vi "Maintenance4Ch.vi"() -> ()   [LabVIEW 2020]
doc: "Maintanence VI for FLS imaging system.\n[Covers: REQ9]\n[Covers: REQ10]"
uses:
  SubVI/DigitizerConfiguration/FLImDAQ.ctl
  <instrlib>/niScope/Controls/niScope trigger source.ctl
  SubVI/LabJack/LJ Pin Setting.ctl
  <vilib>/addons/control/pid/autopid.llb/PID autotuning parameters.ctl
  LaguerreDeconLib/DeconEngineClass/LaguerreDeconEngineClass.lvclass/LaguerreDeconEngineClass.ctl
  <vilib>/Utility/error.llb/DialogType.ctl
  <vilib>/event_ctls.llb/usereventprio.ctl
  <vilib>/Utility/miscctls.llb/LVRowAndColumnTypeDef.ctl
  <vilib>/Utility/miscctls.llb/LVMinMaxIncTypeDef.ctl
  SubVI/APD/APDClass.lvclass
  SubVI/APD/GainData.ctl
  SubVI/APD/iRFData.ctl
  <vilib>/Analysis/baseanly.llb/Mean (DBL).vi
  SubVI/GlobalVariables.vi
  <vilib>/addons/control/pid/autopid.llb/PID Online Autotuning (Step Closed Loop).vi
  <vilib>/addons/control/pid/pid.llb/PID Advanced (DBL).vi
  <instrlib>/niScope/Acquire/Fetch/niScope Multi Fetch Binary 16.vi
  <vilib>/Instr/_visa.llb/VISA Configure Serial Port (Instr).vi
  <userlib>/_OpenG.lib/file/file.llb/openg_file.lvlib
  <userlib>/_OpenG.lib/time/time.llb/openg_time.lvlib
  <vilib>/Analysis/NI_AALBase.lvlib
  LaguerreDeconLib/DeconEngineClass/LaguerreDeconEngineClass.lvclass
  <vilib>/Utility/miscctls.llb/LVPointTypeDef.ctl
  <vilib>/addons/control/pid/NI_PID_autopid.lvlib
  <vilib>/addons/control/pid/NI_PID_pid.lvlib
panel:
  in  "Duty Cycle (%)":u32=50
  in  "AB Rep Rate":u16 caption="Rep Rate" max=1000 step=1 format="%.0dHz"
  in  "Current":dbl=1.0 min=1.0 max=63.0 step=1.0 format="%#.1fA"
  out "GainIndicator":dbl caption="Gain"
  out "Noise\n(std of DC)":dbl format="%0.6f"
  in  "BG flag?":bool
  out "DC":dbl format="%0.2f"
  out "Amplitude":dbl
  in  "Gain High":dbl max=4.5
  in  "Gain low":dbl=3.0
  in  "Step":dbl=0.1
  in  "Num WF to acquire":u64=18446744073709551615
  in  "Channel":enum32{"Ch1", "Ch2", "Ch3", "Ch4"}(radio)
  in  "Task":enum32{"iRFAndGain", "Alignment"}(radio)
  in  "Aiming beam toggle":bool caption="445nm 15Hz"
  in  "Laser Rep Rate":u16=120 caption="Rep Rate" min=5 max=4000 step=1 format="%.0dHz"
  in  "355nm Laser toggle":bool caption="355nm 460Hz"
  out "appended path":path
  out "Current State":string
  out "WF max value":dbl
  out "Disclamer":picture
  out "Calibration #":i8
  out "BG #":i8
  in  "TCP Connect":bool
  out "Help":string
  in  "Auto gain":bool=TRUE
  out "Run #":i8
  in  "StopButton":bool caption="Stop"
  out "System Status:":bool
  in  "StartButton":bool caption="Start"
  in  "Ctrl V":dbl=0.05 min=0.0 max=5.5 step=0.1 format="%#.3f"
  out "System Hardware Connection Status":T1
  out "Waveform (no average)":dbl[](graph)
  in  "Tab Control":T2(tab)
  out "Ch1 Max CtrlV":dbl
  out "Ch1 iRF Graph":dbl[][](graph)
  out "Ch1 Gain":cluster{"CtrlV":dbl[], "Gain":dbl[]}(graph)
  out "Serial Number Ch1":string caption="Serial Number"
  out "DateTimeCh1":string caption="DateTime"
  out "Ch2 Gain":cluster{"CtrlV":dbl[], "Gain":dbl[]}(graph)
  out "Ch2 iRF Graph":dbl[][](graph)
  out "Ch2 Max CtrlV":dbl
  out "Serial Number Ch2":string caption="Serial Number"
  out "DateTimeCh2":string caption="DateTime"
  out "Ch3 iRF Graph":dbl[][](graph)
  out "Ch3 Gain":cluster{"CtrlV":dbl[], "Gain":dbl[]}(graph)
  out "Serial Number Ch3":string caption="Serial Number"
  out "Ch3 Max CtrlV":dbl
  out "DateTimeCh3":string caption="DateTime"
  out "Ch4 iRF Graph":dbl[][](graph)
  out "Ch4 Gain":cluster{"CtrlV":dbl[], "Gain":dbl[]}(graph)
  out "Serial Number Ch4":string caption="Serial Number"
  out "Ch4 Max CtrlV":dbl
  out "DateTimeCh4":string caption="DateTime"
  out "display loop timing(ms)":u32
  out "Aquisition loop timing(ms)":u32
  out "DisplayLoop":i32
  out "processing loop":i32
  out "processing loop timing(ms)":dbl
  out "laser EM lamp V":dbl format="%0.6f"
  out "aquisition loop Error Out":errorcluster
  out "Aq Loop?":bool
  out "processing Error Out":errorcluster
  out "Triggering:Trigger Delay":dbl
  out "Foot Pedal":bool
  out "LJ Pinout":T3={"Ch1 Bias"="DAC0", "Ch2 Bias"="DAC1", "Ch3 Bias"="DAC2", "Ch4 Bias"="DAC0", "355 PWM"="FIO0", "AimingBeam PWM"="FIO2", "Laser Ready"="FIO3", "Interlock"="FIO1", "Laser Start/Stop"="FIO1", "Red LED"="FIO1", "Green LED"="DIO3", "Foot Pedal"="DIO15"}
  out "FLImDAQ":T4={"Digitizer 1"="", "Digitizer 2"="", "Channel"=enum."Channel 0", "trigger source"="VAL_EXTERNAL", "trigger level"=0.5, "trigger delay"=1.35e-07, "min sample rate"=12500000000.0, "min record length"=2500, "vertical range"=1.0, "vertical offset"=-0.25, "Waveform to Avg"=2000} caption="FLIm DAQ Configuration" {"trigger delay" format="%^#.4e"; "trigger level" min=0.0 max=3.5 step=0.5 format="%.2f"; "vertical offset" format="%.4f"; "vertical range" format="%.2f"; "min sample rate" format="%#.2p"}
  out "Dig1 Temp":dbl
  out "Dig2 Temp":dbl
  in  "Sys Reconfig":bool
  out "Fetch Record #":i32
  out "Record Backlog":i32
  out "Fetch:Records Done":i32
  out "dt (s)":dbl format="%#_6p"
  out "Fetch:Records Done 2":i32
  in  "SaveData?":bool
  out "data Size":i32[](array[numeric])
  out "numWFInQ":i32
  in  "Clear WF Chart History":bool
  out "Waveform Chart":dbl(graph)
  in  "SaveiRFData":bool
  out "iRFDataTable":string[][](table)
  in  "SetIRFCtrlV":bool
  in  "ClearIRFData":bool
  in  "AcquireIRF":bool
  out "iRFInstSting":string="To aquire gain data, please start data aquisition! \nPlace blue (Ch1&2) or Green(Ch3) Chroma slide as close as possible to the fiber port! \nPlease remove channel 3 bandpass filter as well!"
  out "iRFSigInRange":bool caption="Signal  In Range?"
  out "Current iRF":dbl[](graph)
  out "iRFCtrlV":dbl[](array[numeric])
  in  "SaveGainData":bool
  out "GainInstSting":string="To aquire gain data, please start data aquisition! \nPlace blue (Ch1&2) or Green(Ch3) Chroma slide as close as possible to the fiber port! \nPlease remove channel 3 bandpass filter as well!"
  in  "ClearGainData":bool
  out "Gain":dbl[](array[numeric])
  in  "ComputeGain":bool
  out "Int Corr AUC":dbl[](array[numeric])
  out "AUC Std":dbl[](array[numeric])
  out "GainSigInRange":bool caption="Signal  In Range?"
  in  "AcquireGain":bool
  out "GainDataTable":string[][](table)
  out "Intensity Factor":dbl[](array[numeric])
  out "AUC":dbl[](array[numeric])
  out "Ctrl V":dbl[](array[numeric])
  out "XY Graph":cluster{"Ctrl V":dbl[], dbl[]}(graph)
  in  "Ch4 PID gains":T6={"proportional gain (Kc)"=0.5, "integral time (Ti, min)"=0.0003, "derivative time (Td, min)"=1e-05} {"derivative time (Td, min)" format="%.6f"; "integral time (Ti, min)" format="%.6f"; "proportional gain (Kc)" format="%.6f"}
  in  "Save PID":bool
  out "Targer and Max":cluster{"V target(1.0)":dbl, dbl}(graph)
  out "Completed?":bool
  out "Gain(Log10)":dbl(graph)
  in  "Gain(Log)":dbl=1.0
  in  "Ch1 PID gains":T6={"proportional gain (Kc)"=0.5, "integral time (Ti, min)"=0.0003, "derivative time (Td, min)"=1e-05} {"derivative time (Td, min)" format="%.6f"; "integral time (Ti, min)" format="%.6f"; "proportional gain (Kc)" format="%.6f"}
  in  "autotune? (F)":bool
  in  "PID dt (s)":dbl=-1.0
  out "dt out (s)":dbl format="%.3f"
  in  "V target(1.0)":dbl=1.0 format="%#_2f"
  in  "Accept?":bool
  out "tuned PID gains":T6={"proportional gain (Kc)"=1.0, "integral time (Ti, min)"=0.01, "derivative time (Td, min)"=0.0} {"derivative time (Td, min)" format="%_6f"; "integral time (Ti, min)" format="%.6f"; "proportional gain (Kc)" format="%.6f"}
  in  "autotuning parameters":T7={"type of controller"=2, "relay cycles"=100, "relay amplitude"=0.25, "control specifications"=1, "PV noise level"=0.01} {"PV noise level" format="%.5f"; "control specifications" items=["normal", "fast", "slow"]; "relay amplitude" format="%.2f"; "type of controller" items=["P", "PI", "PID"]}
  in  "Ch2 PID gains":T6={"proportional gain (Kc)"=0.5, "integral time (Ti, min)"=0.0003, "derivative time (Td, min)"=1e-05} {"derivative time (Td, min)" format="%.6f"; "integral time (Ti, min)" format="%.6f"; "proportional gain (Kc)" format="%.6f"}
  in  "Ch3 PID gains":T6={"proportional gain (Kc)"=0.5, "integral time (Ti, min)"=0.0003, "derivative time (Td, min)"=1e-05} {"derivative time (Td, min)" format="%.6f"; "integral time (Ti, min)" format="%.6f"; "proportional gain (Kc)" format="%.6f"}
  in  "gamma":dbl=1.0 format="%.2f"
  in  "alpha":dbl=nan format="%.2f"
  in  "Quit":bool
  # "440nm Laser Setting"
  # "355nm Laser Setting"
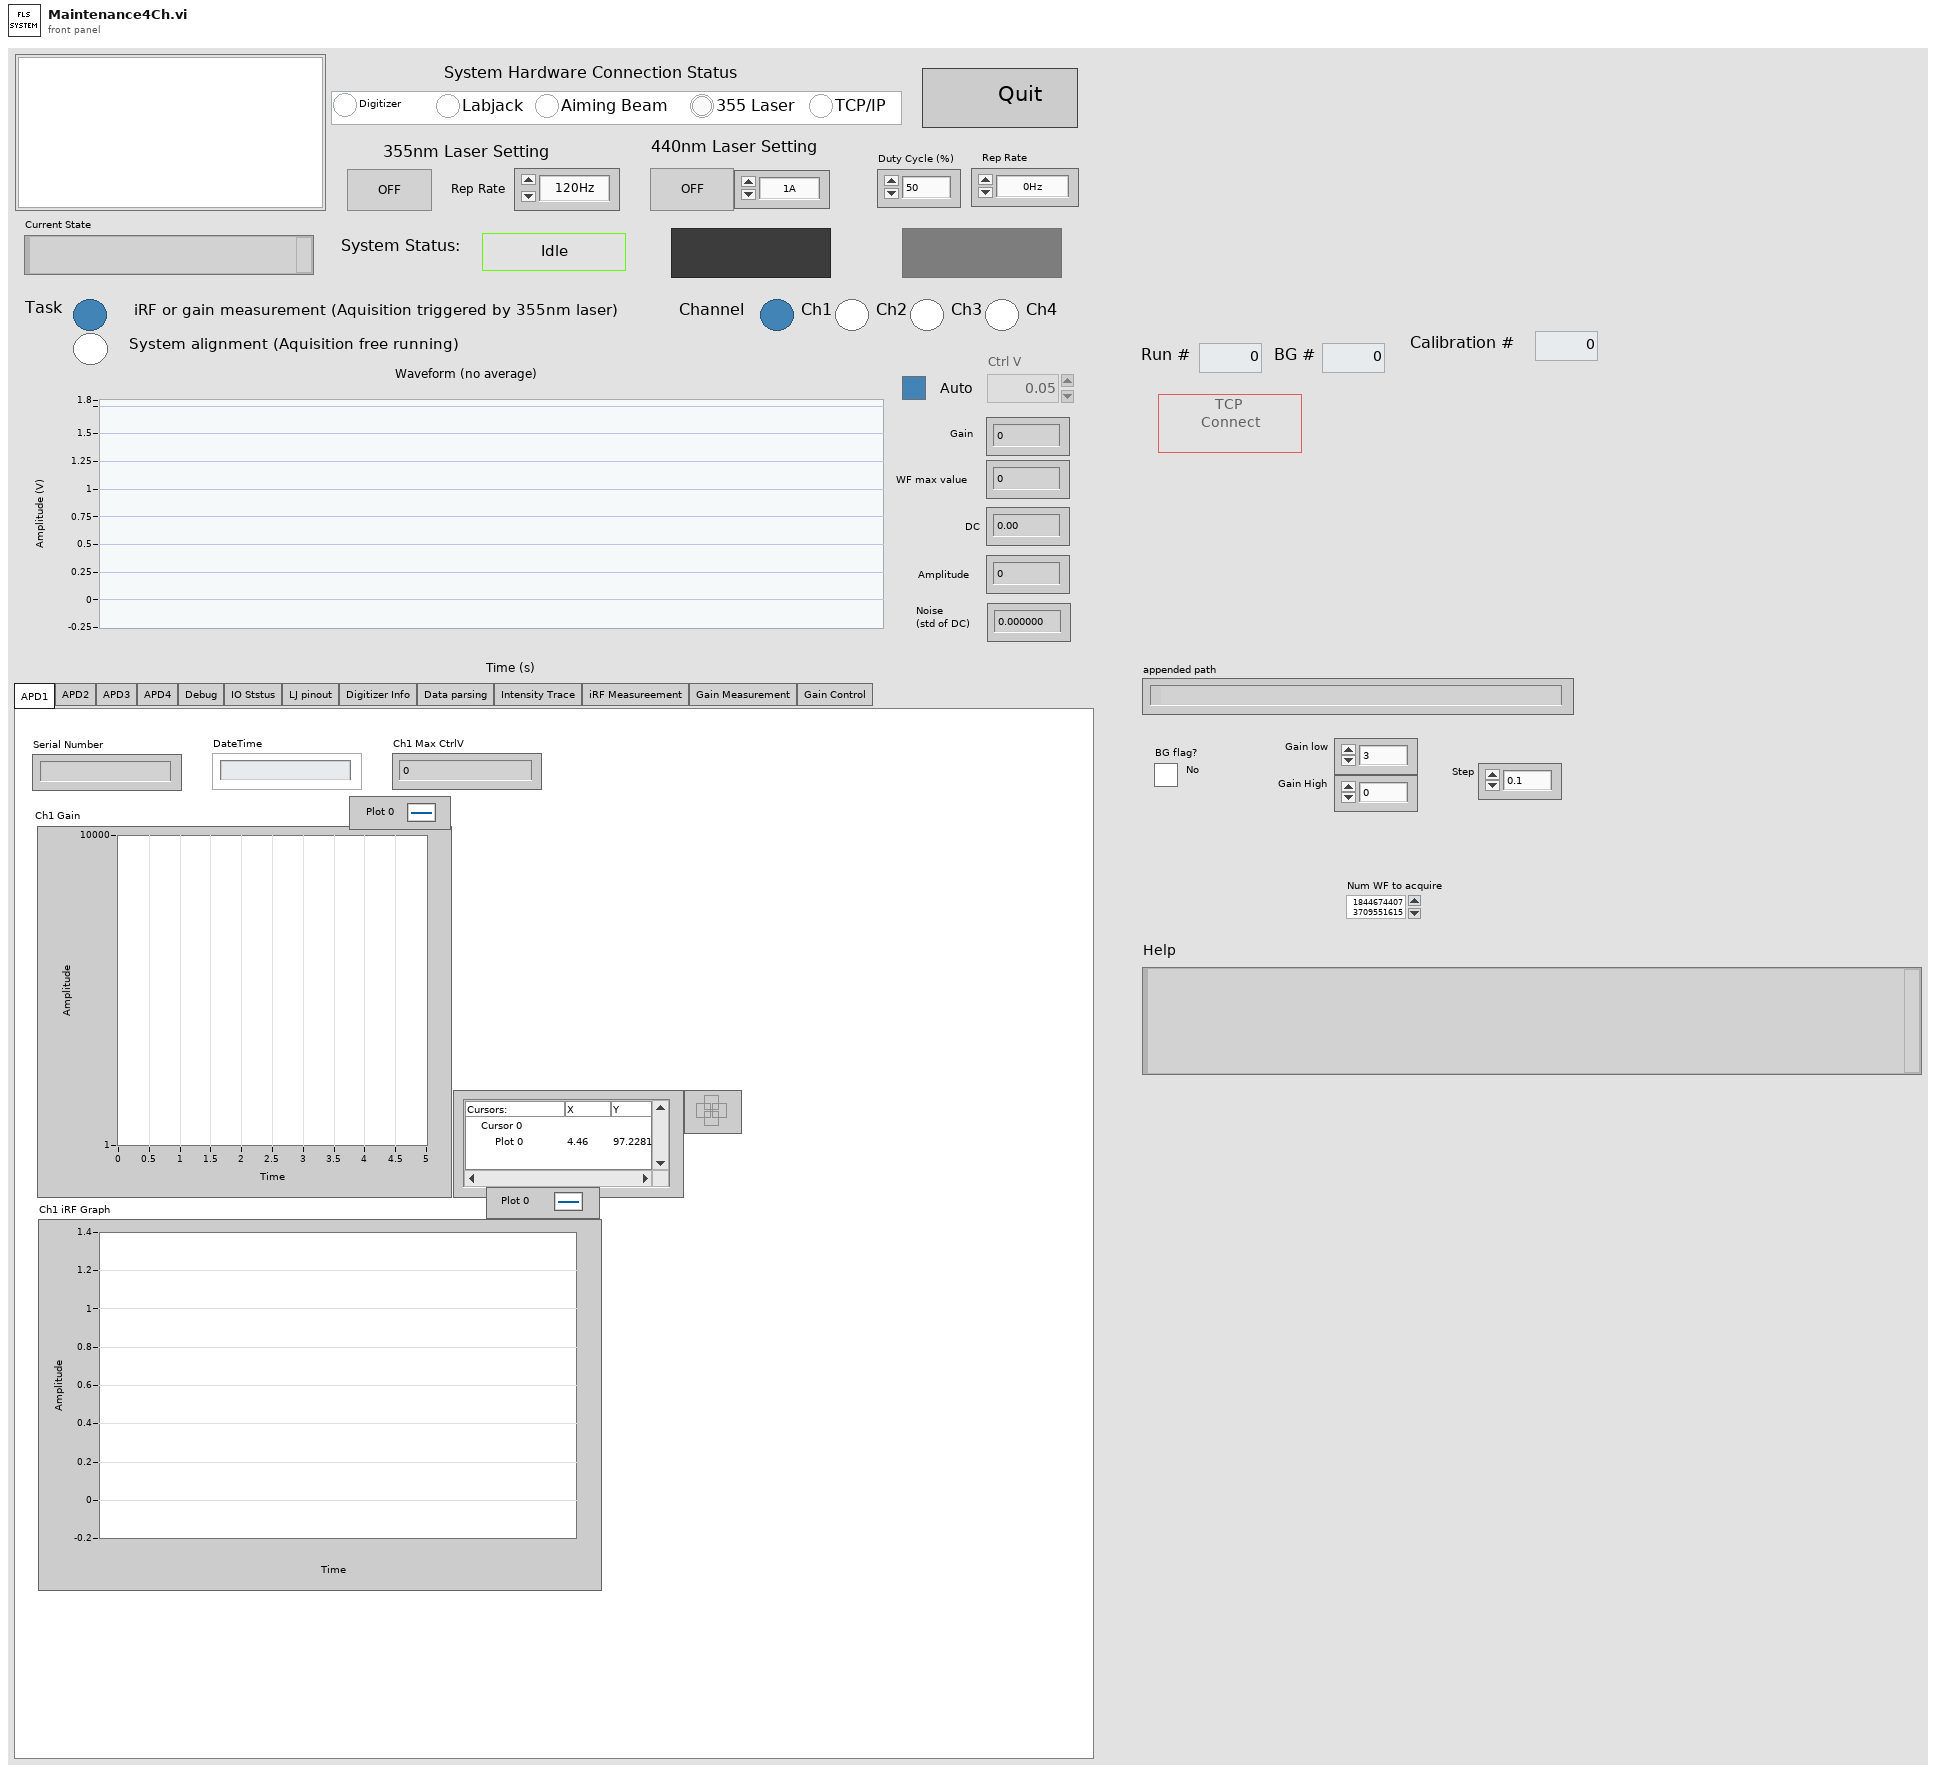
[diagram p1: front panel]
types:
  T1 = cluster{"Digitizer":bool, "Labjack":bool, "Aiming Beam":bool, "355 Laser":bool, "TCP/IP":bool}
  T2 = enum32{"APD1", "APD2", "APD3", "APD4", "Debug", "IO Ststus", "LJ pinout", "Digitizer Info", "Data parsing", "Intensity Trace", "iRF Measureement", "Gain Measurement", "Gain Control"}
  T3 = typedef "LJ Pin Setting.ctl" = cluster{"Ch1 Bias":string, "Ch2 Bias":string, "Ch3 Bias":string, "Ch4 Bias":string, "355 PWM":string, "AimingBeam PWM":string, "Laser Ready":string, "Interlock":string, "Laser Start/Stop":string, "Red LED":string, "Green LED":string, "Foot Pedal":string}
  T4 = typedef "FLImDAQ.ctl" = cluster{"Digitizer 1":refnum<k15>, "Digitizer 2":refnum<k15>, "Channel":enum16{"Channel 0", "Channel 1", "Channel 0&1"}, "trigger source":T5, "trigger level":dbl, "trigger delay":dbl, "min sample rate":dbl, "min record length":i32, "vertical range":dbl, "vertical offset":dbl, "Waveform to Avg":i16}
  T5 = typedef "niScope trigger source.ctl" = string
  T6 = cluster{"proportional gain (Kc)":dbl, "integral time (Ti, min)":dbl, "derivative time (Td, min)":dbl}
  T7 = typedef "PID autotuning parameters.ctl" = cluster{"type of controller":u16, "relay cycles":i32, "relay amplitude":dbl, "control specifications":u16, "PV noise level":dbl}
  T8 = cluster{"CtrlV":dbl, "WFs":dbl[][], "WFavg":dbl[]}
  T9 = enum16{"open", "replace", "create", "open or create", "replace or create", "replace or create with confirmation"}
  T10 = typedef "LVPointTypeDef.ctl" = cluster{"Horizontal":i16, "Vertical":i16}
  T11 = enum8{"Enabled", "Disabled", "Disabled and Grayed Out"}
  T12 = cluster{"CtrlV":dbl, "PeakV":dbl, "PeakV Std":dbl, "IntFactor":dbl, "IntCorrPeakV":dbl}
  T13 = enum16{"open", "open or create", "create or replace", "create", "open (read-only)"}
  T14 = enum32{"Invalid", "Standard", "Closed", "Hidden", "Minimized", "Maximized"}
  T15 = enum32{"invalid app kind", "Development System", "Run Time System", "Student Edition", "Embedded LabVIEW", "Evaluation", "Custom"}
  T16 = typedef "usereventprio.ctl" = enum32{"high priority", "normal priority"}
  T17 = enum32{"APD1", "APD2", "APD3", "Debug", "IO Ststus", "LJ pinout", "Digitizer Info", "Data parsing"}
  T18 = enum32{"Bad", "Idle", "Run top level", "Running"}
  T19 = typedef "LVRowAndColumnTypeDef.ctl" = cluster{"Row":i32, "Column":i32}
  T20 = typedef "LVMinMaxIncTypeDef.ctl" = cluster{"Minimum":dbl, "Maximum":dbl, "Increment":dbl}
  T21 = cluster{"Aiming Beam COM Port":refnum<visa-resource-name>, "Min Current":dbl, "Max Current":dbl, "Default Current":dbl, "Frequency(Hz)":i32}
  T22 = cluster{"Core":cluster{"Current VI Reference":refnum<vi>, "Close Panel on Exit?":bool}, "SysConfigCluster":cluster{"Ch1Enable?":bool, "Ch2Enable?":bool, "Ch3Enable?":bool, "Ch1AutoGain?":bool, "Ch2AutoGain?":bool, "Ch3AutoGain?":bool, "AimingBeamEnable?":bool}, "System Status":cluster{"Digitizer":bool, "Labjack":bool, "Aiming Beam":bool, "355 Laser":bool, "TCP/IP":bool}, "IDs":cluster{"RunID":i8, "BG ID":i8, "Cali ID":i8}, "DefaultPath":path, "Pathes":cluster{"DataPath":path, "BG Path":path, "iRFPath":path, "CaliPath":path}, "FLImDAQ":cluster{"resource name":refnum<k15>, "resource name 2":refnum<k15>, "Channel":enum16{"Channel 0", "Channel 1", "Channel 0&1"}, "trigger source":T5, "trigger level":dbl, "trigger delay":dbl, "min sample rate":dbl, "min record length":i32, "vertical range":dbl, "vertical offset":dbl, "Waveform to Avg":i32}, "SysRunning?":bool, "AB Cluster":cluster{"Aiming Beam COM Port":refnum<visa-resource-name>, "Min Current":dbl, "Max Current":dbl, "Default Current":dbl, "Frequency(Hz)":i32}, "LJ Pinout":T3, "355 PWM setting":cluster{"DIO_EF_CLOCK1_DIVISOR":i16, "DIO_EF_CLOCK1_ROLL_VALUE":i32, "DIO#_EF_INDEX":i16, "DIO#_EF_OPTIONS":i16, "DIO#_EF_CONFIG_A":i32}, "AB PWM setting":cluster{"DIO_EF_CLOCK1_DIVISOR":i16, "DIO_EF_CLOCK1_ROLL_VALUE":i32, "DIO#_EF_INDEX":i16, "DIO#_EF_OPTIONS":i16, "DIO#_EF_CONFIG_A":i32}, "Last Trigger":u32, "niTClk sessions":refnum<k20>[], "Laser start tic":u32, "TCP attempt count":i32, "iRFAllGain":dbl[][], "SlowTimer":u32, "FastTimer":u32, "TempPath":path, "LED vi reference":refnum<vi>, "APDSerials":cluster{"Ch1Serial":string, "Ch2Serial":string, "Ch3Serial":string, "Ch4Serial":string}, "LedViRefOpen":bool, "GainBGRaw":dbl[][], "GainDataTemp":cluster{"CtrlV":dbl, "AUC":dbl, "AUC Std":dbl, "IntFactor":dbl, "IntCorrAUC":dbl}, "iRFIdx":i32}
  T23 = cluster{"CtrlV":dbl, "AUC":dbl, "AUC Std":dbl, "IntFactor":dbl, "IntCorrAUC":dbl}
  T24 = cluster{"Ch1Serial":string, "Ch2Serial":string, "Ch3Serial":string, "Ch4Serial":string}
  T25 = cluster{"DataPath":path, "BG Path":path, "iRFPath":path, "CaliPath":path}
  T26 = cluster{"DIO_EF_CLOCK1_DIVISOR":i16, "DIO_EF_CLOCK1_ROLL_VALUE":i32, "DIO#_EF_INDEX":i16, "DIO#_EF_OPTIONS":i16, "DIO#_EF_CONFIG_A":i32}
  T27 = cluster{"resource name":refnum<k15>, "resource name 2":refnum<k15>, "Channel":enum16{"Channel 0", "Channel 1", "Channel 0&1"}, "trigger source":T5, "trigger level":dbl, "trigger delay":dbl, "min sample rate":dbl, "min record length":i32, "vertical range":dbl, "vertical offset":dbl, "Waveform to Avg":i32}
  T28 = cluster{"Ch1Enable?":bool, "Ch2Enable?":bool, "Ch3Enable?":bool, "Ch1AutoGain?":bool, "Ch2AutoGain?":bool, "Ch3AutoGain?":bool, "AimingBeamEnable?":bool}
  T29 = cluster{"Current VI Reference":refnum<vi>, "Close Panel on Exit?":bool}
  T30 = cluster{"iRF":dbl[], "iRF":dbl[], "iRF":dbl[], "iRF":dbl[]}
  T31 = typedef "DialogType.ctl" = u16
  T32 = typedef "LJ PWM Setting.ctl" = cluster{"DIO_EF_CLOCK1_DIVISOR":i16, "DIO_EF_CLOCK1_ROLL_VALUE":i32, "DIO#_EF_INDEX":i16, "DIO#_EF_OPTIONS":i16, "DIO#_EF_CONFIG_A":i32}
  T33 = typedef "AimingBeam.ctl" = cluster{"Aiming Beam COM Port":refnum<visa-resource-name>, "Min Current":dbl, "Max Current":dbl, "Default Current":dbl, "Frequency(Hz)":u32}
  T34 = typedef "LVBoundsTypeDef.ctl" = cluster{"Width":u32, "Height":u32}
  T35 = typedef "imagedata.ctl" = cluster{"image type":i32, "image depth":i32, "image":u8[], "mask":u8[], "colors":u32[], "Rectangle":cluster{"left":i16, "top":i16, "right":i16, "bottom":i16}}
  T36 = typedef "LVCursorListTypeDef.ctl" = cluster{"Name":string, "Color":u32, "Style":u8, "Point Style":u8, "Name Visible":bool, "Allow Drag":bool, "Cursor Mode":u32, "Plot":i32, "Index":i32, "Position":cluster{"X":dbl, "Y":dbl}, "X Scale":u32, "Y Scale":u32, "Watch Plots":i32[], "Watch All Plots":bool, "Plot Area":i32, "Label Offset":cluster{"X":dbl, "Y":dbl}}[]
  T37 = cluster{"Name":string, "Color":u32, "Style":u8, "Point Style":u8, "Name Visible":bool, "Allow Drag":bool, "Cursor Mode":u32, "Plot":i32, "Index":i32, "Position":cluster{"X":dbl, "Y":dbl}, "X Scale":u32, "Y Scale":u32, "Watch Plots":i32[], "Watch All Plots":bool, "Plot Area":i32, "Label Offset":cluster{"X":dbl, "Y":dbl}}
  T38 = cluster{"Name":string, "Color":u32, "Style":u8, "Point Style":u8, "Name Visible":bool, "Allow Drag":bool, "Cursor Mode":u32, "Plot":i32, "Index":i32, "Position":cluster{"X":dbl, "Y":dbl}, "X Scale":u32, "Y Scale":u32, "Watch Plots":i32[], "Watch All Plots":bool, "Plot Area":i32, "Label Offset":cluster{"X":dbl, "Y":dbl}}[]
  T39 = cluster{"Ch1APDSerial#":string, "Ch2APDSerial#":string, "Ch3APDSerial#":string, "Ch4APDSerial#":string}
  T40 = typedef "GainData.ctl" = cluster{"CtrlV":dbl[], "NumOfWFs":i32, "WF length":i32, "Gain":dbl[], "GainRaw":dbl[][], "GainBGRaw":dbl[][]}
  T41 = typedef "iRFData.ctl" = cluster{"dt":dbl, "NumOfWFs":i32, "WFLength":i32, "iRFCtrlV":dbl[], "iRFWFsAvg":dbl[][], "iRFRaw":dbl[][]}
  T42 = cluster{"CtrlV":dbl, "WFs":dbl[][], "WFavg":dbl[]}[]
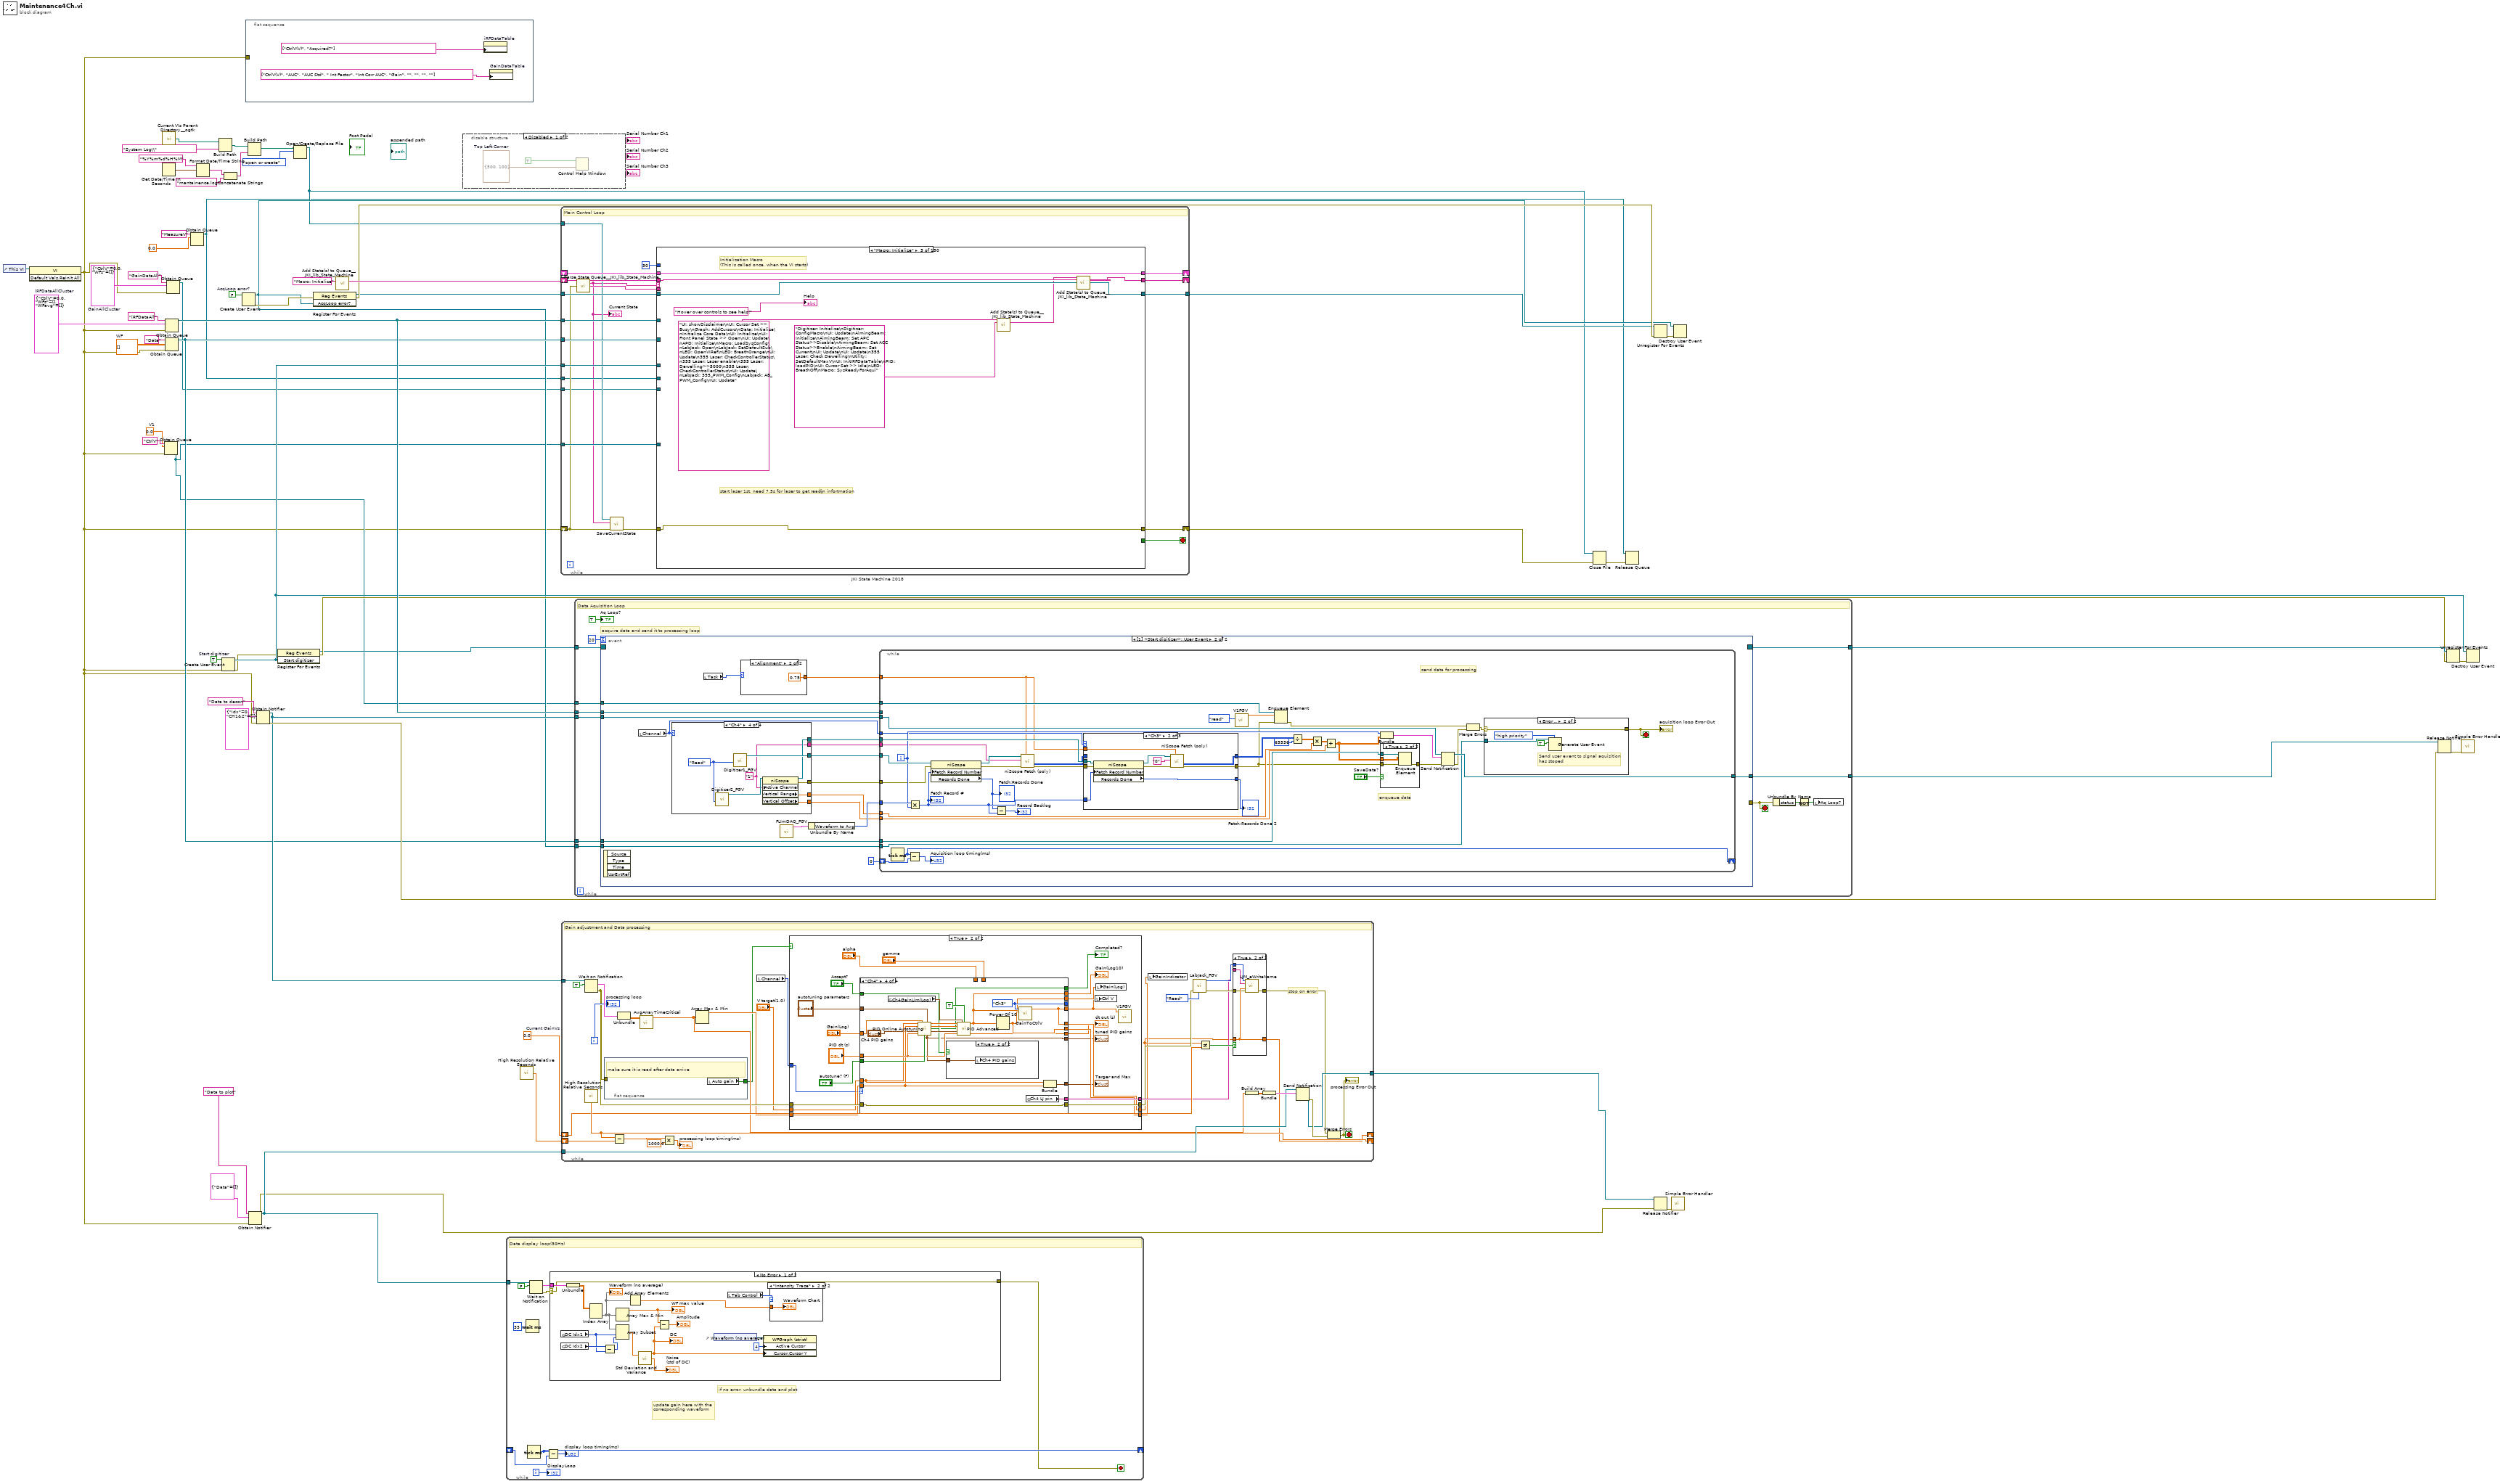
[diagram p0: block diagram]
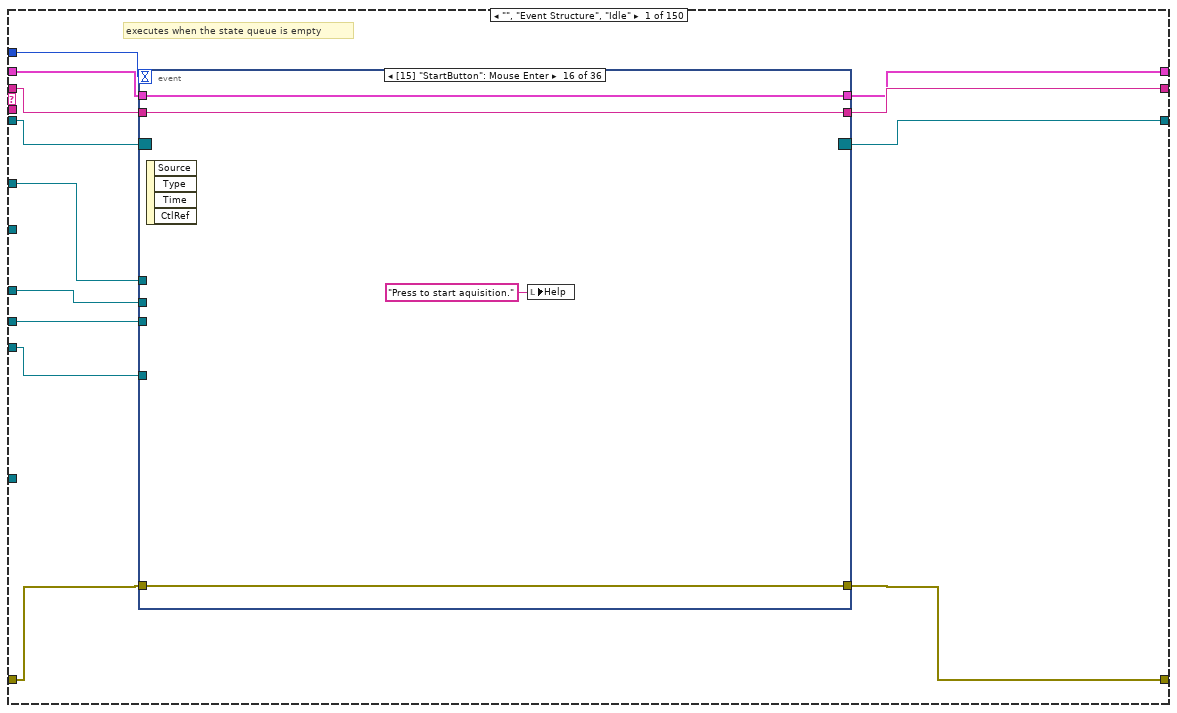
[diagram p3: hidden frame]
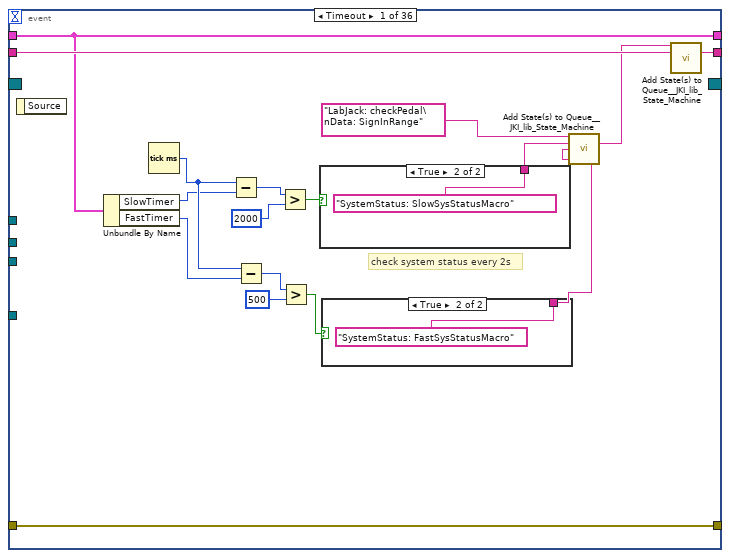
[diagram p4: hidden frame]
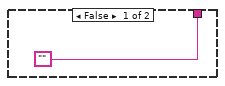
[diagram p5: hidden frame]
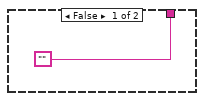
[diagram p6: hidden frame]
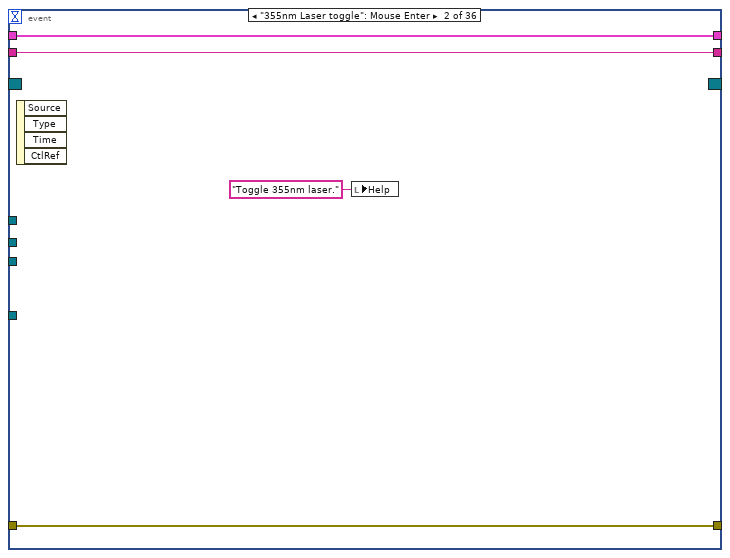
[diagram p7: hidden frame]
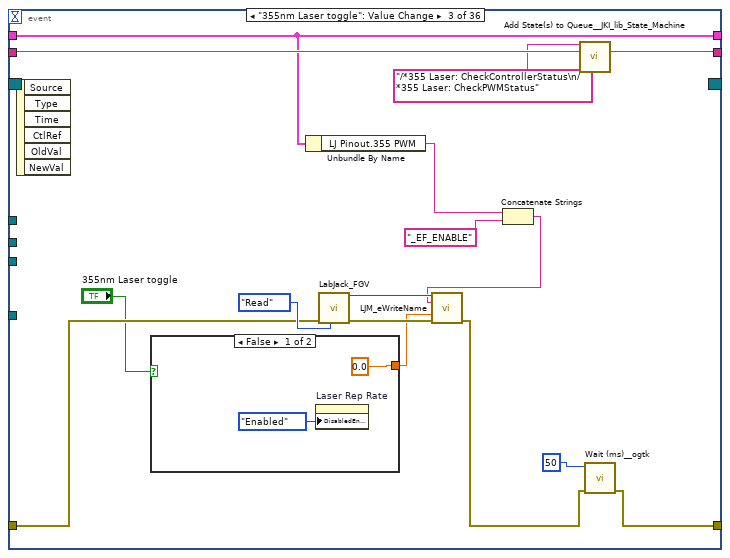
[diagram p8: hidden frame]
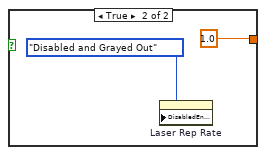
[diagram p9: hidden frame]
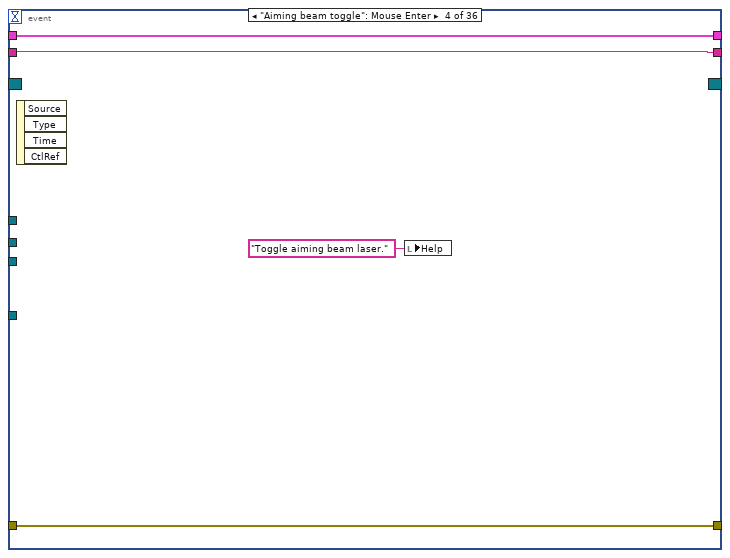
[diagram p10: hidden frame]
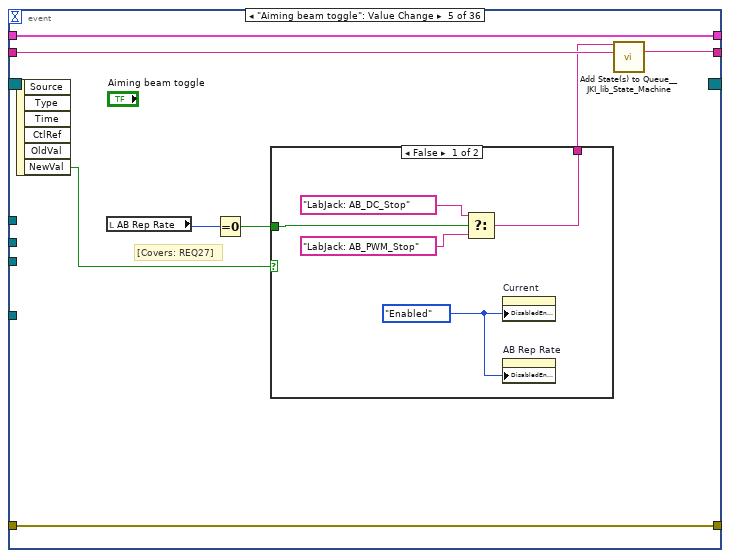
[diagram p11: hidden frame]
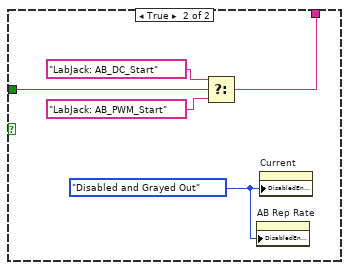
[diagram p12: hidden frame]
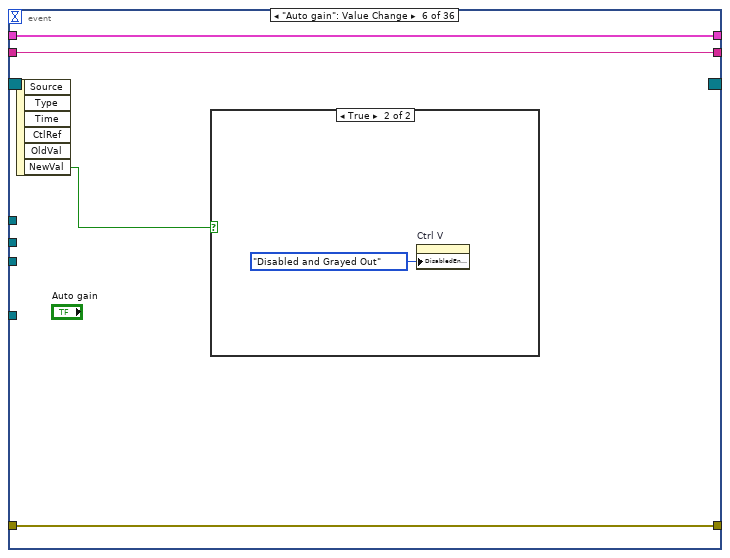
[diagram p13: hidden frame]
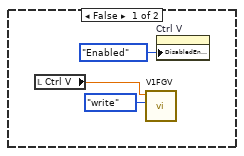
[diagram p14: hidden frame]
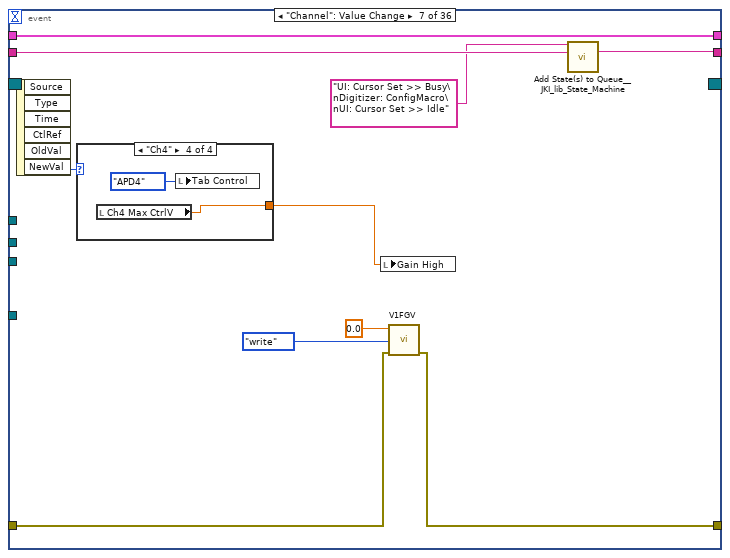
[diagram p15: hidden frame]
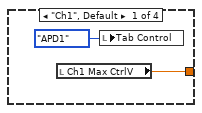
[diagram p16: hidden frame]
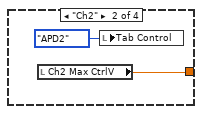
[diagram p17: hidden frame]
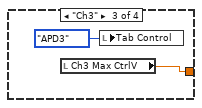
[diagram p18: hidden frame]
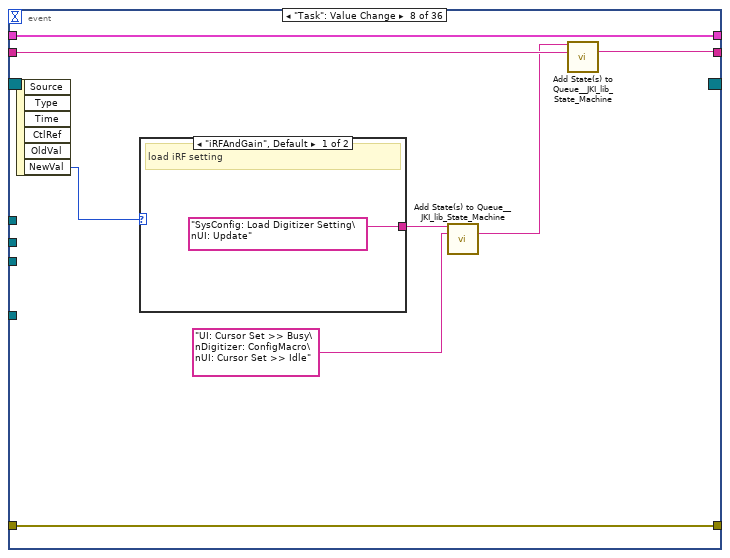
[diagram p19: hidden frame]
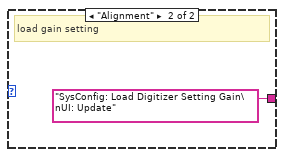
[diagram p20: hidden frame]
diagram:
  w3 = cluster{"CtrlV":dbl, "WFs":dbl[][]} {"CtrlV"=0.0, "WFs"=[]}  # GainAllCluster
  w5 = T8 {"CtrlV"=0.0, "WFs"=[], "WFavg"=[]}  # iRFDataAllCluster
  w22 = 0.0  # V1
  w26 = 0.0  # Current GainVs
  w43 = FALSE  # AcqLoop error?
  w53 = TRUE  # Start digitizer
  w56 = dbl[][] []  # WF
  n1 = control-ref of="This VI"() -> (w58:refnum<vi>)
  n2 = invoke on="Invoke Node" class="VI" method="Default Vals.Reinit All"(reference=w58) -> (error out=w1:errorcluster)  [unwired: 2 in, 2 out]
  n3 = call <userlib>:"Current VIs Parent Directory__ogtk.vi"() -> ("Parent Directory (+ Relative)"=w21:path)  [unwired: 5 in]
  n4 = Get Date/Time In Seconds() -> (seconds since 1Jan1904=w19:timestamp)
  n5 = Obtain Queue(name (unnamed)="CtrlV", element data type=w22, error in (no error)=w1) -> (queue out=w24:refnum<queue>)  [unwired: 2 in, 2 out]
  n6 = Obtain Queue(name (unnamed)="Data", element data type=w56, error in (no error)=w1) -> (queue out=w32:refnum<queue>)  [unwired: 2 in, 2 out]
  n7 = Obtain Queue(name (unnamed)="iRFDataAll", element data type=w5, error in (no error)=w1) -> (queue out=w54:refnum<queue>)  [unwired: 2 in, 2 out]
  n8 = Obtain Queue(name (unnamed)="GainDataAll", element data type=w3, error in (no error)=w1) -> (queue out=w2:refnum<queue>)  [unwired: 2 in, 2 out]
  n9 = Obtain Queue(name (unnamed)="MeasureV", element data type=0.0) -> (queue out=w6:refnum<queue>)  [unwired: 3 in, 2 out]
  n10 = Format Date/Time String(time format string (%c)="%Y%m%d%H%M", seconds (now)=w19) -> (date/time string=w16:string)  [unwired: 1 in]
  n11 = Build Path(base path=w21, name or relative path="System Log\\") -> (appended path=w12:path)
  n12 = Create User Event(user event datatype=w53, error in=w1) -> (user event=w42:refnum<user-event>, error out=w28:errorcluster)
  n13 = Concatenate Strings(w16, "mantainence.log" ("string")) -> (w14:string)
  n14 = Create User Event(user event datatype=w43) -> (user event=w27:refnum<user-event>, error out=w29:errorcluster)  [unwired: 1 in]
  n15 = flat-sequence {
    tunnel: w1 -> [_]
    frame #0 {
      n16 = property on="iRFDataTable" class="Tbl (strict)"("Column Headers[]"=string[] ["CtrlV(V)", "Acquired?"] ("Column Header Strings[]")) -> ()  [unwired: 2 in, 2 out]
      n17 = property on="GainDataTable" class="Tbl (strict)"("Column Headers[]"=string[] ["CtrlV(V)", "AUC", "AUC Std", " Int Factor", "Int Corr AUC", "Gain", "", "", "", ""] ("Column Header Strings[]")) -> ()  [unwired: 2 in, 2 out]
    }
  }
  n18 = Build Path(base path=w12, name or relative path=w14) -> (appended path=w17:path)
  n19 = Obtain Notifier(name (unnamed)="Data to plot", notification data type=cluster{"Data":dbl[][]} {"Data"=[]}, error in (no error)=w1) -> (notifier out=w36:refnum<notifier>, error out=w33:errorcluster)  [unwired: 1 in, 1 out]
  n20 = Obtain Notifier(name (unnamed)="Data to decon", notification data type=cluster{"idx":i32, "CH1&2":dbl[][]} {"idx"=0, "CH1&2"=[]}, error in (no error)=w1) -> (notifier out=w39:refnum<notifier>, error out=w47:errorcluster)  [unwired: 1 in, 1 out]
  n21 = register-events(error in=w28, w42) -> (reference out=w44:refnum<event-registration>, error out=w50:errorcluster)  [unwired: 1 in]
  n22 = Open/Create/Replace File(file path (use dialog)=w17, operation (0:open)=T9."open or create") -> (refnum out=w10:refnum<file>)  [unwired: 4 in, 2 out]
  n23 = register-events(error in=w29, w27) -> (reference out=w31:refnum<event-registration>, error out=w40:errorcluster)  [unwired: 1 in]
  n24 = call <vilib>:"Add State(s) to Queue__JKI_lib_State_Machine.vi"("State(s) in (\"\")"="Macro: Initialize") -> ("States Out"=w60:string)  [unwired: 14 in]
  n25 = disable-structure "Diagram Disable Structure" shown="Disabled" {
    frame Disabled {
      w63 = T10 {"Horizontal"=500, "Vertical"=100}  # Top Left Corner
      n26 = Control Help Window(0:w63, 1:TRUE ("Show")) -> ()
    }
    frame Enabled {
    }
  }
  n27 = while {
    tunnel: w36 -> [w74]
    shift-right: [w68] -> _
    shift-left: _ -> [w72]
    i -> [w66]
    stop <- w65 stop-if-true
    # "if no error, unbundle data and plot"
    # "update gain here with the corresponding waveform"
    # "Data display loop(30Hz)"
    n28 = Wait (ms)(milliseconds to wait=u32 33) -> ()  [unwired: 1 out]
    n29 = Tick Count (ms)() -> (millisecond timer value=w68:u32)
    n30 = Wait on Notification(notifier=w74, ignore previous (F)=FALSE) -> (notification=w69:cluster{"Data":dbl[][]}, error out=w67:errorcluster)  [unwired: 2 in, 2 out]
    n31 = Subtract(x=w68, y=w72) -> (x-y=→"display loop timing(ms)":u32)
    n32 = case shown="No Error" w67 {
      selector: w67 -> [w83 w92]
      tunnel: w69 -> [w90 _]
      tunnel: [w83 w92] -> w65
      frame No Error {
        n33 = global read "GlobalVariables.vi" "DC Idx1"() -> (w76:i32)
        n34 = global read "GlobalVariables.vi" "DC Idx2"() -> (w77:i32)
        n35 = Unbundle(w90) -> ("Data"=w87:dbl[][])
        n36 = Index Array(array=w87) -> (element=w86:dbl[])  [unwired: 2 in]
        "Waveform (no average)" <- w86
        n37 = Subtract(x=w77, y=w76) -> (x-y=w75:i32)
        n38 = Array Max & Min(array=w86) -> (max value=w89:dbl)  [unwired: 3 out]
        "WF max value" <- w89
        n39 = Array Subset(array=w86, index=w76, length=w75) -> (w82:dbl[])
        n40 = Add Array Elements(numeric array=w86) -> (sum=w85:dbl)
        n41 = call <vilib>:"Std Deviation and Variance.vi"("X"=w82) -> ("mean"=w78:dbl, "standard deviation"=→"Noise\n(std of DC)":dbl)  [unwired: 1 in, 1 out]
        "DC" <- w78
        n42 = Subtract(x=w89, y=w78) -> (x-y=→"Amplitude":dbl)
        n43 = control-ref of="Waveform (no average)"() -> (w80:refnum<vi>)
        n44 = local read "Tab Control"() -> (w84:T2)
        n45 = property class="WFGraph (strict)"(reference=w80, "Active Cursor"=u32 4, "Cursor.Cursor Y"=w78) -> ()  [unwired: 1 in, 2 out]
        n46 = case shown="\"Intensity Trace\"" w84 {
          tunnel: w85 -> [_ w91]
          frame "APD1", Default {
          }
          frame "Intensity Trace" {
            "Waveform Chart" <- w91
          }
        }
      }
      frame Error {
      }
    }
    "DisplayLoop" <- w66
  }
  n47 = call <vilib>:"High Resolution Relative Seconds.vi"() -> ("relative seconds"=w23:dbl)
  n48 = while "JKI State Machine 2018" {
    shift-right: [w109] -> _
    shift-left: _ -> [w108]
    shift-right: [w99] -> w11
    shift-left: w1 -> [w98]
    shift-right: [w110] -> _
    shift-left: w60 -> [w111]
    tunnel: w54 -> [w106]
    tunnel: w32 -> [w105]
    tunnel: w42 -> [w104]
    tunnel: w31 -> [w103]
    tunnel: [w102] -> w30
    tunnel: w24 -> [w100]
    tunnel: w10 -> [w96]
    tunnel: w6 -> [w95]
    tunnel: w2 -> [w94]
    stop <- w101 stop-if-true
    # "Main Control Loop"
    n49 = call <vilib>:"Parse State Queue__JKI_lib_State_Machine.vi"("State Queue"=w111, "Error In (no error)"=w98) -> ("Remaining States"=w113:string, "Current State"=w93:string, "Arguments"=w112:string)  [unwired: 11 in]
    "Current State" <- w93
    n50 = call "SaveCurrentState.vi"("error in (no error)"=w98, "Current State"=w93, "Byte Stream File in"=w96) -> ("error out"=w97:errorcluster)  [unwired: 8 in]
    n51 = case shown="\"Macro: Initialize\"" w93 {
      selector: w93 -> [_ _ _ _ _ _ _ _ _ _ _ _ _ _ _ _ _ _ _ _ _ _ w832 _ _ _ _ _ _ _ _ _ _ _ _ _ _ _ _ _ _ _ _ _ _ _ _ _ _ _ _ _ _ _ _ _ _ _ _ _ _ _ _ _ _ _ _ _ _ _ _ _ _ _ _ _ _ _ _ _ _ _ _ _ _ _ _ _ _ _ _ _ _ _ _ _ _ _ _ _ _ _ _ _ _ _ _ _ _ _ _ _ _ _ _ _ _ _ _ _ _ _ _ _ _ _ _ _ _ _ _ _ _ _ _ _ _ _ _ _ _ _ _ _ _ _ _ _ _ _]
      tunnel: w113 -> [w126 w461 w470 w476 w483 w492 w503 w512 w537 w552 w583 w589 w614 w635 w652 w664 w695 w728 w783 w818 w825 w830 w836 w861 w869 w893 w898 w910 w919 w936 w944 w960 w976 w1000 w1005 w1015 w1040 w1068 w1091 w1135 w1187 w1218 w1241 w1266 w1298 w1321 w1370 w1385 w1401 w1406 w1417 w1428 w1444 w1482 w1499 w1513 w1547 w1558 w1564 w1575 w1587 w1618 w1650 w1663 w1676 w1690 w1704 w1709 w1721 w1733 w1746 w1759 w1775 w1803 w1818 w1823 w1832 w1870 w1883 w1891 w1899 w1913 w1918 w1924 w1941 w1958 w1975 w1995 w2020 w2029 w2034 w2042 w2050 w2055 w2064 w2103 w2143 w2148 w2171 w2184 w2202 w2208 w2219 w2232 w2250 w2257 w2269 w2334 w2345 w2358 w2383 w2406 w2412 w2418 w2433 w2478 w2486 w2492 w2497 w2503 w2511 w2520 w2530 w2536 w2542 w2547 w2553 w2566 w2600 w2609 w2621 w2632 w2686 w2708 w2714 w2739 w2764 w2789 w2814 w2831 w2894 w2952 w2971 w2981 w3004 w3009 w3031 w3040 w3049 w3054]
      tunnel: w112 -> [_ _ _ _ _ _ _ _ _ _ _ _ _ _ _ _ _ _ _ _ _ _ _ _ _ _ _ _ _ _ w943 w959 _ _ _ _ _ _ _ _ _ _ _ _ _ _ _ _ _ _ _ _ _ _ _ _ _ _ _ _ w1585 _ _ _ _ _ _ _ _ _ _ _ _ _ _ _ _ _ _ _ _ _ _ _ _ _ _ _ _ _ _ _ _ _ _ _ _ _ w2162 _ _ _ _ _ _ w2252 w2264 _ _ _ _ w2402 _ _ _ _ _ _ _ w2498 _ w2512 w2525 _ _ _ _ _ _ _ _ _ _ _ _ _ _ _ _ _ _ _ _ _ w2995 _ _ _ _ _]
      tunnel: w108 -> [w124 w458 w466 w473 w479 w486 w500 w510 w521 w549 _ w586 w608 w626 w649 w655 w692 w722 w765 w792 w819 w827 w834 w844 w866 w891 w895 w900 w912 w921 w937 w953 w972 w992 w1002 w1012 w1037 w1052 w1075 w1100 w1152 w1203 w1225 w1248 w1280 w1318 w1358 w1383 w1387 w1403 w1410 w1421 w1433 w1470 w1486 w1503 w1523 w1556 w1561 w1565 w1577 w1595 w1628 w1652 w1665 w1679 w1692 w1706 w1718 w1730 w1741 w1753 w1770 w1791 w1806 w1820 w1828 w1868 w1880 w1888 w1897 w1911 w1915 w1922 w1925 w1942 w1960 w1976 w2001 w2025 w2031 w2035 w2043 w2052 w2061 w2098 w2124 w2155 w2168 w2182 w2199 w2205 w2212 w2224 w2246 w2255 w2262 w2331 w2336 w2350 w2375 w2403 w2409 w2415 w2419 w2465 w2483 w2489 w2494 w2500 w2508 w2517 w2527 w2533 w2539 w2544 w2550 w2564 w2598 w2606 w2619 w2628 w2672 w2706 w2711 w2736 w2762 w2787 w2812 w2825 w2888 w2950 w2968 w2979 w2996 w3006 w3010 w3037 w3047 w3051]
      tunnel: [w123 w459 w468 w474 w481 w490 w501 w504 w535 w550 w581 w587 w604 w620 w650 w659 w693 w703 w771 w798 w822 w828 w838 w859 errorcluster {"status"=FALSE, "code"=0, "source"=""} ("error out") w890 w896 w905 w917 w928 w941 w957 w971 w994 w1003 w1013 w1035 w1060 w1083 w1126 w1178 w1210 w1233 w1259 w1291 w1313 w1360 w1373 w1391 w1404 w1407 w1418 w1438 w1471 w1493 w1506 w1527 w1550 w1562 w1573 w1579 w1600 w1632 w1655 w1668 w1680 w1696 w1707 w1711 w1723 w1742 w1754 w1764 w1793 w1808 w1821 w1825 w1863 w1881 w1889 w1894 w1908 w1916 w1919 w1930 w1947 w1970 w1990 w2015 w2023 w2032 w2040 w2048 w2053 w2062 w2101 w2141 w2156 w2169 w2181 w2200 w2206 w2217 w2230 w2248 w2253 w2266 w2332 w2342 w2354 w2378 w2404 w2410 w2416 w2424 w2470 w2484 w2490 w2495 w2501 w2509 w2518 w2528 w2534 w2540 w2545 w2551 w2559 w2595 w2607 w2616 w2622 w2671 w2692 w2712 w2726 w2740 w2766 w2790 w2826 w2890 w2944 w2969 w2975 w2998 w3007 w3011 w3038 w3045 w3052] -> w99
      tunnel: w97 -> [w122 w459 w468 w474 w481 w490 w501 w504 w535 w550 w581 w587 w609 w630 w650 w661 w693 w702 w770 w807 w823 w828 w837 w859 w862 w890 w896 w906 w916 w927 w940 w956 w973 w993 w1003 w1013 w1034 w1062 w1085 w1129 w1181 w1212 w1235 w1260 w1292 w1312 w1359 w1374 w1393 w1404 w1413 w1424 w1437 w1472 w1494 w1511 w1531 w1549 w1562 w1571 w1582 w1599 w1620 w1654 w1667 w1684 w1695 w1707 w1710 w1722 w1743 w1756 w1771 w1792 w1809 w1821 w1824 w1861 w1881 w1889 w1892 w1902 w1916 w1919 w1936 w1953 w1969 w1989 w2014 w2024 w2032 w2040 w2048 w2053 w2062 w2101 w2141 w2156 w2169 w2181 w2200 w2206 w2217 w2230 w2248 w2254 w2267 w2332 w2342 w2352 w2381 w2404 w2410 w2416 w2428 w2469 w2484 w2490 w2495 w2501 w2509 w2518 w2528 w2534 w2540 w2545 w2551 w2557 w2594 w2607 w2612 w2627 w2668 w2690 w2712 w2715 w2741 w2765 w2806 w2828 w2889 w2946 w2969 w2974 w2999 w3007 w3012 w3038 w3044 w3052]
      tunnel: [w125 w460 w469 w475 w482 w491 w502 w511 w536 w551 w582 w588 w613 w634 w651 w663 w694 w727 w782 w817 w824 w829 w835 w860 w868 w892 w897 w909 w918 w935 w944 w960 w975 w999 w1004 w1014 w1039 w1067 w1090 w1134 w1186 w1217 w1240 w1265 w1297 w1320 w1369 w1384 w1400 w1405 w1416 w1427 w1443 w1481 w1498 w1512 w1546 w1557 w1563 w1574 w1586 w1617 w1649 w1662 w1675 w1689 w1703 w1708 w1720 w1732 w1745 w1758 w1774 w1802 w1817 w1822 w1831 w1869 w1882 w1890 w1898 w1912 w1917 w1923 w1940 w1957 w1974 w1994 w2019 w2028 w2033 w2041 w2049 w2054 w2063 w2102 w2142 w2157 w2170 w2183 w2201 w2207 w2218 w2231 w2249 w2256 w2268 w2333 w2344 w2357 w2382 w2405 w2411 w2417 w2432 w2477 w2485 w2491 w2496 w2502 w2510 w2519 w2529 w2535 w2541 w2546 w2552 w2565 w2599 w2608 w2620 w2631 w2685 w2707 w2713 w2738 w2763 w2788 w2813 w2830 w2893 w2951 w2970 w2980 w3003 w3008 w3030 w3039 w3048 w3053] -> w110
      tunnel: [_ _ _ _ _ _ _ _ _ _ _ _ _ _ _ _ _ _ _ _ _ _ _ _ _ TRUE _ _ _ _ _ _ _ _ _ _ _ _ _ _ _ _ _ _ _ _ _ _ _ _ _ _ _ _ _ _ _ _ _ _ _ _ _ _ _ _ _ _ _ _ _ _ _ _ _ _ _ _ _ _ _ _ _ _ _ _ _ _ _ _ _ _ _ _ _ _ _ _ _ _ _ _ _ _ _ _ _ _ _ _ _ _ _ _ _ _ _ _ _ _ _ _ _ _ _ _ _ _ _ _ _ _ _ _ _ _ _ _ _ _ _ _ _ _ _ _ _ _ _ _] -> w101
      tunnel: [w121 w458 w466 w473 w479 w486 w500 w510 w521 w549 w559 w586 w608 w626 w649 w656 w692 w721 w766 w792 w819 w827 w834 w843 w866 w891 w895 w901 w911 w921 w937 w953 w972 w992 w1002 w1012 w1037 w1051 w1074 w1099 w1151 w1202 w1224 w1253 w1285 w1318 w1358 w1383 w1386 w1403 w1410 w1421 w1434 w1470 w1486 w1504 w1523 w1556 w1561 w1566 w1577 w1595 w1628 w1652 w1665 w1679 w1692 w1706 w1718 w1730 w1739 w1753 w1770 w1791 w1806 w1820 w1828 w1868 w1880 w1888 w1897 w1911 w1915 w1922 w1926 w1943 w1961 w1977 w2002 w2026 w2031 w2036 w2044 w2052 w2061 w2098 w2124 w2155 w2168 w2182 w2199 w2205 w2213 w2225 w2246 w2255 w2262 w2331 w2336 w2351 w2376 w2403 w2409 w2415 w2420 w2465 w2483 w2489 w2494 w2500 w2508 w2517 w2527 w2533 w2539 w2544 w2550 w2564 w2598 w2606 w2619 w2629 w2673 w2706 w2711 w2736 w2762 w2787 w2812 w2825 w2888 w2950 w2968 w2979 w2996 w3006 w3010 w3037 w3047 w3051] -> w109
      tunnel: 30 ("Timeout") -> [w120 _ _ _ _ _ _ _ _ _ _ _ _ _ _ _ _ _ _ _ _ _ _ _ _ _ _ _ _ _ _ _ _ _ _ _ _ _ _ _ _ _ _ _ _ _ _ _ _ _ _ _ _ _ _ _ _ _ _ _ _ _ _ _ _ _ _ _ _ _ _ _ _ _ _ _ _ _ _ _ _ _ _ _ _ _ _ _ _ _ _ _ _ _ _ _ _ _ _ _ _ _ _ _ _ _ _ _ _ _ _ _ _ _ _ _ _ _ _ _ _ _ _ _ _ _ _ _ _ _ _ _ _ _ _ _ _ _ _ _ _ _ _ _ _ _ _ _ _ _]
      tunnel: w106 -> [w114 _ _ _ _ _ _ _ _ _ _ _ _ w623 _ _ _ _ w774 _ _ _ _ _ _ _ _ _ _ _ _ _ _ _ _ _ _ _ _ _ _ _ _ _ _ _ _ _ _ _ _ _ _ _ _ _ _ _ _ _ _ _ _ _ _ _ _ _ _ _ _ _ _ _ _ _ _ w1864 _ _ _ w1907 _ _ _ _ _ _ _ _ _ _ _ _ _ _ _ _ _ _ _ _ _ _ _ _ _ _ _ _ _ _ _ _ _ _ _ _ _ _ _ _ _ _ _ _ _ _ _ _ _ _ _ _ _ _ _ _ _ _ w2891 _ _ _ _ _ _ _ _ _]
      tunnel: w105 -> [_ _ _ _ _ _ _ _ _ _ _ _ w611 w632 _ _ _ w724 w780 _ _ _ _ _ _ _ _ _ _ _ _ _ _ _ _ _ _ _ _ _ _ _ _ _ _ _ _ _ _ _ _ _ _ _ _ _ _ _ _ _ _ _ _ _ _ _ _ _ _ _ _ _ _ _ _ _ _ _ w1875 _ w1895 w1906 _ _ _ _ _ _ _ _ _ _ _ _ _ _ _ _ _ _ _ _ _ _ _ _ _ _ _ _ _ _ _ _ _ _ _ _ _ _ _ _ _ _ _ _ _ _ _ _ _ _ _ _ _ _ _ _ _ _ _ _ _ _ _ _ _ _ _ _]
      tunnel: w104 -> [w119 _ _ _ _ _ _ _ _ _ _ _ _ _ _ _ _ _ _ _ _ _ _ _ _ _ _ _ _ _ _ _ _ _ _ _ _ _ _ _ _ _ _ _ _ w1315 _ _ _ _ _ _ _ _ _ _ _ _ _ _ _ _ _ _ _ _ _ _ _ _ _ _ _ _ _ _ _ _ _ _ _ _ _ _ _ _ _ _ _ _ _ _ _ _ _ _ _ _ _ _ _ _ _ _ _ _ _ _ _ _ _ _ _ _ _ _ _ _ _ _ _ _ _ _ _ _ _ _ _ _ _ _ _ _ _ _ _ _ _ _ _ _ _ _ _ _ _ _ _ _]
      tunnel: w103 -> [w118 w457 w467 w472 w480 w489 w499 w509 w530 w548 w569 w585 w612 w633 w648 w662 w691 w726 w781 w816 w821 w826 w831 w848 w865 w889 w894 w902 w914 w926 w939 w955 w974 w998 w1001 w1011 w1030 w1058 w1081 w1106 w1158 w1208 w1231 w1257 w1289 w1319 w1368 w1382 w1388 w1402 w1415 w1426 w1442 w1480 w1497 w1505 w1545 w1548 w1560 w1569 w1578 w1596 w1629 w1653 w1666 w1683 w1694 w1705 w1719 w1731 w1744 w1757 w1773 w1801 w1807 w1819 w1830 w1867 w1879 w1887 w1896 w1905 w1914 w1921 w1928 w1945 w1964 w1980 w2006 w2027 w2030 w2038 w2046 w2051 w2060 w2100 w2140 w2154 w2167 w2180 w2198 w2204 w2216 w2228 w2247 w2251 w2263 w2330 w2343 w2355 w2379 w2399 w2407 w2413 w2427 w2476 w2481 w2487 w2493 w2499 w2507 w2516 w2526 w2532 w2538 w2543 w2549 w2563 w2597 w2605 w2618 w2630 w2684 w2705 w2710 w2737 w2761 w2786 w2811 w2829 w2892 w2949 w2967 w2978 w3002 w3005 w3029 w3036 w3046 w3050]
      tunnel: [w116 w457 w467 w472 w480 w489 w499 w509 w530 w548 w569 w585 w612 w633 w648 w662 w691 w726 w781 w816 w821 w826 w831 w848 w865 w889 w894 w902 w914 w926 w939 w955 w974 w998 w1001 w1011 w1030 w1058 w1081 w1106 w1158 w1208 w1231 w1257 w1289 w1319 w1368 w1382 w1388 w1402 w1415 w1426 w1442 w1480 w1497 w1505 w1545 w1548 w1560 w1569 w1578 w1596 w1629 w1653 w1666 w1683 w1694 w1705 w1719 w1731 w1744 w1757 w1773 w1801 w1807 w1819 w1830 w1867 w1879 w1887 w1896 w1905 w1914 w1921 w1928 w1945 w1964 w1980 w2006 w2027 w2030 w2038 w2046 w2051 w2060 w2100 w2140 w2154 w2167 w2180 w2198 w2204 w2216 w2228 w2247 w2251 w2263 w2330 w2343 w2355 w2379 w2399 w2407 w2413 w2427 w2476 w2481 w2487 w2493 w2499 w2507 w2516 w2526 w2532 w2538 w2543 w2549 w2563 w2597 w2605 w2618 w2630 w2684 w2705 w2710 w2737 w2761 w2786 w2811 w2829 w2892 w2949 w2967 w2978 w3002 w3005 w3029 w3036 w3046 w3050] -> w102
      tunnel: w100 -> [_ _ _ _ _ _ _ _ _ _ _ _ _ _ _ _ _ _ _ _ _ _ _ _ _ _ _ _ _ _ _ _ _ _ _ _ _ _ _ _ _ _ _ _ _ _ _ _ _ _ _ _ _ _ _ _ _ _ _ _ _ _ _ _ _ _ _ _ _ _ _ _ _ _ _ _ _ _ _ _ _ w1904 _ _ _ _ _ _ _ _ _ _ _ _ _ _ _ _ _ _ _ _ _ _ _ _ _ _ _ _ _ _ _ _ _ _ _ _ _ _ _ _ _ _ _ _ _ _ _ _ _ _ _ _ _ _ _ _ _ _ _ _ _ _ _ _ _ _ _ _]
      tunnel: w95 -> [w117 _ _ _ _ _ _ _ _ _ _ _ _ _ _ _ _ _ _ _ _ _ _ _ _ _ _ _ _ _ _ _ _ _ _ _ _ _ _ _ _ _ _ _ _ _ _ _ _ _ _ _ _ _ _ _ _ _ _ _ _ _ _ _ _ _ _ _ _ _ _ _ _ _ _ _ w1829 w1866 _ _ _ _ _ _ _ _ _ _ _ _ _ _ _ _ _ _ _ _ _ _ _ _ _ _ _ _ _ _ _ _ _ _ _ _ _ _ _ _ _ _ _ _ _ _ _ _ _ _ _ _ _ _ _ _ _ _ _ _ _ _ _ _ _ w2976 _ _ _ _ _ _]
      tunnel: w94 -> [w115 _ _ _ _ _ _ _ _ _ _ _ w601 _ _ w660 _ w707 _ _ _ _ _ _ _ _ _ _ _ _ _ _ _ _ _ _ _ _ _ _ _ _ _ _ _ _ _ _ _ _ _ _ _ _ _ _ _ _ _ _ _ _ _ _ _ _ _ _ _ _ _ _ _ _ _ _ _ w1860 _ _ _ w1901 _ _ _ _ _ _ _ _ _ _ _ _ _ _ _ _ _ _ _ _ _ _ _ _ _ _ _ _ _ _ _ _ _ _ _ _ _ _ _ _ _ _ _ _ _ _ _ _ _ _ _ _ _ _ _ _ _ w2827 _ _ _ _ _ _ _ _ _ _]
      frame "", "Event Structure", "Idle" {
        # "executes when the state queue is empty"
        n52 = event shown="[15] \"StartButton\": Mouse Enter" {
          selector: w118 -> [_ _ _ _ _ _ _ _ _ _ _ _ _ _ _ _ _ _ _ _ _ _ _ _ _ _ _ _ _ _ _ _ _ _ _ _]
          dyn-events: [_ _ _ _ _ _ _ _ _ _ _ _ _ _ _ _ _ _ _ _ _ _ _ _ _ _ _ _ _ _ _ _ _ _ _ _] -> w116
          timeout: w120 -> [_ _ _ _ _ _ _ _ _ _ _ _ _ _ _ _ _ _ _ _ _ _ _ _ _ _ _ _ _ _ _ _ _ _ _ _]
          tunnel: w126 -> [w142 w151 w160 w172 w180 w197 w210 w227 w234 w241 w254 w265 w270 w276 w292 w296 w300 w305 w309 w314 w327 w333 w338 w342 w346 w357 w364 w382 w399 w404 w411 w416 w424 w433 w447 w456]
          tunnel: [w143 w151 w159 w172 w179 w197 w209 w226 w234 w240 w254 w265 w269 w277 w291 w296 w301 w305 w310 w314 w328 w332 w338 w342 w345 w358 w363 w381 w399 w405 w410 w415 w424 w433 w447 w455] -> w125
          tunnel: w124 -> [w129 w149 w153 w174 w182 w196 w211 w225 w233 w237 w253 w264 w266 w278 w290 w294 w298 w303 w307 w312 w316 w334 w336 w340 w347 w356 w366 w383 w397 w406 w412 w417 w419 w428 w445 w453]
          tunnel: [w131 w150 w156 w175 w183 w195 w202 w224 w230 w243 w250 w260 w268 w271 w286 w295 w299 w304 w308 w313 w324 w335 w337 w341 w348 w359 w367 w384 w398 w401 w413 w418 w423 w426 w446 w454] -> w123
          tunnel: w122 -> [w131 w150 w161 w175 w183 w195 w203 w224 w231 w242 w249 w259 w268 w272 w287 w295 w299 w304 w308 w313 w326 w335 w337 w341 w348 w359 w367 w384 w398 w400 w413 w418 w423 w425 w446 w454]
          tunnel: [w129 w149 w153 w174 w182 w196 w211 w225 w233 w236 w253 w264 w266 w278 w290 w294 w298 w303 w307 w312 w315 w334 w336 w340 w347 w356 w366 w383 w397 w407 w412 w417 w419 w429 w445 w453] -> w121
          tunnel: w119 -> [_ _ _ _ _ _ _ _ _ _ _ _ _ _ _ _ _ _ _ _ _ _ _ _ _ _ _ _ _ _ _ _ _ _ _ _]
          tunnel: w117 -> [_ _ _ _ _ _ _ _ _ _ _ _ _ _ _ _ _ _ _ _ _ _ _ _ _ _ _ _ _ _ _ _ _ _ _ _]
          tunnel: w115 -> [_ _ _ _ _ _ _ _ _ _ _ _ _ _ _ _ _ _ _ _ _ _ _ _ _ _ _ _ _ _ _ _ _ w427 _ _]
          tunnel: w114 -> [_ _ _ _ _ _ _ _ _ _ _ _ _ _ _ _ _ _ _ _ _ _ _ _ _ _ _ _ _ w402 _ _ _ _ _ _]
          event Timeout {
            # "check system status every 2s"
            n53 = event-data() -> ()  [unwired: 1 in, 1 out]
            n54 = Unbundle By Name(w129) -> ("SlowTimer"=w127:u32, "FastTimer"=w128:u32)
            n55 = Tick Count (ms)() -> (millisecond timer value=w132:u32)
            n56 = Subtract(x=w132, y=w127) -> (x-y=w137:u32)
            n57 = Subtract(x=w132, y=w128) -> (x-y=w133:u32)
            n58 = Greater?(x=w137, y=u32 2000) -> (0:w138:bool)
            n59 = Greater?(x=w133, y=u32 500) -> (0:w135:bool)
            n60 = case shown="True" w138 {
              tunnel: ["" ("Empty String Constant") "SystemStatus: SlowSysStatusMacro" ("State(s) in Front (\"\")")] -> w139
              frame False {
              }
              frame True {
              }
            }
            n61 = case shown="True" w135 {
              tunnel: ["" ("Empty String Constant") "SystemStatus: FastSysStatusMacro" ("State(s) in Front (\"\")")] -> w134
              frame False {
              }
              frame True {
              }
            }
            n62 = call <vilib>:"Add State(s) to Queue__JKI_lib_State_Machine.vi"("State(s) in Front (\"\")"="LabJack: checkPedal\nData: SignInRange" ("State(s) in Front (\"\")"), "State(s) in (\"\")"=w139, "State(s) at Back (\"\")"=w134) -> ("States Out"=w130:string)  [unwired: 12 in]
            n63 = call <vilib>:"Add State(s) to Queue__JKI_lib_State_Machine.vi"("State(s) in Front (\"\")"=w130, "State(s) in (\"\")"=w142) -> ("States Out"=w143:string)  [unwired: 13 in]
          }
          event "355nm Laser toggle": Mouse Enter {
            n64 = event-data() -> ()  [unwired: 1 in, 4 out]
            n65 = local write "Help"("Toggle 355nm laser." ("Help")) -> ()
          }
          event "355nm Laser toggle": Value Change {
            n66 = event-data() -> ()  [unwired: 1 in, 6 out]
            n67 = case shown="False" "355nm Laser toggle" {
              tunnel: [0.0 ("Value") 1.0 ("Value")] -> w163
              frame False {
                n68 = property on="Laser Rep Rate" class="DigNum (strict)"("DisabledEnum"=T11."Enabled" ("Disabled")) -> ()  [unwired: 2 in, 2 out]
              }
              frame True {
                n69 = property on="Laser Rep Rate" class="DigNum (strict)"("DisabledEnum"=T11."Disabled and Grayed Out" ("Disabled")) -> ()  [unwired: 2 in, 2 out]
              }
            }
            n70 = Unbundle By Name(w153) -> ("LJ Pinout.355 PWM"=w152:string)
            n71 = call "LabJack_FGV.vi"("Operation(Read)"=enum16{"Write", "Read"}."Read" ("Operation"), "error in (no error)"=w161) -> ("error out"=w165:errorcluster, "Read data"=w166:i32)  [unwired: 8 in]
            n72 = Concatenate Strings(w152, "_EF_ENABLE" ("string")) -> (w162:string)
            n73 = call "LJM_eWriteName.vi"("Handle In"=w166, "Name"=w162, "Value"=w163, "error in"=w165) -> ("error out"=w157:errorcluster)  [unwired: 10 in, 1 out]
            n74 = call <vilib>:"Add State(s) to Queue__JKI_lib_State_Machine.vi"("State(s) in Front (\"\")"="/*355 Laser: CheckControllerStatus\n/*355 Laser: CheckPWMStatus" ("State(s) in Front (\"\")"), "State(s) in (\"\")"=w160) -> ("States Out"=w159:string)  [unwired: 13 in]
            n75 = call <userlib>:"Wait (ms)__ogtk.vi"("error in (no error)"=w157, "milliseconds to wait"=u32 50) -> ("error out"=w156:errorcluster)  [unwired: 8 in, 1 out]
          }
          event "Aiming beam toggle": Mouse Enter {
            n76 = event-data() -> ()  [unwired: 1 in, 4 out]
            n77 = local write "Help"("Toggle aiming beam laser." ("Help")) -> ()
          }
          event "Aiming beam toggle": Value Change {
            # "[Covers: REQ27]"
            n78 = event-data() -> ("NewVal"=w181:bool)  [unwired: 1 in, 5 out]
            n79 = local read "AB Rep Rate"() -> (w177:u16)
            n80 = Equal To 0?(x=w177) -> (x = 0?=w176:bool)
            n81 = case shown="False" w181 {
              tunnel: [w184 w191] -> w178
              tunnel: w176 -> [w187 w189]
              frame False {
                w188 = T11."Enabled" ("Disabled")
                n82 = Select(t="LabJack: AB_DC_Stop" ("State(s) in Front (\"\")"), s=w187, f="LabJack: AB_PWM_Stop" ("State(s) in Front (\"\")")) -> (s? t:f=w184:string)
                n83 = property on="Current" class="DigNum (strict)"("DisabledEnum"=w188) -> ()  [unwired: 2 in, 2 out]
                n84 = property on="AB Rep Rate" class="DigNum (strict)"("DisabledEnum"=w188) -> ()  [unwired: 2 in, 2 out]
              }
              frame True {
                w193 = T11."Disabled and Grayed Out" ("Disabled")
                n85 = Select(t="LabJack: AB_DC_Start" ("State(s) in Front (\"\")"), s=w189, f="LabJack: AB_PWM_Start" ("State(s) in Front (\"\")")) -> (s? t:f=w191:string)
                n86 = property on="AB Rep Rate" class="DigNum (strict)"("DisabledEnum"=w193) -> ()  [unwired: 2 in, 2 out]
                n87 = property on="Current" class="DigNum (strict)"("DisabledEnum"=w193) -> ()  [unwired: 2 in, 2 out]
              }
            }
            n88 = call <vilib>:"Add State(s) to Queue__JKI_lib_State_Machine.vi"("State(s) in Front (\"\")"=w178, "State(s) in (\"\")"=w180) -> ("States Out"=w179:string)  [unwired: 13 in]
          }
          event "Auto gain": Value Change {
            n89 = event-data() -> ("NewVal"=w194:bool)  [unwired: 1 in, 5 out]
            n90 = case shown="True" w194 {
              frame False {
                n91 = local read "Ctrl V"() -> (w198:dbl)
                n92 = call "V1FGV.vi"("action (write)"=enum16{"write", "read"}."write" ("action"), "V1 in"=w198) -> ()  [unwired: 8 in, 2 out]
                n93 = property on="Ctrl V" class="DigNum (strict)"("DisabledEnum"=T11."Enabled" ("Disabled")) -> ()  [unwired: 2 in, 2 out]
              }
              frame True {
                n94 = property on="Ctrl V" class="DigNum (strict)"("DisabledEnum"=T11."Disabled and Grayed Out" ("Disabled")) -> ()  [unwired: 2 in, 2 out]
              }
            }
          }
          event "Channel": Value Change {
            n95 = event-data() -> ("NewVal"=w207:enum32{"Ch1", "Ch2", "Ch3", "Ch4"})  [unwired: 1 in, 5 out]
            n96 = case shown="\"Ch4\"" w207 {
              tunnel: [w213 w215 w217 w218] -> w206
              frame "Ch1", Default {
                n97 = local read "Ch1 Max CtrlV"() -> (w213:dbl)
                n98 = local write "Tab Control"(T2."APD1" ("Tab Control")) -> ()
              }
              frame "Ch2" {
                n99 = local read "Ch2 Max CtrlV"() -> (w215:dbl)
                n100 = local write "Tab Control"(T2."APD2" ("Tab Control")) -> ()
              }
              frame "Ch3" {
                n101 = local read "Ch3 Max CtrlV"() -> (w217:dbl)
                n102 = local write "Tab Control"(T2."APD3" ("Tab Control")) -> ()
              }
              frame "Ch4" {
                n103 = local read "Ch4 Max CtrlV"() -> (w218:dbl)
                n104 = local write "Tab Control"(T2."APD4" ("Tab Control")) -> ()
              }
            }
            n105 = local write "Gain High"(w206) -> ()
            n106 = call "V1FGV.vi"("Error In"=w203, "action (write)"=enum16{"write", "read"}."write" ("action"), "V1 in"=0.0) -> ("Error Out"=w202:errorcluster)  [unwired: 7 in, 1 out]
            n107 = call <vilib>:"Add State(s) to Queue__JKI_lib_State_Machine.vi"("State(s) in Front (\"\")"="UI: Cursor Set >> Busy\nDigitizer: ConfigMacro\nUI: Cursor Set >> Idle" ("State(s) in Front (\"\")"), "State(s) in (\"\")"=w210) -> ("States Out"=w209:string)  [unwired: 13 in]
          }
          event "Task": Value Change {
            n108 = event-data() -> ("NewVal"=w223:enum32{"iRFAndGain", "Alignment"})  [unwired: 1 in, 5 out]
            n109 = case shown="\"iRFAndGain\", Default" w223 {
              tunnel: ["SysConfig: Load Digitizer Setting\nUI: Update" ("State(s) in Front (\"\")") "SysConfig: Load Digitizer Setting Gain\nUI: Update" ("State(s) in Front (\"\")")] -> w222
              frame "iRFAndGain", Default {
                # "load iRF setting"
              }
              frame "Alignment" {
                # "load gain setting"
              }
            }
            n110 = call <vilib>:"Add State(s) to Queue__JKI_lib_State_Machine.vi"("State(s) in Front (\"\")"=w222, "State(s) in (\"\")"="UI: Cursor Set >> Busy\nDigitizer: ConfigMacro\nUI: Cursor Set >> Idle" ("State(s) in Front (\"\")")) -> ("States Out"=w220:string)  [unwired: 13 in]
            n111 = call <vilib>:"Add State(s) to Queue__JKI_lib_State_Machine.vi"("State(s) in Front (\"\")"=w220, "State(s) in (\"\")"=w227) -> ("States Out"=w226:string)  [unwired: 13 in]
          }
          event "Waveform (no average)": Cursor Move {
            n112 = event-data() -> ()  [unwired: 1 in, 9 out]
            n113 = control-ref of="Waveform (no average)"() -> (w232:refnum<vi>)
            n114 = call "UpdateCurserIdx(SubVI).vi"("error in (no error)"=w231, "WaveformGraph in"=w232) -> ("error out"=w230:errorcluster)  [unwired: 9 in]
          }
          event "Current": Value Change {
            n115 = event-data() -> ()  [unwired: 1 in, 6 out]
            n116 = Unbundle By Name(w237) -> ("AB Cluster"=w238:T21)
            n117 = Bundle By Name(cluster=w238, "Default Current"="Current") -> (w235:T21)
            n118 = Bundle By Name(cluster=w237, "AB Cluster"=w235) -> (w236:T22)
            n119 = call "writeAimingBeamSetting.vi"("error in"=w242, "Aiming Beam Cluster"=w235) -> ("error out"=w243:errorcluster)  [unwired: 9 in]
            n120 = call <vilib>:"Add State(s) to Queue__JKI_lib_State_Machine.vi"("State(s) in Front (\"\")"="SysConfig: Load AB setting\nAimingBeam: Set Current" ("State(s) in Front (\"\")"), "State(s) in (\"\")"=w241) -> ("States Out"=w240:string)  [unwired: 13 in]
          }
          event "Ctrl V": Value Change; "Ctrl V": Key Down {
            n121 = event-data() -> ()  [unwired: 1 in, 4 out]
            n122 = local read "Channel"() -> (w251:enum32{"Ch1", "Ch2", "Ch3", "Ch4"})
            n123 = case shown="\"Ch4\"" w251 {
              tunnel: [enum16{"Ch1", "Ch2", "Ch3", "Ch4"}."Ch1" ("Channel") enum16{"Ch1", "Ch2", "Ch3", "Ch4"}."Ch2" ("Channel") enum16{"Ch1", "Ch2", "Ch3", "Ch4"}."Ch3" ("Channel") enum16{"Ch1", "Ch2", "Ch3", "Ch4"}."Ch4" ("Channel")] -> w245
              frame "Ch1", Default {
              }
              frame "Ch2" {
              }
              frame "Ch3" {
              }
              frame "Ch4" {
              }
            }
            n124 = call "CtrlVtoGain.vi"("error in (no error)"=w249, "CtrlV(V)"="Ctrl V", "Channel"=w245) -> ("error out"=w250:errorcluster, "Gain"=→"GainIndicator":dbl)  [unwired: 7 in]
            n125 = formula code="float32 y=0.05;\nif (x>0&&x<3.8)\ny=0.1;\nif (x>=3.8&&x<4.4)\ny=0.02;\nif (x>=4.4)\ny=0.01;"("x"="Ctrl V") -> ("y"=w246:sgl)
            n126 = call "V1FGV.vi"("action (write)"=enum16{"write", "read"}."write" ("action"), "V1 in"="Ctrl V") -> ()  [unwired: 8 in, 2 out]
            n127 = property on="Ctrl V" class="DigNum (strict)"("Increment"=w246) -> ()  [unwired: 2 in, 2 out]
          }
          event "Save PID": Value Change {
            n128 = event-data() -> ()  [unwired: 1 in, 6 out]
            n129 = local read "Ch1 PID gains"() -> (w263:T6)
            n130 = local read "Ch2 PID gains"() -> (w262:T6)
            n131 = local read "Ch3 PID gains"() -> (w261:T6)
            n132 = call "writePIDSetting.vi"("Error In"=w259, "Ch3 PID gains"=w261, "Ch2 PID gains"=w262, "Ch1 PID gains"=w263) -> ("Error Out"=w260:errorcluster)  [unwired: 7 in]
          }
          event "Quit": Value Change {
            # "Exit Button Value Change (pressed) Event\n(when pressed.  quite)"
            n133 = event-data() -> ()  [unwired: 1 in, 1 out]
            n134 = call <vilib>:"Add State(s) to Queue__JKI_lib_State_Machine.vi"("State(s) in Front (\"\")"="LED: Off\nMacro: Exit", "State(s) in (\"\")"=w270) -> ("States Out"=w269:string)  [unwired: 13 in]
          }
          event "Laser Rep Rate": Value Change {
            n135 = event-data() -> ()  [unwired: 1 in, 6 out]
            n136 = call "LJ_calculate_PWM_parameters.vi"("Error In"=w272, "Laser Rep Rate (Hz)"="Laser Rep Rate", "Laser"=enum16{"355nm", "AimingBeam"}."355nm") -> ("Error Out"=w271:errorcluster)  [unwired: 7 in, 1 out]
            n137 = call <vilib>:"Add State(s) to Queue__JKI_lib_State_Machine.vi"("State(s) in Front (\"\")"="SysConfig: Load 355 PWM\nLabJack: 355_PWM_Config" ("State(s) in Front (\"\")"), "State(s) in (\"\")"=w276) -> ("States Out"=w277:string)  [unwired: 13 in]
          }
          event "AB Rep Rate", "Duty Cycle (%)": Value Change {
            n138 = event-data() -> ()  [unwired: 1 in, 6 out]
            n139 = Unbundle By Name(w290) -> ("AB Cluster"=w289:T21)
            n140 = Bundle By Name(cluster=w289, "Frequency(Hz)"="AB Rep Rate") -> (w288:T21)
            n141 = call "writeAimingBeamSetting.vi"("error in"=w287, "Aiming Beam Cluster"=w288) -> ("error out"=w286:errorcluster)  [unwired: 9 in]
            n142 = Equal To 0?(x="AB Rep Rate") -> (x = 0?=w284:bool)
            n143 = Select(t="", s=w284, f="AimingBeam: ComputePWM\nSysConfig: Load AB PWM\nLabJack: AB_PWM_Config" ("State(s) in Front (\"\")")) -> (s? t:f=w280:string)
            n144 = call <vilib>:"Add State(s) to Queue__JKI_lib_State_Machine.vi"("State(s) in Front (\"\")"="SysConfig: Load AB setting" ("State(s) in Front (\"\")"), "State(s) in (\"\")"=w280) -> ("States Out"=w279:string)  [unwired: 13 in]
            n145 = call <vilib>:"Add State(s) to Queue__JKI_lib_State_Machine.vi"("State(s) in Front (\"\")"=w279, "State(s) in (\"\")"=w292) -> ("States Out"=w291:string)  [unwired: 13 in]
          }
          event "StartButton": Mouse Enter {
            n146 = event-data() -> ()  [unwired: 1 in, 4 out]
            n147 = local write "Help"("Press to start aquisition." ("Help")) -> ()
          }
          event "StartButton": Value Change {
            # "Initialize both digitizer aquisition and\n send user event to trigger aquisition loop"
            n148 = event-data() -> ()  [unwired: 1 in, 6 out]
            n149 = call <vilib>:"Add State(s) to Queue__JKI_lib_State_Machine.vi"("State(s) in Front (\"\")"="Macro: StartRun" ("State(s) in Front (\"\")"), "State(s) in (\"\")"=w300) -> ("States Out"=w301:string)  [unwired: 13 in]
          }
          event "StopButton": Mouse Enter {
            n150 = event-data() -> ()  [unwired: 1 in, 4 out]
            n151 = local write "Help"("Press to stop data aquisition." ("Help")) -> ()
          }
          event "StopButton": Value Change {
            n152 = event-data() -> ()  [unwired: 1 in, 6 out]
            n153 = call <vilib>:"Add State(s) to Queue__JKI_lib_State_Machine.vi"("State(s) in Front (\"\")"="Macro: StopRun" ("State(s) in Front (\"\")"), "State(s) in (\"\")"=w309) -> ("States Out"=w310:string)  [unwired: 13 in]
          }
          event "Sys Reconfig": Mouse Enter {
            n154 = event-data() -> ()  [unwired: 1 in, 4 out]
            n155 = local write "Help"("Click to reconfig digitizer settings." ("Help")) -> ()
          }
          event "Sys Reconfig": Value Change {
            # "everytime the user change data aquisition setting, need to reinitilize decon engine and realign iRF.\ncheck whether data length has changed, if changed, reinitialize Decon engine\nreset BG ready, need a new BG"
            # "update DAQ FGV"
            n156 = event-data() -> ()  [unwired: 1 in, 6 out]
            n157 = call "SystemConfigEditorV6.vi"("error in"=w326) -> ("error out"=w325:errorcluster, "FLImDAQ out"=w322:T4)  [unwired: 1 in]
            n158 = Unbundle By Name(w316) -> ("FLImDAQ.min record length"=w317:i32)
            n159 = Unbundle By Name(w322) -> ("min record length"=w323:i32)
            n160 = call "FLImDAQ_FGV.vi"("error in (no error)"=w325, "Operation (Read)"=enum16{"Write", "Read"}."Write" ("Operation"), "Write data"=w322) -> ("error out"=w324:errorcluster, "Read data"=w321:T4)  [unwired: 7 in]
            n161 = Equal?(x=w317, y=w323) -> (x = y?=w320:bool)
            n162 = case shown="False" w320 {
              tunnel: ["UI: Cursor Set >> Busy\nDigitizer: ConfigMacro\n/*UI: CaliAndiRFNotReady\n/*UI iRF not ready\nUI: Update\nUI: Cursor Set >> Idle" "UI: Cursor Set >> Busy\nDigitizer: ConfigCh3iRF\nUI: Update\nUI: Cursor Set >> Idle"] -> w319
              frame False {
              }
              frame True {
              }
            }
            n163 = Bundle By Name(cluster=w316, "FLImDAQ"=w321) -> (w315:T22)
            n164 = call <vilib>:"Add State(s) to Queue__JKI_lib_State_Machine.vi"("State(s) in Front (\"\")"=w319, "State(s) in (\"\")"=w327) -> ("States Out"=w328:string)  [unwired: 13 in]
          }
          event "Clear WF Chart History": Value Change {
            n165 = event-data() -> ()  [unwired: 1 in, 6 out]
            n166 = call <vilib>:"Add State(s) to Queue__JKI_lib_State_Machine.vi"("State(s) in Front (\"\")"="Graph: ClearHistory" ("State(s) in Front (\"\")"), "State(s) in (\"\")"=w333) -> ("States Out"=w332:string)  [unwired: 13 in]
          }
          event "System Hardware Connection Status", "StartButton", "StopButton", "355nm Laser toggle", "Aiming beam toggle", "Sys Reconfig": Mouse Leave {
            n167 = event-data() -> ()  [unwired: 1 in, 4 out]
            n168 = invoke on="Help" class="Str" method="Reinit To Default"() -> ()  [unwired: 3 in, 3 out]
          }
          event "System Hardware Connection Status.Digitizer": Mouse Enter {
            n169 = event-data() -> ()  [unwired: 1 in, 4 out]
            n170 = local write "Help"("Status of hardware connections. TCP/IP is optional." ("Help")) -> ()
          }
          event "TCP Connect": Value Change {
            n171 = event-data() -> ("NewVal"=w343:bool)  [unwired: 1 in, 5 out]
            n172 = case shown="False" w343 {
              tunnel: ["UI: Update" ("State(s) in Front (\"\")") "UI: Update" ("State(s) in Front (\"\")")] -> w344
              frame False {
              }
              frame True {
              }
            }
            n173 = call <vilib>:"Add State(s) to Queue__JKI_lib_State_Machine.vi"("State(s) in Front (\"\")"=w344, "State(s) in (\"\")"=w346) -> ("States Out"=w345:string)  [unwired: 13 in]
          }
          event User Event {
            # "if aquisition loop is error out. Stop digitizer, flash queue, update front panel indicator, stop both laser and parse and save data"
            n174 = event-data() -> ()  [unwired: 1 in, 5 out]
            n175 = case shown="True" FALSE {
              tunnel: ["" ("Empty String Constant") "Data: parseRunDataMacro" ("State(s) in Front (\"\")")] -> w354
              frame False {
                # "if flag is 0, do not save data"
              }
              frame True {
                # "if save data flag is true enqueue data"
              }
            }
            n176 = call <vilib>:"Add State(s) to Queue__JKI_lib_State_Machine.vi"("State(s) in Front (\"\")"="Digitizer: Abort\nLabJack: ZeroV" ("State(s) in Front (\"\")"), "State(s) in (\"\")"=w354, "State(s) at Back (\"\")"="LED: BreathOff\nMacro: SysReadyForAqui\nUI: Update" ("State(s) in Front (\"\")")) -> ("States Out"=w355:string)  [unwired: 12 in]
            n177 = call <vilib>:"Add State(s) to Queue__JKI_lib_State_Machine.vi"("State(s) in Front (\"\")"=w355, "State(s) in (\"\")"=w357) -> ("States Out"=w358:string)  [unwired: 13 in]
          }
          event "AcquireGain": Value Change {
            n178 = event-data() -> ()  [unwired: 1 in, 6 out]
            n179 = local read "GainSigInRange"() -> (w365:bool)
            n180 = case shown="True" w365 {
              tunnel: ["" ("State(s) in Front (\"\")") w370] -> w362
              frame False {
                n181 = One Button Dialog(message="Please make sure peak voltage is with in 0.3V to 1.4V and try again!") -> ()  [unwired: 1 in, 1 out]
              }
              frame True {
                n182 = local read "Laser Rep Rate"() -> (w374:u16)
                n183 = In Range and Coerce(upper limit=u16 1500, x=w374, lower limit=u16 50) -> (In Range?=w371:bool)  [unwired: 1 out]
                n184 = case shown="False" w371 {
                  tunnel: ["" ("State(s) in Front (\"\")") "UI: Cursor Set >> Busy\nUtility: EnableGain? >> False\nUtility: setSaveFlag >> 0\nQueue: Flash\nUtility: setSaveFlag >> 1\nQueue: CheckNumOfWF\nData: parseSingleGainData\nUI: UpdateGainDataIndicators\nUtility: EnableGain? >> True\nUI: Cursor Set >> Idle\n" ("State(s) in Front (\"\")")] -> w370
                  frame False {
                    n185 = One Button Dialog(message="Please set 355nm laser rep rate between 20 and 1500Hz ") -> ()  [unwired: 1 in, 1 out]
                  }
                  frame True {
                    n186 = local write "Num WF to acquire"(500) -> ()
                  }
                }
              }
            }
            n187 = call <vilib>:"Add State(s) to Queue__JKI_lib_State_Machine.vi"("State(s) in Front (\"\")"=w362, "State(s) in (\"\")"=w364) -> ("States Out"=w363:string)  [unwired: 13 in]
          }
          event "AcquireIRF": Value Change {
            n188 = event-data() -> ()  [unwired: 1 in, 6 out]
            n189 = local read "iRFSigInRange"() -> (w379:bool)
            n190 = case shown="True" w379 {
              tunnel: ["" ("State(s) in Front (\"\")") w387] -> w380
              frame False {
                n191 = One Button Dialog(message="Please make sure peak voltage is with in 0.5V to 1.4V and try again!") -> ()  [unwired: 1 in, 1 out]
              }
              frame True {
                n192 = local read "Laser Rep Rate"() -> (w391:u16)
                n193 = In Range and Coerce(upper limit=u16 1500, x=w391, lower limit=u16 20) -> (In Range?=w388:bool)  [unwired: 1 out]
                n194 = case shown="False" w388 {
                  tunnel: ["" ("State(s) in Front (\"\")") "UI: Cursor Set >> Busy\nUtility: EnableGain? >> False\nUtility: setSaveFlag >> 0\nQueue: Flash\nUtility: setSaveFlag >> 1\nQueue: CheckNumOfWF\nData: parseIRFSingleIRFData\nUI: UpdateIRFDataTable\nUtility: EnableGain? >> True\nUI: Cursor Set >> Idle\n" ("State(s) in Front (\"\")")] -> w387
                  frame False {
                    n195 = One Button Dialog(message="Please set 355nm laser rep rate between 20 and 1500Hz ") -> ()  [unwired: 1 in, 1 out]
                  }
                  frame True {
                    n196 = local write "Num WF to acquire"(500) -> ()
                  }
                }
              }
            }
            n197 = call <vilib>:"Add State(s) to Queue__JKI_lib_State_Machine.vi"("State(s) in Front (\"\")"=w380, "State(s) in (\"\")"=w382) -> ("States Out"=w381:string)  [unwired: 13 in]
          }
          event "Tab Control": Value Change {
            n198 = event-data() -> ()  [unwired: 1 in, 6 out]
            n199 = case shown="\"Data parsing\"" "Tab Control" {
              frame "APD1", Default {
              }
              frame "APD2" {
              }
              frame "APD3" {
              }
              frame "Debug" {
              }
              frame "IO Ststus" {
              }
              frame "LJ pinout" {
              }
              frame "Digitizer Info" {
              }
              frame "Data parsing" {
              }
              frame "Intensity Trace" {
              }
              frame "iRF Measureement" {
              }
              frame "Gain Measurement" {
              }
            }
          }
          event "ClearIRFData": Value Change {
            n200 = event-data() -> ()  [unwired: 1 in, 6 out]
            n201 = Bundle By Name(cluster=w406, "iRFIdx"=0) -> (w407:T22)
            n202 = Flush Queue(queue=w402, error in (no error)=w400) -> (error out=w401:errorcluster)  [unwired: 2 out]
            n203 = call <vilib>:"Add State(s) to Queue__JKI_lib_State_Machine.vi"("State(s) in Front (\"\")"="UI: InitIRFDataTable" ("State(s) in Front (\"\")"), "State(s) in (\"\")"=w404) -> ("States Out"=w405:string)  [unwired: 13 in]
          }
          event "SaveGainData": Value Change {
            n204 = event-data() -> ()  [unwired: 1 in, 6 out]
            n205 = call <vilib>:"Add State(s) to Queue__JKI_lib_State_Machine.vi"("State(s) in Front (\"\")"="UI: Cursor Set >> Busy\nAPD: LoadFromSerial\nAPD: writeGain\nFile: BackupOld\nAPD: SaveNew\nAPD: LoadFromSerialNoRawData\nAPD: UpdateIndicatorCh1\nAPD: UpdateIndicatorCh2\nAPD: UpdateIndicatorCh3\nAPD: UpdateIndicatorCh4\nUI: Cursor Set >> Idle" ("State(s) in Front (\"\")"), "State(s) in (\"\")"=w411) -> ("States Out"=w410:string)  [unwired: 13 in]
          }
          event "SaveiRFData": Value Change {
            n206 = event-data() -> ()  [unwired: 1 in, 6 out]
            n207 = call <vilib>:"Add State(s) to Queue__JKI_lib_State_Machine.vi"("State(s) in Front (\"\")"="UI: Cursor Set >> Busy\nAPD: LoadFromSerial\nAPD: writeiRF\nFile: BackupOld\nAPD: SaveNew\nAPD: LoadFromSerialNoRawData\nAPD: UpdateIndicatorCh1\nAPD: UpdateIndicatorCh2\nAPD: UpdateIndicatorCh3\nAPD: UpdateIndicatorCh4\nUI: Cursor Set >> Idle" ("State(s) in Front (\"\")"), "State(s) in (\"\")"=w416) -> ("States Out"=w415:string)  [unwired: 13 in]
          }
          event "SetIRFCtrlV": Value Change {
            # "set iRF V"
            n208 = event-data() -> ()  [unwired: 1 in, 6 out]
            n209 = local read "iRFCtrlV"() -> (w422:dbl[])
            n210 = Unbundle By Name(w419) -> ("iRFIdx"=w420:i32)
            n211 = Index Array(array=w422, index=w420) -> (element=w421:dbl)
            n212 = property on="Ctrl V" class="DigNum (strict)"("Val(Sgnl)"=w421) -> ()  [unwired: 2 in, 2 out]
          }
          event "ClearGainData": Value Change {
            w432 = dbl[] [] ("Gain")
            n213 = event-data() -> ()  [unwired: 1 in, 6 out]
            n214 = Flush Queue(queue=w427, error in (no error)=w425) -> (error out=w426:errorcluster)  [unwired: 2 out]
            n215 = local write "GainDataTable"(string[][] [] ("Table Control")) -> ()
            n216 = Bundle By Name(cluster=w428, "GainDataTemp"=T12 {"CtrlV"=-1.0, "PeakV"=0.0, "PeakV Std"=0.0, "IntFactor"=1.0, "IntCorrPeakV"=0.0}) -> (w429:T22)
            n217 = local write "Gain"(w432) -> ()
            n218 = local write "Ctrl V"(w432) -> ()
            n219 = local write "Intensity Factor"(w432) -> ()
            n220 = local write "AUC Std"(w432) -> ()
            n221 = local write "AUC"(w432) -> ()
            n222 = local write "Int Corr AUC"(w432) -> ()
          }
          event "ComputeGain": Value Change {
            # "Devide Int corrected Peak V by the 1st element"
            n223 = event-data() -> ()  [unwired: 1 in, 6 out]
            n224 = local read "Int Corr AUC"() -> (w444:dbl[])
            n225 = local read "Ctrl V"() -> (w436:dbl[])
            n226 = Reverse 1D Array(array=w444) -> (reversed array=w443:dbl[])
            n227 = Index Array(array=w443, index=0) -> (element=w441:dbl)
            n228 = local read "GainDataTable"() -> (w440:string[][])
            n229 = Divide(x=w444, y=w441) -> (x/y=w435:dbl[])
            "Gain" <- w435
            n230 = Bundle("Ctrl V"=w436, w435) -> (→"XY Graph":cluster{"Ctrl V":dbl[], dbl[]})  [unwired: 1 in]
            n231 = for {
              tunnel: w435 -> [w450] mode=indexing
              tunnel: [w448] -> w438 mode=indexing
              n232 = Number To Fractional String(number=w450, precision (6)=i16 3) -> (F-format string=w448:string)  [unwired: 2 in]
            }
            n233 = Insert Into Array(array=w440, index (col)=5 ("disabled index (col)"), new element=w438) -> (w437:string[][])  [unwired: 1 in]
            n234 = local write "GainDataTable"(w437) -> ()
          }
          event Panel Close? {
            # "Discard the event because we'll close the front panel ourselves in Macro: Exit"
            # "Close Panel button (pressed) Event\n(this executes Macro: Exit to terminate the VI)"
            n235 = event-data() -> ()  [unwired: 1 in, 1 out]
            n236 = event-data ("Event Filter Node")("Discard?"=TRUE) -> ()  [unwired: 1 in, 1 out]
            n237 = call <vilib>:"Add State(s) to Queue__JKI_lib_State_Machine.vi"("State(s) in Front (\"\")"="Macro: Exit", "State(s) in (\"\")"=w456) -> ("States Out"=w455:string)  [unwired: 13 in]
          }
        }
      }
      frame "---------- Macro ----------" {
        # "Do not put any code in this frame.\n(It is a separator no-op. You can make a copy of this frame to create a new Macro frame)"
        n238 = call <vilib>:"Add State(s) to Queue__JKI_lib_State_Machine.vi"("State(s) in (\"\")"=w461) -> ("States Out"=w460:string)  [unwired: 14 in]
      }
      frame "Macro: Initialize" {
        # "load Labjack setting 1st as it contaisn laser pin infortmation"
        # "start laser 1st, need 7.5s for laser to get ready"
        # "Initialization Macro\n(This is called once, when the VI starts)"
        n239 = call <vilib>:"Add State(s) to Queue__JKI_lib_State_Machine.vi"("State(s) in Front (\"\")"="UI: showDisclaimer\nUI: Cursor Set >> Busy\nGraph: AddCursors\nData: Initialize\nInitialize Core Data\nUI: Initialize\nUI: Front Panel State >> Open\nUI: Update\nAPD: Initialize\nMacro: LoadSysConfig\nLabJack: Open\nLabJack: SetDefaultSub\nLED: OpenVIRef\nLED: BreathOrange\nUI: Update\n355 Laser: CheckControllerStatus\n355 Laser: Laser enable\n355 Laser: Dewelling>>5000\n355 Laser: CheckControllerStatus\nUI: Update\nLabJack: 355_PWM_Config\nLabJack: AB_PWM_Config\nUI: Update", "State(s) in (\"\")"="Digitizer: Initialize\nDigitizer: ConfigMacro\nUI: Update\nAimingBeam: Initialize\nAimingBeam: Set APC Status>>Disable\nAimingBeam: Set ACC Status>>Enable\nAimingBeam: Set Current\nUI: Update\nUI: Update\n355 Laser: Check Dewelling\nUtility: SetDefaultMaxV\nUI: InitIRFDataTable\nPID: loadPID\nUI: Cursor Set >> Idle\nLED: BreathOff\nMacro: SysReadyForAqui") -> ("States Out"=w462:string)  [unwired: 13 in]
        n240 = call <vilib>:"Add State(s) to Queue__JKI_lib_State_Machine.vi"("State(s) in Front (\"\")"=w462, "State(s) in (\"\")"=w470) -> ("States Out"=w469:string)  [unwired: 13 in]
        "Help" <- "Hover over controls to see help!" ("Help")
      }
      frame "Macro: LoadSysConfig" {
        # "System configuration Macro\n(Load configurations for different component of the system)"
        n241 = call <vilib>:"Add State(s) to Queue__JKI_lib_State_Machine.vi"("State(s) in Front (\"\")"="SysConfig: Load Digitizer Setting\nSysConfig: Load AB setting\nSysConfig: Load LJ Pinout\nSysConfig: Load 355 PWM\nSysConfig: Load APD Info", "State(s) in (\"\")"=w476) -> ("States Out"=w475:string)  [unwired: 13 in]
      }
      frame "Macro: StartRun" {
        # "start PWM before acquisition"
        # "Start Run Macro\n(Macro to start a aquisition run)"
        n242 = local read "Task"() -> (w478:enum32{"iRFAndGain", "Alignment"})
        n243 = case shown="\"iRFAndGain\", Default" w478 {
          tunnel: ["UI: Update\nLabJack: 355_PWM_Start\nLabJack: SetV\nDigitizer: Start\nUI: DuringAquisition\nLED: BreathGreen\nUI: Update" "UI: Update\nLabJack: SetV\nUtility: Dewelling >>250\nDigitizer: Start\nUI: DuringAquisition\nLED: BreathGreen\nUI: Update"] -> w477
          frame "iRFAndGain", Default {
          }
          frame "Alignment" {
          }
        }
        n244 = call <vilib>:"Add State(s) to Queue__JKI_lib_State_Machine.vi"("State(s) in Front (\"\")"=w477, "State(s) in (\"\")"=w483) -> ("States Out"=w482:string)  [unwired: 13 in]
      }
      frame "Macro: StopRun" {
        # "if system is running, send stop command, if not do nothing."
        # "stop aquisition\nupdate UI"
        # "Do not put any code in this frame.\n(It is a separator no-op. You can make a copy of this frame to create a new Macro frame)"
        n245 = Unbundle By Name(w486) -> ("SysRunning?"=w487:bool)
        n246 = case shown="True" w487 {
          tunnel: ["" ("Empty String Constant") w494] -> w488
          frame False {
          }
          frame True {
            n247 = local read "Task"() -> (w495:enum32{"iRFAndGain", "Alignment"})
            n248 = case shown="\"Alignment\"" w495 {
              tunnel: ["LabJack: 355_PWM_Stop" ("State(s) in Front (\"\")") "Digitizer: Abort" ("State(s) in Front (\"\")")] -> w494
              frame "iRFAndGain", Default {
                # "stop laser if taken iRF"
              }
              frame "Alignment" {
                # "do nothing if take gain"
              }
            }
          }
        }
        n249 = call <vilib>:"Add State(s) to Queue__JKI_lib_State_Machine.vi"("State(s) in Front (\"\")"=w488, "State(s) in (\"\")"=w492) -> ("States Out"=w491:string)  [unwired: 13 in]
      }
      frame "Macro: SysReadyForAqui" {
        # "System ready for aquisition macro.\n(Set UI and LED)"
        n250 = call <vilib>:"Add State(s) to Queue__JKI_lib_State_Machine.vi"("State(s) in Front (\"\")"="UI: ReadyForAquisition\nLED: Green" ("State(s) in Front (\"\")"), "State(s) in (\"\")"=w503) -> ("States Out"=w502:string)  [unwired: 13 in]
      }
      frame "Macro: AskOverWrite" {
        # "Ask user whther to over write existing APD data\n(It is a separator no-op. You can make a copy of this frame to create a new Data frame)"
        n251 = Two Button Dialog(message="Do you want to save new data? old file will be renamed as backup.", 2:"Save" ("T button name (\"OK\")")) -> (T button?=w506:bool)  [unwired: 1 in]
        n252 = case shown="True" w506 {
          tunnel: ["" ("Empty String Constant") "File: BackupOld\nAPD: SaveNew" ("State(s) in Front (\"\")")] -> w505
          frame False {
          }
          frame True {
            # "backup old file and save new file"
          }
        }
        n253 = call <vilib>:"Add State(s) to Queue__JKI_lib_State_Machine.vi"("State(s) in Front (\"\")"=w505, "State(s) in (\"\")"=w512) -> ("States Out"=w511:string)  [unwired: 13 in]
      }
      frame "Macro: Exit" {
        # "close LJ last"
        # "check whether hardware is initilized, if so close, if not do nothing"
        # "Exit Macro, close all hardware\n(This is called once, when the VI exits)"
        n254 = Unbundle By Name(w521) -> ("System Status.TCP/IP"=w520:bool, "System Status.Digitizer"=w519:bool, "System Status.Aiming Beam"=w518:bool, "System Status.355 Laser"=w517:bool, "System Status.Labjack"=w516:bool, "Core.Close Panel on Exit?"=w515:bool)
        n255 = case shown="True" w520 {
          tunnel: ["" ("Empty String Constant") ""] -> w528
          frame False {
          }
          frame True {
          }
        }
        n256 = case shown="True" w519 {
          tunnel: ["" ("Empty String Constant") "Digitizer: Close"] -> w529
          frame False {
          }
          frame True {
          }
        }
        n257 = case shown="True" w516 {
          tunnel: ["" ("Empty String Constant") "LabJack: SetDefaultAndClose"] -> w522
          frame False {
          }
          frame True {
          }
        }
        n258 = case shown="True" w518 {
          tunnel: ["" ("Empty String Constant") "AimingBeam: Set ACC Status >> Disable\nAimingBeam: Close"] -> w524
          frame False {
          }
          frame True {
          }
        }
        n259 = case shown="True" w517 {
          tunnel: ["" ("Empty String Constant") "355 Laser: Close\n355 Laser: CheckControllerStatus"] -> w523
          frame False {
          }
          frame True {
          }
        }
        n260 = Select(t="UI: Front Panel State >> Close", s=w515, f="" ("Empty String Constant")) -> (s? t:f=w525:string)
        n261 = call <vilib>:"Add State(s) to Queue__JKI_lib_State_Machine.vi"("State(s) in Front (\"\")"=w528, "State(s) in (\"\")"=w529, "State(s) at Back (\"\")"=w524) -> ("States Out"=w531:string)  [unwired: 12 in]
        n262 = call <vilib>:"Add State(s) to Queue__JKI_lib_State_Machine.vi"("State(s) in Front (\"\")"=w531, "State(s) in (\"\")"=w523, "State(s) at Back (\"\")"=w522) -> ("States Out"=w527:string)  [unwired: 12 in]
        n263 = call <vilib>:"Add State(s) to Queue__JKI_lib_State_Machine.vi"("State(s) in Front (\"\")"=w527, "State(s) in (\"\")"="UI: Update\nLED: CloseVIRef\nQueue: Destory\nData: Cleanup\nExit", "State(s) at Back (\"\")"=w525) -> ("States Out"=w532:string)  [unwired: 12 in]
        n264 = call <vilib>:"Add State(s) to Queue__JKI_lib_State_Machine.vi"("State(s) in Front (\"\")"=w532, "State(s) in (\"\")"=w537) -> ("States Out"=w536:string)  [unwired: 13 in]
      }
      frame "---------- Data ----------" {
        # "Template Separator\n(You can make a copy of, or modify, this frame)"
        n265 = call <vilib>:"Add State(s) to Queue__JKI_lib_State_Machine.vi"("State(s) in (\"\")"=w552) -> ("States Out"=w551:string)  [unwired: 14 in]
      }
      frame "Data: Initialize" {
        w555 = 0  # iRFIdx
        w557 = T23 {"CtrlV"=-1.0, "AUC"=0.0, "AUC Std"=0.0, "IntFactor"=1.0, "IntCorrAUC"=0.0}  # GainDataTemp
        w558 = dbl[][] []  # GainBGRaw
        w560 = FALSE  # LedViRefOpen
        w556 = T24 {"Ch1Serial"="", "Ch2Serial"="", "Ch3Serial"="", "Ch4Serial"=""}  # APDSerials
        w561 = cluster{"RunID":i8, "BG ID":i8, "Cali ID":i8} {"RunID"=1, "BG ID"=1, "Cali ID"=1}  # IDs
        w562 = refnum<vi> refnum  # LED vi reference
        w563 = path ""  # TempPath
        w564 = T25 {"DataPath"=path "", "BG Path"=path "", "iRFPath"=path "", "CaliPath"=path ""}  # Pathes
        w565 = u32 0  # FastTimer
        w566 = u32 0  # SlowTimer
        w567 = dbl[][] []  # iRFAllGain
        w570 = T1 {"Digitizer"=FALSE, "Labjack"=FALSE, "Aiming Beam"=FALSE, "355 Laser"=FALSE, "TCP/IP"=FALSE}  # System Status
        w554 = T26 {"DIO_EF_CLOCK1_DIVISOR"=16, "DIO_EF_CLOCK1_ROLL_VALUE"=25000, "DIO#_EF_INDEX"=0, "DIO#_EF_OPTIONS"=1, "DIO#_EF_CONFIG_A"=6250}  # AB PWM setting
        w571 = T3 {"Ch1 Bias"="TDA11", "Ch2 Bias"="DAC10", "Ch3 Bias"="DAC0", "Ch4 Bias"="DAC0", "355 PWM"="FIO0", "AimingBeam PWM"="FIO2", "Laser Ready"="FIO3", "Interlock"="FIO1", "Laser Start/Stop"="FIO1", "Red LED"="FIO1", "Green LED"="FIO1", "Foot Pedal"="DIO15"}  # LJ Pinout
        w572 = 0  # TCP attempt count
        w553 = u32 0  # Laser start tic
        w573 = refnum<k20>[] []  # niTClk sessions
        w574 = u32 0  # Last Trigger
        w575 = T26 {"DIO_EF_CLOCK1_DIVISOR"=16, "DIO_EF_CLOCK1_ROLL_VALUE"=25000, "DIO#_EF_INDEX"=0, "DIO#_EF_OPTIONS"=1, "DIO#_EF_CONFIG_A"=6250}  # 355 PWM setting
        w576 = T21 {"Aiming Beam COM Port"="COM3", "Min Current"=0.0, "Max Current"=63.0, "Default Current"=20.0, "Frequency(Hz)"=0}  # AB Cluster
        w577 = T27 {"resource name"="", "resource name 2"="", "Channel"=enum."Channel 0", "trigger source"="VAL_EXTERNAL", "trigger level"=0.5, "trigger delay"=1.35e-07, "min sample rate"=12500000000.0, "min record length"=2500, "vertical range"=1.0, "vertical offset"=-0.25, "Waveform to Avg"=2000}  # FLImDAQ
        w578 = FALSE  # SysRunning?
        w568 = path ""  # DefaultPath
        w579 = T28 {"Ch1Enable?"=FALSE, "Ch2Enable?"=FALSE, "Ch3Enable?"=FALSE, "Ch1AutoGain?"=FALSE, "Ch2AutoGain?"=FALSE, "Ch3AutoGain?"=FALSE, "AimingBeamEnable?"=FALSE}  # SysConfigCluster
        w580 = T29 {"Current VI Reference"=refnum, "Close Panel on Exit?"=FALSE}  # Core
        # "Initialize the shift-register data, here.\n(data names are defined by what you wire into the bundle function)"
        n266 = call <vilib>:"Add State(s) to Queue__JKI_lib_State_Machine.vi"("State(s) in (\"\")"=w583) -> ("States Out"=w582:string)  [unwired: 14 in]
        n267 = Bundle("Core"=w580, "SysConfigCluster"=w579, "System Status"=w570, "IDs"=w561, "DefaultPath"=w568, "Pathes"=w564, "FLImDAQ"=w577, "SysRunning?"=w578, "AB Cluster"=w576, "LJ Pinout"=w571, "355 PWM setting"=w575, "AB PWM setting"=w554, "Last Trigger"=w574, "niTClk sessions"=w573, "Laser start tic"=w553, "TCP attempt count"=w572, "iRFAllGain"=w567, "SlowTimer"=w566, "FastTimer"=w565, "TempPath"=w563, "LED vi reference"=w562, "APDSerials"=w556, "LedViRefOpen"=w560, "GainBGRaw"=w558, "GainDataTemp"=w557, "iRFIdx"=w555) -> (w559:T22)  [unwired: 1 in]
      }
      frame "Data: SignInRange" {
        # "Check Whether Signal is in Range.\n(It is a separator no-op. You can make a copy of this frame to create a new Data frame)"
        n268 = local read "Task"() -> (w584:enum32{"iRFAndGain", "Alignment"})
        n269 = case shown="\"iRFAndGain\", Default" w584 {
          frame "iRFAndGain", Default {
            n270 = local read "Tab Control"() -> (w592:T2)
            n271 = case shown="\"iRF Measureement\"" w592 {
              tunnel: 1.4 ("upper limit") -> [_ w594 w598]
              tunnel: 0.1 ("lower limit") -> [_ w593 w597]
              frame "APD1", Default {
              }
              frame "Gain Measurement" {
                n272 = local read "WF max value"() -> (w596:dbl)
                n273 = In Range and Coerce(upper limit=w594, x=w596, lower limit=w593) -> (In Range?=→"GainSigInRange":bool)  [unwired: 1 out]
              }
              frame "iRF Measureement" {
                n274 = local read "WF max value"() -> (w600:dbl)
                n275 = In Range and Coerce(upper limit=w598, x=w600, lower limit=w597) -> (In Range?=→"iRFSigInRange":bool)  [unwired: 1 out]
              }
            }
          }
          frame "Alignment" {
          }
        }
        n276 = call <vilib>:"Add State(s) to Queue__JKI_lib_State_Machine.vi"("State(s) in (\"\")"=w589) -> ("States Out"=w588:string)  [unwired: 14 in]
      }
      frame "Data: parseRunDataGain" {
        w603 = cluster{"CtrlV":dbl, "WFs":dbl[][]} {"CtrlV"=0.0, "WFs"=[]}  # GainAllCluster
        # "data individual gian"
        # "Flash data from queue and save it in structure\n()"
        n277 = Flush Queue(queue=w611, error in (no error)=w609) -> (remaining elements=w610:cluster{"WF":dbl[][]}[], error out=w605:errorcluster)  [unwired: 1 out]
        n278 = for {
          tunnel: w610 -> [w616] mode=indexing
          tunnel: [w615] -> w602 mode=concatenating
          n279 = Unbundle By Name(w616) -> ("WF"=w615:dbl[][])
        }
        n280 = local read "Ctrl V"() -> (w607:dbl)
        n281 = Bundle By Name(cluster=w603, "CtrlV"=w607, "WFs"=w602) -> (w606:cluster{"CtrlV":dbl, "WFs":dbl[][]})
        n282 = Enqueue Element(queue=w601, element=w606, error in (no error)=w605) -> (error out=w604:errorcluster)  [unwired: 1 in, 2 out]
        n283 = call <vilib>:"Add State(s) to Queue__JKI_lib_State_Machine.vi"("State(s) in (\"\")"=w614) -> ("States Out"=w613:string)  [unwired: 14 in]
      }
      frame "Data: parseRunDataiRF" {
        w618 = T8 {"CtrlV"=0.0, "WFs"=[], "WFavg"=[]}  # DataAllCluster
        # "add remove dc and normalize"
        # "update graph"
        # "data individual gian"
        # "Flash data from queue and save it in structure\n()"
        n284 = Flush Queue(queue=w632, error in (no error)=w630) -> (remaining elements=w631:cluster{"WF":dbl[][]}[], error out=w621:errorcluster)  [unwired: 1 out]
        n285 = for {
          tunnel: w631 -> [w642] mode=indexing
          tunnel: [w641] -> w625 mode=concatenating
          n286 = Unbundle By Name(w642) -> ("WF"=w641:dbl[][])
        }
        n287 = Array Size(array=w625) -> (size(s)=→"data Size":i32[])
        n288 = Transpose 2D Array(2D array=w625) -> (transposed array=w628:dbl[][])
        n289 = for {
          tunnel: w628 -> [w640] mode=indexing
          tunnel: [w639] -> w619 mode=indexing
          n290 = call-poly <vilib>:"Mean.vi"("X"=w640) -> ("mean"=w639:dbl)  [unwired: 1 out]
        }
        n291 = local read "Ctrl V"() -> (w624:dbl)
        n292 = local read "Channel"() -> (w617:enum32{"Ch1", "Ch2", "Ch3", "Ch4"})
        n293 = Bundle By Name(cluster=w618, "CtrlV"=w624, "WFs"=w625, "WFavg"=w619) -> (w622:T8)
        n294 = Build Array(w619) -> (w627:dbl[][])
        n295 = Enqueue Element(queue=w623, element=w622, error in (no error)=w621) -> (error out=w620:errorcluster)  [unwired: 1 in, 2 out]
        n296 = case shown="\"Ch3\"" w617 {
          tunnel: w627 -> [w636 w637 w638]
          frame "Ch1", Default {
            n297 = local write "Ch1 iRF Graph"(w636) -> ()
          }
          frame "Ch2" {
            n298 = local write "Ch2 iRF Graph"(w637) -> ()
          }
          frame "Ch3" {
            n299 = local write "Ch3 iRF Graph"(w638) -> ()
          }
        }
        n300 = call <vilib>:"Add State(s) to Queue__JKI_lib_State_Machine.vi"("State(s) in (\"\")"=w635) -> ("States Out"=w634:string)  [unwired: 14 in]
      }
      frame "Data: parseRunDataMacro" {
        # "Sometimes it takes some time to parse run data"
        # "Parse data macro.\n(Set curse busy, parse data, then set cursor idle)"
        n301 = local read "Task"() -> (w647:enum32{"iRFAndGain", "Alignment"})
        n302 = case shown="\"Alignment\"" w647 {
          tunnel: ["Data: parseRunDataiRF" ("State(s) in Front (\"\")") "Data: parseRunDataGain" ("State(s) in Front (\"\")")] -> w646
          frame "iRFAndGain", Default {
          }
          frame "Alignment" {
          }
        }
        n303 = call <vilib>:"Add State(s) to Queue__JKI_lib_State_Machine.vi"("State(s) in Front (\"\")"="UI: Cursor Set >> Busy" ("State(s) in Front (\"\")"), "State(s) in (\"\")"=w646, "State(s) at Back (\"\")"="UI: Cursor Set>>Idle" ("State(s) in Front (\"\")")) -> ("States Out"=w645:string)  [unwired: 12 in]
        n304 = call <vilib>:"Add State(s) to Queue__JKI_lib_State_Machine.vi"("State(s) in Front (\"\")"=w645, "State(s) in (\"\")"=w652) -> ("States Out"=w651:string)  [unwired: 13 in]
      }
      frame "Data: parseGainBGAllGain" {
        # "Parse all data for all gain\n(parse data all gain)"
        n305 = Unbundle By Name(w655) -> ("SysRunning?"=w658:bool)
        n306 = case shown="False" w658 {
          tunnel: w661 -> [w675 w687]
          tunnel: w660 -> [w674 _]
          tunnel: [w670 w687] -> w659
          tunnel: ["" ("State(s) in Front (\"\")") "Idle\nData: parseGainBGAllGain" ("State(s) in Front (\"\")")] -> w657
          tunnel: w655 -> [w672 w686]
          tunnel: [w669 w686] -> w656
          frame False {
            # "save gain BG to temp"
            n307 = Flush Queue(queue=w674, error in (no error)=w675) -> (remaining elements=w676:cluster{"CtrlV":dbl, "WFs":dbl[][]}[], error out=w670:errorcluster)  [unwired: 1 out]
            n308 = for {
              tunnel: w676 -> [w684] mode=indexing
              tunnel: [w681] -> w671 mode=indexing
              tunnel: [w682] -> w668 mode=indexing
              tunnel: [w680] -> w667 mode=indexing
              n309 = Unbundle By Name(w684) -> ("CtrlV"=w682:dbl, "WFs"=w683:dbl[][])
              n310 = for {
                tunnel: w683 -> [w685] mode=indexing
                tunnel: [w685] -> w681 mode=concatenating
              }
              n311 = call-poly <vilib>:"Mean.vi"("X"=w681) -> ("mean"=w680:dbl)  [unwired: 1 out]
            }
            n312 = local read "Channel"() -> (w666:enum32{"Ch1", "Ch2", "Ch3", "Ch4"})
            n313 = Bundle(w668, w667) -> (w665:cluster{dbl[], dbl[]})  [unwired: 1 in]
            n314 = case shown="\"Ch3\"" w666 {
              tunnel: w665 -> [w677 w678 w679]
              frame "Ch1", Default {
                n315 = local write "Ch1 Gain"(w677) -> ()
              }
              frame "Ch2" {
                n316 = local write "Ch2 Gain"(w678) -> ()
              }
              frame "Ch3" {
                n317 = local write "Ch3 Gain"(w679) -> ()
              }
            }
            n318 = Bundle By Name(cluster=w672, "GainBGRaw"=w671) -> (w669:T22)
          }
          frame True {
            # "repeat if system is running"
          }
        }
        n319 = call <vilib>:"Add State(s) to Queue__JKI_lib_State_Machine.vi"("State(s) in Front (\"\")"=w657, "State(s) in (\"\")"=w664) -> ("States Out"=w663:string)  [unwired: 13 in]
      }
      frame "Data: parseDataAllGainMacro" {
        # "Do not put any code in this frame.\n(It is a separator no-op. You can make a copy of this frame to create a new Data frame)"
        n320 = local read "Task"() -> (w690:enum32{"iRFAndGain", "Alignment"})
        n321 = case shown="\"Alignment\"" w690 {
          tunnel: ["APD: writeiRF" ("State(s) in Front (\"\")") w698] -> w689
          frame "iRFAndGain", Default {
          }
          frame "Alignment" {
            n322 = case shown="True" "BG flag?" {
              tunnel: ["APD: writeGain" ("State(s) in Front (\"\")") "Data: parseGainBGAllGain" ("State(s) in Front (\"\")")] -> w698
              frame False {
              }
              frame True {
              }
            }
          }
        }
        n323 = call <vilib>:"Add State(s) to Queue__JKI_lib_State_Machine.vi"("State(s) in Front (\"\")"=w689, "State(s) in (\"\")"=w695) -> ("States Out"=w694:string)  [unwired: 13 in]
      }
      frame "Data: parseSingleGainData" {
        # "Parse gain data for a single gain.\n(Flush data from queue, calculate peak V and std)"
        n324 = Flush Queue(queue=w724, error in (no error)=w702) -> (remaining elements=w725:cluster{"WF":dbl[][]}[], error out=w704:errorcluster)  [unwired: 1 out]
        n325 = for {
          tunnel: w725 -> [w739] mode=indexing
          tunnel: [w738] -> w723 mode=concatenating
          tunnel: [w737] -> w709 mode=concatenating
          tunnel: [w736] -> w701 mode=concatenating
          n326 = Unbundle By Name(w739) -> ("WF"=w736:dbl[][])
          n327 = for {
            tunnel: w736 -> [w742] mode=indexing
            tunnel: [w741] -> w738 mode=indexing
            tunnel: [w740] -> w737 mode=indexing
            n328 = disable-structure shown="Enabled" {
              disable-tunnel: w742 -> [w745 w751]
              disable-tunnel: [w750 w763] -> w741
              disable-tunnel: [_ w752] -> w740
              frame Disabled {
                n329 = global read "GlobalVariables.vi" "DC Idx1"() -> (w748:i32)
                n330 = global read "GlobalVariables.vi" "DC Idx2"() -> (w749:i32)
                n331 = Subtract(x=w749, y=w748) -> (x-y=w747:i32)
                n332 = Array Subset(array=w745, index=w748, length=w747) -> (w746:dbl[])
                n333 = call-poly <vilib>:"Mean.vi"("X"=w746) -> ("mean"=w744:dbl)  [unwired: 1 out]
                n334 = Subtract(x=w745, y=w744) -> (x-y=w743:dbl[])
                n335 = Array Max & Min(array=w743) -> (max value=w750:dbl)  [unwired: 3 out]
              }
              frame Enabled {
                # "Compute AUC"
                # "DC remove"
                n336 = global read "GlobalVariables.vi" "DC Idx1"() -> (w758:i32)
                n337 = global read "GlobalVariables.vi" "DC Idx2"() -> (w760:i32)
                n338 = Subtract(x=w760, y=w758) -> (x-y=w759:i32)
                n339 = Array Subset(array=w751, index=w758, length=w759) -> (w757:dbl[])
                n340 = call-poly <vilib>:"Mean.vi"("X"=w757) -> ("mean"=w756:dbl)  [unwired: 1 out]
                n341 = Subtract(x=w751, y=w756) -> (x-y=w755:dbl[])
                n342 = global read "GlobalVariables.vi" "BG Idx2"() -> (w762:i32)
                n343 = global read "GlobalVariables.vi" "BG Idx1"() -> (w761:i32)
                n344 = Subtract(x=w762, y=w761) -> (x-y=w754:i32)
                n345 = Array Subset(array=w755, index=w761, length=w754) -> (w753:dbl[])
                n346 = Array Max & Min(array=w751) -> (max value=w752:dbl)  [unwired: 3 out]
                n347 = Add Array Elements(numeric array=w753) -> (sum=w763:dbl)
              }
            }
          }
        }
        n348 = call "V1FGV.vi"("action (write)"=enum16{"write", "read"}."read") -> ("V1 out"=w706:dbl)  [unwired: 9 in, 1 out]
        n349 = Unbundle By Name(w722) -> ("GainDataTemp.IntFactor"=w712:dbl, "GainDataTemp.CtrlV"=w717:dbl, "GainDataTemp.AUC"=w714:dbl)
        n350 = Equal?(x=w706, y=w717) -> (x = y?=w716:bool)
        n351 = call <vilib>:"Std Deviation and Variance.vi"("X"=w723) -> ("mean"=w715:dbl, "standard deviation"=w719:dbl)  [unwired: 1 in, 1 out]
        n352 = call-poly <vilib>:"Mean.vi"("X"=w709) -> ("mean"=w708:dbl)  [unwired: 1 out]
        n353 = case shown="True" w716 {
          tunnel: w715 -> [_ w735]
          tunnel: w714 -> [_ w734]
          tunnel: [w730 w731] -> w713
          tunnel: w712 -> [w730 w733]
          frame False {
            # "if new Ctrl V, use old int factor"
          }
          frame True {
            # "if current CtrlV is the same as last, this is intensity change point, calculate intensity factor"
            n354 = Divide(x=w735, y=w734) -> (x/y=w732:dbl)
            n355 = Multiply(x=w733, y=w732) -> (x*y=w731:dbl)
          }
        }
        n356 = Greater?(x=w708, y=1.2) -> (0:w710:bool)
        n357 = Divide(x=w715, y=w713) -> (x/y=w718:dbl)
        n358 = Bundle By Name(cluster=w722, "GainDataTemp.CtrlV"=w706, "GainDataTemp.AUC"=w715, "GainDataTemp.AUC Std"=w719, "GainDataTemp.IntFactor"=w713, "GainDataTemp.IntCorrAUC"=w718) -> (w721:T22)
        n359 = case shown="True" w710 {
          frame False {
          }
          frame True {
            # "Inform user data near maximum"
            n360 = One Button Dialog(message="Data near threshold! Move target away and retake data at the same gain to record intensity change! ") -> ()  [unwired: 1 in, 1 out]
          }
        }
        n361 = Bundle("V1 out"=w706, "WF"=w701) -> (w705:cluster{"V1 out":dbl, "WF":dbl[][]})  [unwired: 1 in]
        n362 = Enqueue Element(queue=w707, element=w705, error in (no error)=w704) -> (error out=w703:errorcluster)  [unwired: 1 in, 2 out]
        n363 = call <vilib>:"Add State(s) to Queue__JKI_lib_State_Machine.vi"("State(s) in (\"\")"=w728) -> ("States Out"=w727:string)  [unwired: 14 in]
      }
      frame "Data: parseIRFSingleIRFData" {
        w773 = T8 {"CtrlV"=0.0, "WFs"=[], "WFavg"=[]}  # iRFDataAllCluster
        # "Parse iRF data from a single gain\n(It is a separator no-op. You can make a copy of this frame to create a new Data frame)"
        n364 = Flush Queue(queue=w780, error in (no error)=w770) -> (remaining elements=w779:cluster{"WF":dbl[][]}[], error out=w772:errorcluster)  [unwired: 1 out]
        n365 = for {
          tunnel: w779 -> [w787] mode=indexing
          tunnel: [w786] -> w775 mode=concatenating
          n366 = Unbundle By Name(w787) -> ("WF"=w786:dbl[][])
        }
        n367 = Transpose 2D Array(2D array=w775) -> (transposed array=w777:dbl[][])
        n368 = for {
          tunnel: w777 -> [w785] mode=indexing
          tunnel: [w784] -> w769 mode=indexing
          # "Average WF"
          n369 = call-poly <vilib>:"Mean.vi"("X"=w785) -> ("mean"=w784:dbl)  [unwired: 1 out]
        }
        "Current iRF" <- w769
        n370 = call "V1FGV.vi"("action (write)"=enum16{"write", "read"}."read") -> ("V1 out"=w776:dbl)  [unwired: 9 in, 1 out]
        n371 = Bundle By Name(cluster=w773, "CtrlV"=w776, "WFs"=w775, "WFavg"=w769) -> (w764:T8)
        n372 = Enqueue Element(queue=w774, element=w764, error in (no error)=w772) -> (error out=w771:errorcluster)  [unwired: 1 in, 2 out]
        n373 = Unbundle By Name(w765) -> ("iRFIdx"=w768:i32)
        n374 = Increment(x=w768) -> (x+1=w767:i32)
        n375 = Bundle By Name(cluster=w765, "iRFIdx"=w767) -> (w766:T22)
        n376 = call <vilib>:"Add State(s) to Queue__JKI_lib_State_Machine.vi"("State(s) in (\"\")"=w783) -> ("States Out"=w782:string)  [unwired: 14 in]
      }
      frame "Data: saveiRF" {
        w791 = enum16{"write", "read"}."read" ("action")
        # "Get iRF from decon stracture and save it on disk.\n(It is a separator no-op. You can make a copy of this frame to create a new Data frame)"
        n377 = Unbundle By Name(w792) -> ("TempPath"=w793:path)
        n378 = call "Ch1DeconEngineFGV.vi"("action(read)"=w791) -> ("Error Out"=w814:errorcluster, "Ch1DeconEngine out"=w815:refnum<class "LaguerreDeconEngineClass.lvclass">)  [unwired: 9 in]
        n379 = call "Ch2DeconEngineFGV.vi"("action(read)"=w791) -> ("Error Out"=w812:errorcluster, "Ch2DeconEngine out"=w813:refnum<class "LaguerreDeconEngineClass.lvclass">)  [unwired: 9 in]
        n380 = call "Ch3DeconEngineFGV.vi"("action(read)"=w791) -> ("Error Out"=w810:errorcluster, "Ch3DeconEngine out"=w811:refnum<class "LaguerreDeconEngineClass.lvclass">)  [unwired: 9 in]
        n381 = call "Ch4DeconEngineFGV.vi"("action(read)"=w791) -> ("Error Out"=w789:errorcluster, "Ch3DeconEngine out"=w790:refnum<class "LaguerreDeconEngineClass.lvclass">)  [unwired: 9 in]
        n382 = Build Path(base path=w793, name or relative path="iRF" ("default name")) -> (appended path=w808:path)
        n383 = call "getIRF.vi"("error in (no error)"=w789, "LaguerreDeconEngineClass in"=w790) -> ("iRF"=w788:dbl[])  [unwired: 7 in, 2 out]
        n384 = call "getIRF.vi"("error in (no error)"=w814, "LaguerreDeconEngineClass in"=w815) -> ("iRF"=w797:dbl[])  [unwired: 7 in, 2 out]
        n385 = call "getIRF.vi"("error in (no error)"=w812, "LaguerreDeconEngineClass in"=w813) -> ("iRF"=w796:dbl[])  [unwired: 7 in, 2 out]
        n386 = call "getIRF.vi"("error in (no error)"=w810, "LaguerreDeconEngineClass in"=w811) -> ("iRF"=w795:dbl[])  [unwired: 7 in, 2 out]
        n387 = TDMS Open(8:w807, 10:T13."create or replace" ("operation (0:open)"), 11:w808) -> (0:w804:errorcluster, 3:w805:refnum<k34>)  [unwired: 4 in]
        n388 = Build Array(w797, w796, w795, w788) -> (w803:dbl[][])
        n389 = Bundle("iRF"=w797, "iRF"=w796, "iRF"=w795, "iRF"=w788) -> (w794:T30)  [unwired: 1 in]
        n390 = global write "GlobalVariables.vi" "LastUseiRF"(w794) -> ()
        n391 = TDMS Write(0:w805, 5:"iRF" ("group name in (Untitled)"), 7:string[] ["Ch1", "Ch2", "Ch3", "Ch4"] ("channel name(s) in (Untitled)"), 9:w803, 11:w804) -> (4:w800:refnum<k34>, 15:w799:errorcluster)  [unwired: 1 in, 2 out]
        n392 = TDMS Close(8:w799, 11:w800) -> (0:w798:errorcluster)  [unwired: 1 out]
        n393 = call <vilib>:"Add State(s) to Queue__JKI_lib_State_Machine.vi"("State(s) in (\"\")"=w818) -> ("States Out"=w817:string)  [unwired: 14 in]
      }
      frame "Data: Cleanup" {
        # "Cleanup any data and references, here.\n(this is called automatically, by the Macro: Exit)"
        n394 = Unbundle By Name(w819) -> ("Core.Current VI Reference"=w820:refnum<vi>)
        n395 = Close Reference(reference=w820, error in (no error)=w823) -> (error out=w822:errorcluster)
        n396 = call <vilib>:"Add State(s) to Queue__JKI_lib_State_Machine.vi"("State(s) in (\"\")"=w825) -> ("States Out"=w824:string)  [unwired: 14 in]
      }
      frame "---------- Core ----------" {
        # "Do not put any code in this frame.\n(it is a separator no-op)"
        n397 = call <vilib>:"Add State(s) to Queue__JKI_lib_State_Machine.vi"("State(s) in (\"\")"=w830) -> ("States Out"=w829:string)  [unwired: 14 in]
      }
      frame Default {
        w841 = 42 items=["No error", "Argument error", "Memory is full", "Out of zone", "End of file", "File already open", "Generic file I/O error", "File not found", "File permission error", "Disk is full", "Duplicate path", "Too many files open", "System feature not enabled", "Resource file not found", "Cannot add resource", "Resource not found", "Image not found", "Image memory error", "Pen does not exist", "Config type invalid", "Config token not found", "Config parse error", "Config memory error", "Bad external code format", "Bad external code offset", "External code not present", "Null window", "Destroy window error", "Null menu", "Print aborted", "Bad print record", "Print driver error", "Windows error during printing", "Memory error during printing", "Print dialog error", "Generic print error", "Invalid device refnum", "Device not found", "Device parameter error", "Device unit error", "Cannot open device", "Device call aborted", "Generic error", "Cancelled by user", "Object ID too low", "Object ID too high", "Object not in heap", "Unknown heap", "Unknown object (invalid DefProc)", "Unknown object (DefProc not in table)", "Message out of range", "Invalid (null) method", "Unknown message", "Manager call not supported", "Bad address", "Network operation in progress", "Network operation timed out", "Connection is busy", "Network attribute not supported", "Network error", "Address in use", "System out of memory", "Connection aborted", "Connection refused", "Not connected", "Already connected", "Connection closed", "Initialization error (interapplication manager)", "Bad occurrence", "Wait on unbound occurrence handler", "Occurrence queue overflow", "Datalog type conflict", "Unused", "Unrecognized type (interapplication manager)", "Memory corrupt", "Failed to make temporary DLL", "Old CIN version", "Drag socket not found", "Failed to load drop-object", "Failed to register OLE object", "Failed to release OLE object", "Format specifier type mismatch", "Unknown format specifier", "Too few format specifiers", "Too many format specifiers", "Scan failed", "Newer CIN version", "Error converting to variant", "Runtime menu error", "Password tampered", "Variant attribute not found", "Incompatible variant data type", "Event data is not available", "Event Store is not present", "Occurrence is not found", "Event Queue is not created", "Event info is not available", "Refnum passed is NULL", "Error retrieving Class GUID", "Error retrieving CoClass GUID", "Error retrieving TypeLib GUID.", "Bad built application magic bytes.", "Specific driver is different from the specific driver associated with the Logical Name.", "There is no session opened to the class driver.", "Max Error", "MAX - Error with config objects", "MAX - Error loading configuration", "MAX - Group not supported"]
        # "Current State"
        # "Do not delete, rename, or modify this frame.\n(this is used to capture unhandled states and typos)"
        # "Handle mistyped state name (developer tool)"
        n398 = Format Into String(format string="Software Exception: Unhandled State \"%s\"." ("message"), error in=w837, w832) -> (resulting string=w840:string, error out=w839:errorcluster)  [unwired: 1 in]
        n399 = call <vilib>:"Error Cluster From Error Code.vi"("show call chain? (False)"=TRUE, "error in (no error)"=w839, "error message (\"\")"=w840, "error code (0)"=w841) -> ("error out"=w838:errorcluster)  [unwired: 5 in]
        n400 = call <vilib>:"Add State(s) to Queue__JKI_lib_State_Machine.vi"("State(s) in (\"\")"=w836) -> ("States Out"=w835:string)  [unwired: 14 in]
      }
      frame "Initialize Core Data" {
        # "Build default path based on the location of project"
        # "Do not delete, rename, or modify this frame.\n(this is used to determine panel behavior on exit)"
        # "originally closed?"
        # "exe?"
        # "If panel starts closed or is an EXE, then close it when we exit"
        n401 = call <vilib>:"Application Directory.vi"() -> ("Application Directory"=w845:path)
        n402 = property on="Property Node" class="App"() -> ("App.Kind"=w858:T15)  [unwired: 2 in, 2 out]
        n403 = property on="Property Node" class="VI"() -> ("FP.State"=w853:T14)  [unwired: 2 in, 2 out]
        n404 = control-ref of="Current VI Reference"() -> (w854:refnum<vi>)
        n405 = Equal?(x=w853, y=T14."Closed" ("Front Panel Window:State")) -> (x = y?=w851:bool)
        n406 = Equal?(x=w858, y=T15."Run Time System" ("Application:Kind")) -> (x = y?=w856:bool)
        n407 = Build Path(base path=w845, name or relative path="Data") -> (appended path=w849:path)
        n408 = Build Path(base path=w845, name or relative path="SystemTemp") -> (appended path=w846:path)
        n409 = Or(x=w851, y=w856) -> (x .or. y?=w855:bool)
        n410 = Bundle By Name(cluster=w844, "Core.Current VI Reference"=w854, "Core.Close Panel on Exit?"=w855, "DefaultPath"=w849, "TempPath"=w846) -> (w843:T22)
        n411 = call <vilib>:"Add State(s) to Queue__JKI_lib_State_Machine.vi"("State(s) in (\"\")"=w861) -> ("States Out"=w860:string)  [unwired: 14 in]
      }
      frame "Error Handler" {
        # "Unhandled Error -- Display it"
        # "Handle any errors here.\nYou can also output any states to clean-up after errors occur"
        # "Clear error"
        n412 = Unbundle By Name(w862) -> ("code"=w864:i32)
        n413 = case shown="5005" w864 {
          tunnel: ["Macro: Exit" w874 w880 ""] -> w863
          tunnel: w862 -> [w870 _ _ _]
          frame Default {
            w872 = T31 1 items=["no dialog", "OK message", "continue or stop message", "OK message + warnings", "continue/stop + warnings"] ("type of dialog (OK msg:1)")
            n414 = call <vilib>:"General Error Handler.vi"("type of dialog (OK msg:1)"=w872, "error in (no error)"=w870) -> ()  [unwired: 9 in, 5 out]
          }
          frame 5002 {
            n415 = Two Button Dialog(message="Laser interlock open! Please close interlock and try again! ", 1:"Safely Shutdown" ("F button name (\"Cancel\")"), 2:"OK" ("T button name (\"OK\")")) -> (T button?=w875:bool)
            n416 = case shown="True" w875 {
              tunnel: ["Macro: Exit" "355 Laser: CheckControllerStatus"] -> w874
              frame False {
              }
              frame True {
              }
            }
          }
          frame 5001 {
            n417 = Two Button Dialog(message="Unable to connect to imaging computer, do you want to run data aquisiton along? ", 1:"No" ("F button name (\"Cancel\")"), 2:"Yes" ("T button name (\"OK\")")) -> (T button?=w881:bool)
            n418 = case shown="True" w881 {
              tunnel: ["Macro: Exit" "" ("Empty String Constant")] -> w880
              frame False {
              }
              frame True {
              }
            }
          }
          frame 5005 {
          }
        }
        n419 = call <vilib>:"Add State(s) to Queue__JKI_lib_State_Machine.vi"("State(s) in Front (\"\")"=w863, "State(s) in (\"\")"=w869) -> ("States Out"=w868:string)  [unwired: 13 in]
      }
      frame "Exit" {
        # "Do not put any code in this frame.\n(No errors that occur here will be handled.)"
        n420 = call <vilib>:"Add State(s) to Queue__JKI_lib_State_Machine.vi"("State(s) in (\"\")"=w893) -> ("States Out"=w892:string)  [unwired: 14 in]
      }
      frame "---------- AimingBeam ----------" {
        # "Template Separator\n(You can make a copy of, or modify, this frame)"
        n421 = call <vilib>:"Add State(s) to Queue__JKI_lib_State_Machine.vi"("State(s) in (\"\")"=w898) -> ("States Out"=w897:string)  [unwired: 14 in]
      }
      frame "AimingBeam: Initialize" {
        # "set aiming beam button color"
        # "Open COM port for Aiming Beam\n(Require USB connection)"
        n422 = Unbundle By Name(w900) -> ("AB Cluster.Aiming Beam COM Port"=w899:refnum<visa-resource-name>)
        n423 = call-poly "VISA Configure Serial Port"("VISA resource name"=w899, "Enable Termination\nChar (T)"=TRUE ("Enable Termination\nChar (T)"), "baud rate (9600)"=u32 9600, "error in (no error)"=w906) -> ("error out"=w905:errorcluster)  [unwired: 10 in, 1 out]
        n424 = Unbundle By Name(w905) -> ("status"=w904:bool)
        n425 = Not(x=w904) -> (.not. x?=w903:bool)
        n426 = Bundle By Name(cluster=w900, "System Status.Aiming Beam"=w903) -> (w901:T22)
        n427 = call <vilib>:"Add State(s) to Queue__JKI_lib_State_Machine.vi"("State(s) in (\"\")"=w910) -> ("States Out"=w909:string)  [unwired: 14 in]
      }
      frame "AimingBeam: Close" {
        # "Close Aiming Beam COM port\n(Require USB connection to Aiming Beam Laser)"
        n428 = Unbundle By Name(w912) -> ("AB Cluster.Aiming Beam COM Port"=w913:refnum<visa-resource-name>)
        n429 = VISA Close(VISA resource name=w913, error in (no error)=w916) -> (error out=w917:errorcluster)
        n430 = Bundle By Name(cluster=w912, "System Status.Aiming Beam"=FALSE) -> (w911:T22)
        n431 = call <vilib>:"Add State(s) to Queue__JKI_lib_State_Machine.vi"("State(s) in (\"\")"=w919) -> ("States Out"=w918:string)  [unwired: 14 in]
      }
      frame "AimingBeam: Set Current" {
        # "Set Aiming Beam Current\n(You can make a copy of, or modify, this frame)"
        n432 = Unbundle By Name(w921) -> ("AB Cluster.Aiming Beam COM Port"=w920:refnum<visa-resource-name>, "AB Cluster.Max Current"=w925:dbl, "AB Cluster.Default Current"=w924:dbl, "AB Cluster.Min Current"=w923:dbl)
        n433 = In Range and Coerce(upper limit=w925, x=w924, lower limit=w923) -> (coerced(x)=w922:dbl)  [unwired: 1 out]
        n434 = local write "Current"(w922) -> ()
        n435 = Number To Fractional String(number=w922, precision (6)=i16 2) -> (F-format string=w929:string)  [unwired: 2 in]
        n436 = Concatenate Strings("slc:", w929, "\r" ("Carriage Return Constant"), "\n" ("Line Feed Constant")) -> (w932:string)
        n437 = VISA Write(VISA resource name=w920, write buffer=w932, error in (no error)=w927) -> (error out=w928:errorcluster)  [unwired: 2 out]
        n438 = call <vilib>:"Add State(s) to Queue__JKI_lib_State_Machine.vi"("State(s) in (\"\")"=w936) -> ("States Out"=w935:string)  [unwired: 14 in]
      }
      frame "AimingBeam: Set ACC Status" {
        # "Enable Aiming Beam\n(Usage: \"AimingBeam: Set >> Enable|Disable\")"
        n439 = Unbundle By Name(w937) -> ("AB Cluster.Aiming Beam COM Port"=w938:refnum<visa-resource-name>)
        n440 = case shown="\"Enable\"" w943 {
          tunnel: [w945 w949] -> w942
          frame "Disable", Default {
            n441 = Concatenate Strings("cof", "\r" ("Carriage Return Constant"), "\n" ("Line Feed Constant")) -> (w945:string)
          }
          frame "Enable" {
            n442 = Concatenate Strings("con", "\r" ("Carriage Return Constant"), "\n" ("Line Feed Constant")) -> (w949:string)
          }
        }
        n443 = VISA Write(VISA resource name=w938, write buffer=w942, error in (no error)=w940) -> (error out=w941:errorcluster)  [unwired: 2 out]
      }
      frame "AimingBeam: Set APC Status" {
        # "Enable Aiming Beam\n(Usage: \"AimingBeam: Set >> Enable|Disable\")"
        n444 = Unbundle By Name(w953) -> ("AB Cluster.Aiming Beam COM Port"=w954:refnum<visa-resource-name>)
        n445 = case shown="\"Disable\", Default" w959 {
          tunnel: [w961 w965] -> w958
          frame "Disable", Default {
            n446 = Concatenate Strings("lof", "\r" ("Carriage Return Constant"), "\n" ("Line Feed Constant")) -> (w961:string)
          }
          frame "Enable" {
            n447 = Concatenate Strings("lon", "\r" ("Carriage Return Constant"), "\n" ("Line Feed Constant")) -> (w965:string)
          }
        }
        n448 = VISA Write(VISA resource name=w954, write buffer=w958, error in (no error)=w956) -> (error out=w957:errorcluster)  [unwired: 2 out]
      }
      frame "AimingBeam: GetPWMStatus" {
        # "Get aiming beam PWM status\n()"
        n449 = local read "AB Rep Rate"() -> (w970:u16)
        n450 = Greater Than 0?(x=w970) -> (x > 0?=w969:bool)
        n451 = case shown="True" w969 {
          tunnel: w973 -> [w977 w982]
          tunnel: w972 -> [_ w981]
          tunnel: [w977 w980] -> w971
          frame False {
          }
          frame True {
            n452 = Unbundle By Name(w981) -> ("LJ Pinout.AimingBeam PWM"=w978:string)
            n453 = call "LabJack_FGV.vi"("Operation(Read)"=enum16{"Write", "Read"}."Read" ("Operation"), "error in (no error)"=w982) -> ("error out"=w985:errorcluster, "Read data"=w986:i32)  [unwired: 8 in]
            n454 = Concatenate Strings(w978, "_EF_ENABLE" ("string")) -> (w984:string)
            n455 = call "LJM_eReadName.vi"("Handle In"=w986, "Name"=w984, "error in"=w985) -> ("Value"=w983:dbl, "error out"=w980:errorcluster)  [unwired: 10 in, 1 out]
            n456 = Greater Than 0?(x=w983) -> (x > 0?=w979:bool)
            n457 = case shown="True" w979 {
              frame False {
                # "PWM is off\nset color to gray"
                n458 = local write "Aiming beam toggle"(FALSE ("Aimging beam")) -> ()
              }
              frame True {
                # "PWM is on\nset color to light green"
                n459 = local write "Aiming beam toggle"(TRUE ("Aimging beam")) -> ()
              }
            }
          }
        }
        n460 = call <vilib>:"Add State(s) to Queue__JKI_lib_State_Machine.vi"("State(s) in (\"\")"=w976) -> ("States Out"=w975:string)  [unwired: 14 in]
      }
      frame "AimingBeam: ComputePWM" {
        # "Compute PWM parameter based on AB frequency\n(You can make a copy of, or modify, this frame)"
        n461 = Unbundle By Name(w992) -> ("AB Cluster.Frequency(Hz)"=w991:i32)
        n462 = call "LJ_calculate_PWM_parameters.vi"("Duty Cycle (%)"="Duty Cycle (%)", "Error In"=w993, "Show Confirmation"=FALSE, "Laser Rep Rate (Hz)"=w991, "Laser"=enum16{"355nm", "AimingBeam"}."AimingBeam") -> ("Error Out"=w994:errorcluster)  [unwired: 5 in, 1 out]
        n463 = call <vilib>:"Add State(s) to Queue__JKI_lib_State_Machine.vi"("State(s) in (\"\")"=w1000) -> ("States Out"=w999:string)  [unwired: 14 in]
      }
      frame "---------- Digitizer ----------" {
        # "Template Separator\n(You can make a copy of, or modify, this frame)"
        n464 = call <vilib>:"Add State(s) to Queue__JKI_lib_State_Machine.vi"("State(s) in (\"\")"=w1005) -> ("States Out"=w1004:string)  [unwired: 14 in]
      }
      frame "Digitizer: ConfigMacro" {
        # "Digitizer Configuration Macro\n(Decide how to config digitizer)"
        n465 = case shown="\"iRFAndGain\", Default" "Task" {
          tunnel: "Channel" -> [w1017 w1023]
          tunnel: [w1016 w1022] -> w1008
          frame "iRFAndGain", Default {
            n466 = case shown="\"Ch4\"" w1017 {
              tunnel: ["Digitizer: ConfigCh1iRF" ("State(s) at Back (\"\")") "Digitizer: ConfigCh2iRF" ("State(s) at Back (\"\")") "Digitizer: ConfigCh3iRF" ("State(s) at Back (\"\")") "Digitizer: ConfigCh4iRF" ("State(s) at Back (\"\")")] -> w1016
              frame "Ch1", Default {
              }
              frame "Ch2" {
              }
              frame "Ch3" {
              }
              frame "Ch4" {
              }
            }
          }
          frame "Alignment" {
            n467 = case shown="\"Ch4\"" w1023 {
              tunnel: ["Digitizer: ConfigCh1Align" ("State(s) at Back (\"\")") "Digitizer: ConfigCh2Align" ("State(s) at Back (\"\")") "Digitizer: ConfigCh3Align" ("State(s) at Back (\"\")") "Digitizer: ConfigCh4Align" ("State(s) at Back (\"\")")] -> w1022
              frame "Ch1", Default {
              }
              frame "Ch2" {
              }
              frame "Ch3" {
              }
              frame "Ch4" {
              }
            }
          }
        }
        n468 = call <vilib>:"Add State(s) to Queue__JKI_lib_State_Machine.vi"("State(s) in Front (\"\")"=w1008, "State(s) in (\"\")"="Graph: SetXScale\nGraph: ClearHistory\nMacro: SysReadyForAqui" ("State(s) in (\"\")")) -> ("States Out"=w1006:string)  [unwired: 13 in]
        n469 = call <vilib>:"Add State(s) to Queue__JKI_lib_State_Machine.vi"("State(s) in Front (\"\")"=w1006, "State(s) in (\"\")"=w1015) -> ("States Out"=w1014:string)  [unwired: 13 in]
      }
      frame "Digitizer: Initialize" {
        # "Initialize digitizer.\nInitialize both digitizer and update status."
        n470 = call "FLImDAQ_FGV.vi"("error in (no error)"=w1034) -> ("error out"=w1028:errorcluster, "Read data"=w1033:T4)  [unwired: 9 in]
        n471 = property on="Digitizer" class="Bool (strict)"("Blinking"=TRUE) -> ()  [unwired: 2 in, 2 out]
        n472 = Unbundle By Name(w1033) -> ("Digitizer 1"=w1032:refnum<k15>, "Digitizer 2"=w1031:refnum<k15>)
        n473 = case shown="No Error" w1028 {
          selector: w1028 -> [w1041 w1045]
          tunnel: [w1044 w1045] -> w1036
          tunnel: w1031 -> [w1043 _]
          frame No Error {
            n474 = call <instrlib>:"niScope Initialize.vi"("resource name"=w1043, "reset device"=FALSE, "error in"=w1041) -> ("error out"=w1044:errorcluster)  [unwired: 11 in, 1 out]
          }
          frame Error {
          }
        }
        n475 = case shown="No Error" w1028 {
          selector: w1028 -> [w1047 w1050]
          tunnel: w1032 -> [w1049 _]
          tunnel: [w1046 w1050] -> w1029
          frame No Error {
            n476 = call <instrlib>:"niScope Initialize.vi"("resource name"=w1049, "reset device"=FALSE, "error in"=w1047) -> ("error out"=w1046:errorcluster)  [unwired: 11 in, 1 out]
          }
          frame Error {
          }
        }
        n477 = Merge Errors(w1029, w1036) -> (w1035:errorcluster)
        n478 = call <vilib>:"Add State(s) to Queue__JKI_lib_State_Machine.vi"("State(s) in (\"\")"=w1040) -> ("States Out"=w1039:string)  [unwired: 14 in]
      }
      frame "Digitizer: ConfigCh1iRF" {
        # "Synchronize is taking time ~3s."
        # "Config  digitizer\nCall subVi to config digitizer"
        n479 = Unbundle By Name(w1052) -> ("FLImDAQ"=w1053:T27)
        n480 = call "FLImDAQ_FGV.vi"() -> ("Read data"=w1059:T4)  [unwired: 10 in, 1 out]
        n481 = property on="Digitizer" class="Bool (strict)"(error in=w1062, "Blinking"=TRUE) -> (error out=w1057:errorcluster)  [unwired: 1 in, 1 out]
        n482 = Unbundle By Name(w1059) -> ("Digitizer 1"=w1061:refnum<k15>)
        n483 = Bundle By Name(cluster=w1053, "Channel"=enum16{"Channel 0", "Channel 1", "Channel 0&1"}."Channel 0") -> (w1055:T27)
        n484 = case shown="No Error" w1057 {
          selector: w1057 -> [w1070 w1073]
          tunnel: w1055 -> [w1069 _]
          tunnel: [w1072 w1073] -> w1056
          tunnel: w1061 -> [w1071 _]
          frame No Error {
            n485 = call "DigitizerConfig.vi"("error in (no error)"=w1070, "FLImDAQ"=w1069, "IVI Refnum in"=w1071) -> ("error out"=w1072:errorcluster)  [unwired: 7 in, 1 out]
          }
          frame Error {
          }
        }
        n486 = Unbundle By Name(w1056) -> ("status"=w1065:bool)
        n487 = property on="Digitizer" class="Bool (strict)"(error in=w1056, "Blinking"=FALSE) -> (error out=w1060:errorcluster)  [unwired: 1 in, 1 out]
        n488 = Not(x=w1065) -> (.not. x?=w1064:bool)
        n489 = Bundle By Name(cluster=w1052, "System Status.Digitizer"=w1064) -> (w1051:T22)
        n490 = call <vilib>:"Add State(s) to Queue__JKI_lib_State_Machine.vi"("State(s) in (\"\")"=w1068) -> ("States Out"=w1067:string)  [unwired: 14 in]
      }
      frame "Digitizer: ConfigCh2iRF" {
        # "Synchronize is taking time ~3s."
        # "Config  digitizer\nCall subVi to config digitizer"
        n491 = Unbundle By Name(w1075) -> ("FLImDAQ"=w1076:T27)
        n492 = call "FLImDAQ_FGV.vi"() -> ("Read data"=w1082:T4)  [unwired: 10 in, 1 out]
        n493 = property on="Digitizer" class="Bool (strict)"(error in=w1085, "Blinking"=TRUE) -> (error out=w1080:errorcluster)  [unwired: 1 in, 1 out]
        n494 = Unbundle By Name(w1082) -> ("Digitizer 1"=w1084:refnum<k15>)
        n495 = Bundle By Name(cluster=w1076, "Channel"=enum16{"Channel 0", "Channel 1", "Channel 0&1"}."Channel 1") -> (w1078:T27)
        n496 = case shown="No Error" w1080 {
          selector: w1080 -> [w1093 w1096]
          tunnel: w1078 -> [w1092 _]
          tunnel: [w1095 w1096] -> w1079
          tunnel: w1084 -> [w1094 _]
          frame No Error {
            n497 = call "DigitizerConfig.vi"("error in (no error)"=w1093, "FLImDAQ"=w1092, "IVI Refnum in"=w1094) -> ("error out"=w1095:errorcluster)  [unwired: 7 in, 1 out]
          }
          frame Error {
          }
        }
        n498 = Unbundle By Name(w1079) -> ("status"=w1088:bool)
        n499 = property on="Digitizer" class="Bool (strict)"(error in=w1079, "Blinking"=FALSE) -> (error out=w1083:errorcluster)  [unwired: 1 in, 1 out]
        n500 = Not(x=w1088) -> (.not. x?=w1087:bool)
        n501 = Bundle By Name(cluster=w1075, "System Status.Digitizer"=w1087) -> (w1074:T22)
        n502 = call <vilib>:"Add State(s) to Queue__JKI_lib_State_Machine.vi"("State(s) in (\"\")"=w1091) -> ("States Out"=w1090:string)  [unwired: 14 in]
      }
      frame "Digitizer: ConfigCh3iRF" {
        # "Hardcode channel to 0, which is Ch1 and Ch3."
        # "Synchronize is taking time ~3s."
        # "Config  digitizer\nCall subVi to config digitizer"
        n503 = Unbundle By Name(w1100) -> ("FLImDAQ"=w1101:T27)
        n504 = call "FLImDAQ_FGV.vi"() -> ("Read data"=w1125:T4)  [unwired: 10 in, 1 out]
        n505 = Bundle By Name(cluster=w1101, "Channel"=enum16{"Channel 0", "Channel 1", "Channel 0&1"}."Channel 0") -> (w1102:T27)
        n506 = Unbundle By Name(w1125) -> ("Digitizer 1"=w1128:refnum<k15>, "Digitizer 2"=w1127:refnum<k15>)
        n507 = property on="Digitizer" class="Bool (strict)"(error in=w1129, "Blinking"=TRUE) -> (error out=w1105:errorcluster)  [unwired: 1 in, 1 out]
        n508 = case shown="No Error" w1105 {
          selector: w1105 -> [w1145 w1148]
          tunnel: w1102 -> [w1144 _]
          tunnel: [w1147 w1148] -> w1104
          tunnel: w1128 -> [w1146 _]
          frame No Error {
            n509 = call "DigitizerConfig.vi"("error in (no error)"=w1145, "FLImDAQ"=w1144, "IVI Refnum in"=w1146) -> ("error out"=w1147:errorcluster)  [unwired: 7 in, 1 out]
          }
          frame Error {
          }
        }
        n510 = case shown="No Error" w1104 {
          selector: w1104 -> [w1138 w1143]
          tunnel: w1102 -> [w1137 _]
          tunnel: [w1141 w1143] -> w1111
          tunnel: w1127 -> [w1139 w1142]
          tunnel: [w1136 w1142] -> w1098
          frame No Error {
            n511 = call "DigitizerConfig.vi"("Config Trigger? (T)"=FALSE ("Config Trigge(T)r:"), "error in (no error)"=w1138, "FLImDAQ"=w1137, "IVI Refnum in"=w1139) -> ("error out"=w1141:errorcluster, "IVI Refnum out"=w1136:refnum<k15>)  [unwired: 6 in]
          }
          frame Error {
          }
        }
        n512 = call "Digitizer1_FGV.vi"("error in (no error)"=w1111, "Operation (Read)"=enum16{"Write", "Read"}."Read" ("Operation")) -> ("error out"=w1122:errorcluster, "Read data"=w1123:refnum<k15>)  [unwired: 8 in]
        n513 = call <instrlib>:"niScope Get Session Reference.vi"("instrument handle"=w1123, "error in"=w1122) -> ("session reference"=w1115:refnum<k20>, "error out"=w1113:errorcluster)  [unwired: 11 in, 1 out]
        n514 = call "Digitizer2_FGV.vi"("error in (no error)"=w1113, "Operation (Read)"=enum16{"Write", "Read"}."Read" ("Operation")) -> ("error out"=w1119:errorcluster, "Read data"=w1120:refnum<k15>)  [unwired: 8 in]
        n515 = call <instrlib>:"niScope Get Session Reference.vi"("instrument handle"=w1120, "error in"=w1119) -> ("session reference"=w1114:refnum<k20>, "error out"=w1112:errorcluster)  [unwired: 11 in, 1 out]
        n516 = Build Array(w1115, w1114) -> (w1118:refnum<k20>[])
        n517 = property class="niScope"(reference=w1098) -> ("Trigger Delay"=→"Triggering:Trigger Delay":dbl)  [unwired: 1 in, 2 out]
        n518 = call <instrlib>:"niTClk Configure For Homogeneous Triggers.vi"("error in (no error)"=w1112, "sessions"=w1118) -> ("error out"=w1117:errorcluster, "sessions out"=w1116:refnum<k20>[])  [unwired: 8 in]
        n519 = call <instrlib>:"niTClk Synchronize.vi"("error in (no error)"=w1117, "sessions"=w1116) -> ("error out"=w1110:errorcluster, "sessions out"=w1107:refnum<k20>[])  [unwired: 8 in]
        n520 = call <userlib>:"Wait (ms)__ogtk.vi"("error in (no error)"=w1110, "milliseconds to wait"=u32 1500) -> ("error out"=w1109:errorcluster)  [unwired: 8 in, 1 out]
        n521 = Unbundle By Name(w1109) -> ("status"=w1132:bool)
        n522 = Not(x=w1132) -> (.not. x?=w1131:bool)
        n523 = Bundle By Name(cluster=w1100, "System Status.Digitizer"=w1131, "niTClk sessions"=w1107) -> (w1099:T22)
        n524 = property on="Digitizer" class="Bool (strict)"(error in=w1109, "Blinking"=FALSE) -> (error out=w1126:errorcluster)  [unwired: 1 in, 1 out]
        n525 = call <vilib>:"Add State(s) to Queue__JKI_lib_State_Machine.vi"("State(s) in (\"\")"=w1135) -> ("States Out"=w1134:string)  [unwired: 14 in]
      }
      frame "Digitizer: ConfigCh4iRF" {
        # "Hardcode channel to 0, which is Ch2 and Ch4."
        # "Synchronize is taking time ~3s."
        # "Config  digitizer\nCall subVi to config digitizer"
        n526 = Unbundle By Name(w1152) -> ("FLImDAQ"=w1153:T27)
        n527 = call "FLImDAQ_FGV.vi"() -> ("Read data"=w1177:T4)  [unwired: 10 in, 1 out]
        n528 = Bundle By Name(cluster=w1153, "Channel"=enum16{"Channel 0", "Channel 1", "Channel 0&1"}."Channel 1") -> (w1154:T27)
        n529 = Unbundle By Name(w1177) -> ("Digitizer 1"=w1180:refnum<k15>, "Digitizer 2"=w1179:refnum<k15>)
        n530 = property on="Digitizer" class="Bool (strict)"(error in=w1181, "Blinking"=TRUE) -> (error out=w1157:errorcluster)  [unwired: 1 in, 1 out]
        n531 = case shown="No Error" w1157 {
          selector: w1157 -> [w1197 w1200]
          tunnel: w1154 -> [w1196 _]
          tunnel: [w1199 w1200] -> w1156
          tunnel: w1180 -> [w1198 _]
          frame No Error {
            n532 = call "DigitizerConfig.vi"("error in (no error)"=w1197, "FLImDAQ"=w1196, "IVI Refnum in"=w1198) -> ("error out"=w1199:errorcluster)  [unwired: 7 in, 1 out]
          }
          frame Error {
          }
        }
        n533 = case shown="No Error" w1156 {
          selector: w1156 -> [w1190 w1195]
          tunnel: w1154 -> [w1189 _]
          tunnel: [w1193 w1195] -> w1163
          tunnel: w1179 -> [w1191 w1194]
          tunnel: [w1188 w1194] -> w1150
          frame No Error {
            n534 = call "DigitizerConfig.vi"("Config Trigger? (T)"=FALSE ("Config Trigge(T)r:"), "error in (no error)"=w1190, "FLImDAQ"=w1189, "IVI Refnum in"=w1191) -> ("error out"=w1193:errorcluster, "IVI Refnum out"=w1188:refnum<k15>)  [unwired: 6 in]
          }
          frame Error {
          }
        }
        n535 = call "Digitizer1_FGV.vi"("error in (no error)"=w1163, "Operation (Read)"=enum16{"Write", "Read"}."Read" ("Operation")) -> ("error out"=w1174:errorcluster, "Read data"=w1175:refnum<k15>)  [unwired: 8 in]
        n536 = call <instrlib>:"niScope Get Session Reference.vi"("instrument handle"=w1175, "error in"=w1174) -> ("session reference"=w1167:refnum<k20>, "error out"=w1165:errorcluster)  [unwired: 11 in, 1 out]
        n537 = call "Digitizer2_FGV.vi"("error in (no error)"=w1165, "Operation (Read)"=enum16{"Write", "Read"}."Read" ("Operation")) -> ("error out"=w1171:errorcluster, "Read data"=w1172:refnum<k15>)  [unwired: 8 in]
        n538 = call <instrlib>:"niScope Get Session Reference.vi"("instrument handle"=w1172, "error in"=w1171) -> ("session reference"=w1166:refnum<k20>, "error out"=w1164:errorcluster)  [unwired: 11 in, 1 out]
        n539 = Build Array(w1167, w1166) -> (w1170:refnum<k20>[])
        n540 = property class="niScope"(reference=w1150) -> ("Trigger Delay"=w1149:dbl)  [unwired: 1 in, 2 out]
        n541 = call <instrlib>:"niTClk Configure For Homogeneous Triggers.vi"("error in (no error)"=w1164, "sessions"=w1170) -> ("error out"=w1169:errorcluster, "sessions out"=w1168:refnum<k20>[])  [unwired: 8 in]
        n542 = call <instrlib>:"niTClk Synchronize.vi"("error in (no error)"=w1169, "sessions"=w1168) -> ("error out"=w1162:errorcluster, "sessions out"=w1159:refnum<k20>[])  [unwired: 8 in]
        n543 = call <userlib>:"Wait (ms)__ogtk.vi"("error in (no error)"=w1162, "milliseconds to wait"=u32 1500) -> ("error out"=w1161:errorcluster)  [unwired: 8 in, 1 out]
        n544 = Unbundle By Name(w1161) -> ("status"=w1184:bool)
        n545 = Not(x=w1184) -> (.not. x?=w1183:bool)
        n546 = Bundle By Name(cluster=w1152, "System Status.Digitizer"=w1183, "niTClk sessions"=w1159) -> (w1151:T22)
        n547 = property on="Digitizer" class="Bool (strict)"(error in=w1161, "Blinking"=FALSE) -> (error out=w1178:errorcluster)  [unwired: 1 in, 1 out]
        n548 = local write "Triggering:Trigger Delay"(w1149) -> ()
        n549 = call <vilib>:"Add State(s) to Queue__JKI_lib_State_Machine.vi"("State(s) in (\"\")"=w1187) -> ("States Out"=w1186:string)  [unwired: 14 in]
      }
      frame "Digitizer: ConfigCh1Align" {
        # "Synchronize is taking time ~3s."
        # "Config  digitizer\nCall subVi to config digitizer"
        n550 = Unbundle By Name(w1203) -> ("FLImDAQ"=w1204:T27)
        n551 = call "FLImDAQ_FGV.vi"() -> ("Read data"=w1209:T4)  [unwired: 10 in, 1 out]
        n552 = property on="Digitizer" class="Bool (strict)"(error in=w1212, "Blinking"=TRUE) -> (error out=w1207:errorcluster)  [unwired: 1 in, 1 out]
        n553 = Unbundle By Name(w1209) -> ("Digitizer 1"=w1211:refnum<k15>)
        n554 = Bundle By Name(cluster=w1204, "Channel"=enum16{"Channel 0", "Channel 1", "Channel 0&1"}."Channel 0") -> (w1201:T27)
        n555 = case shown="No Error" w1207 {
          selector: w1207 -> [w1220 w1223]
          tunnel: w1201 -> [w1219 _]
          tunnel: [w1222 w1223] -> w1206
          tunnel: w1211 -> [w1221 _]
          frame No Error {
            n556 = call "DigitizerConfigGain.vi"("error in (no error)"=w1220, "FLImDAQ"=w1219, "IVI Refnum in"=w1221) -> ("error out"=w1222:errorcluster)  [unwired: 7 in, 1 out]
          }
          frame Error {
          }
        }
        n557 = Unbundle By Name(w1206) -> ("status"=w1215:bool)
        n558 = property on="Digitizer" class="Bool (strict)"(error in=w1206, "Blinking"=FALSE) -> (error out=w1210:errorcluster)  [unwired: 1 in, 1 out]
        n559 = Not(x=w1215) -> (.not. x?=w1214:bool)
        n560 = Bundle By Name(cluster=w1203, "System Status.Digitizer"=w1214) -> (w1202:T22)
        n561 = call <vilib>:"Add State(s) to Queue__JKI_lib_State_Machine.vi"("State(s) in (\"\")"=w1218) -> ("States Out"=w1217:string)  [unwired: 14 in]
      }
      frame "Digitizer: ConfigCh2Align" {
        # "Synchronize is taking time ~3s."
        # "Config  digitizer\nCall subVi to config digitizer"
        n562 = call "FLImDAQ_FGV.vi"() -> ("Read data"=w1232:T4)  [unwired: 10 in, 1 out]
        n563 = Unbundle By Name(w1225) -> ("FLImDAQ"=w1226:T27)
        n564 = Unbundle By Name(w1232) -> ("Digitizer 1"=w1234:refnum<k15>)
        n565 = Bundle By Name(cluster=w1226, "Channel"=enum16{"Channel 0", "Channel 1", "Channel 0&1"}."Channel 1") -> (w1228:T27)
        n566 = property on="Digitizer" class="Bool (strict)"(error in=w1235, "Blinking"=TRUE) -> (error out=w1230:errorcluster)  [unwired: 1 in, 1 out]
        n567 = case shown="No Error" w1230 {
          selector: w1230 -> [w1243 w1246]
          tunnel: w1228 -> [w1242 _]
          tunnel: [w1245 w1246] -> w1229
          tunnel: w1234 -> [w1244 _]
          frame No Error {
            n568 = call "DigitizerConfigGain.vi"("error in (no error)"=w1243, "FLImDAQ"=w1242, "IVI Refnum in"=w1244) -> ("error out"=w1245:errorcluster)  [unwired: 7 in, 1 out]
          }
          frame Error {
          }
        }
        n569 = Unbundle By Name(w1229) -> ("status"=w1238:bool)
        n570 = property on="Digitizer" class="Bool (strict)"(error in=w1229, "Blinking"=FALSE) -> (error out=w1233:errorcluster)  [unwired: 1 in, 1 out]
        n571 = Not(x=w1238) -> (.not. x?=w1237:bool)
        n572 = Bundle By Name(cluster=w1225, "System Status.Digitizer"=w1237) -> (w1224:T22)
        n573 = call <vilib>:"Add State(s) to Queue__JKI_lib_State_Machine.vi"("State(s) in (\"\")"=w1241) -> ("States Out"=w1240:string)  [unwired: 14 in]
      }
      frame "Digitizer: ConfigCh3Align" {
        # "Synchronize is taking time ~3s."
        # "Config  digitizer\nCall subVi to config digitizer"
        n574 = call "FLImDAQ_FGV.vi"() -> ("Read data"=w1258:T4)  [unwired: 10 in, 1 out]
        n575 = Unbundle By Name(w1248) -> ("FLImDAQ"=w1254:T27)
        n576 = Unbundle By Name(w1258) -> ("Digitizer 1"=w1252:refnum<k15>, "Digitizer 2"=w1247:refnum<k15>)
        n577 = Bundle By Name(cluster=w1254, "Channel"=enum16{"Channel 0", "Channel 1", "Channel 0&1"}."Channel 0") -> (w1251:T27)
        n578 = property on="Digitizer" class="Bool (strict)"(error in=w1260, "Blinking"=TRUE) -> (error out=w1250:errorcluster)  [unwired: 1 in, 1 out]
        n579 = Unbundle By Name(w1248) -> ()  [unwired: 1 out]
        n580 = case shown="No Error" w1250 {
          selector: w1250 -> [w1269 w1271]
          tunnel: w1251 -> [w1268 _]
          tunnel: w1252 -> [w1270 _]
          tunnel: [w1267 w1271] -> w1249
          frame No Error {
            n581 = call "DigitizerConfigGain.vi"("error in (no error)"=w1269, "FLImDAQ"=w1268, "IVI Refnum in"=w1270) -> ("error out"=w1267:errorcluster)  [unwired: 7 in, 1 out]
          }
          frame Error {
          }
        }
        n582 = case shown="No Error" w1249 {
          selector: w1249 -> [w1273 w1278]
          tunnel: w1251 -> [w1276 _]
          tunnel: [w1277 w1278] -> w1256
          tunnel: w1247 -> [w1275 _]
          frame No Error {
            n583 = call <instrlib>:"niScope Reset.vi"("instrument handle"=w1275, "error in"=w1273) -> ("instrument handle out"=w1274:refnum<k15>, "error out"=w1272:errorcluster)  [unwired: 12 in]
            n584 = call "DigitizerConfigGain.vi"("error in (no error)"=w1272, "FLImDAQ"=w1276, "IVI Refnum in"=w1274) -> ("error out"=w1277:errorcluster)  [unwired: 7 in, 1 out]
          }
          frame Error {
          }
        }
        n585 = Unbundle By Name(w1256) -> ("status"=w1263:bool)
        n586 = property on="Digitizer" class="Bool (strict)"(error in=w1256, "Blinking"=FALSE) -> (error out=w1259:errorcluster)  [unwired: 1 in, 1 out]
        n587 = Not(x=w1263) -> (.not. x?=w1262:bool)
        n588 = Bundle By Name(cluster=w1248, "System Status.Digitizer"=w1262) -> (w1253:T22)
        n589 = call <vilib>:"Add State(s) to Queue__JKI_lib_State_Machine.vi"("State(s) in (\"\")"=w1266) -> ("States Out"=w1265:string)  [unwired: 14 in]
      }
      frame "Digitizer: ConfigCh4Align" {
        # "Synchronize is taking time ~3s."
        # "Config  digitizer\nCall subVi to config digitizer"
        n590 = call "FLImDAQ_FGV.vi"() -> ("Read data"=w1290:T4)  [unwired: 10 in, 1 out]
        n591 = Unbundle By Name(w1280) -> ("FLImDAQ"=w1286:T27)
        n592 = Unbundle By Name(w1290) -> ("Digitizer 1"=w1284:refnum<k15>, "Digitizer 2"=w1279:refnum<k15>)
        n593 = Bundle By Name(cluster=w1286, "Channel"=enum16{"Channel 0", "Channel 1", "Channel 0&1"}."Channel 1") -> (w1283:T27)
        n594 = property on="Digitizer" class="Bool (strict)"(error in=w1292, "Blinking"=TRUE) -> (error out=w1282:errorcluster)  [unwired: 1 in, 1 out]
        n595 = Unbundle By Name(w1280) -> ()  [unwired: 1 out]
        n596 = case shown="No Error" w1282 {
          selector: w1282 -> [w1301 w1303]
          tunnel: w1283 -> [w1300 _]
          tunnel: w1284 -> [w1302 _]
          tunnel: [w1299 w1303] -> w1281
          frame No Error {
            n597 = call "DigitizerConfigGain.vi"("error in (no error)"=w1301, "FLImDAQ"=w1300, "IVI Refnum in"=w1302) -> ("error out"=w1299:errorcluster)  [unwired: 7 in, 1 out]
          }
          frame Error {
          }
        }
        n598 = case shown="No Error" w1281 {
          selector: w1281 -> [w1305 w1310]
          tunnel: w1283 -> [w1308 _]
          tunnel: [w1309 w1310] -> w1288
          tunnel: w1279 -> [w1307 _]
          frame No Error {
            n599 = call <instrlib>:"niScope Reset.vi"("instrument handle"=w1307, "error in"=w1305) -> ("instrument handle out"=w1306:refnum<k15>, "error out"=w1304:errorcluster)  [unwired: 12 in]
            n600 = call "DigitizerConfigGain.vi"("error in (no error)"=w1304, "FLImDAQ"=w1308, "IVI Refnum in"=w1306) -> ("error out"=w1309:errorcluster)  [unwired: 7 in, 1 out]
          }
          frame Error {
          }
        }
        n601 = Unbundle By Name(w1288) -> ("status"=w1295:bool)
        n602 = property on="Digitizer" class="Bool (strict)"(error in=w1288, "Blinking"=FALSE) -> (error out=w1291:errorcluster)  [unwired: 1 in, 1 out]
        n603 = Not(x=w1295) -> (.not. x?=w1294:bool)
        n604 = Bundle By Name(cluster=w1280, "System Status.Digitizer"=w1294) -> (w1285:T22)
        n605 = call <vilib>:"Add State(s) to Queue__JKI_lib_State_Machine.vi"("State(s) in (\"\")"=w1298) -> ("States Out"=w1297:string)  [unwired: 14 in]
      }
      frame "Digitizer: Start" {
        # "send trigger to start acquisition loop"
        # "initilize aquisition"
        # "Template Separator\n(You can make a copy of, or modify, this frame)"
        n606 = local read "Channel"() -> (w1311:enum32{"Ch1", "Ch2", "Ch3", "Ch4"})
        n607 = case shown="\"Ch3\"" w1311 {
          tunnel: w1318 -> [_ w1328 w1343]
          tunnel: [w1322 w1330 w1345] -> w1314
          tunnel: w1312 -> [w1325 w1329 w1344]
          frame "Ch1", "Ch2", Default {
            n608 = call "Digitizer1_FGV.vi"("error in (no error)"=w1325, "Operation (Read)"=enum16{"Write", "Read"}."Read" ("Operation")) -> ("error out"=w1324:errorcluster, "Read data"=w1323:refnum<k15>)  [unwired: 8 in]
            n609 = call <instrlib>:"niScope Initiate Acquisition.vi"("instrument handle"=w1323, "error in"=w1324) -> ("error out"=w1322:errorcluster)  [unwired: 12 in, 1 out]
          }
          frame "Ch3" {
            n610 = local read "Task"() -> (w1327:enum32{"iRFAndGain", "Alignment"})
            n611 = case shown="\"Alignment\"" w1327 {
              tunnel: [w1334 w1335] -> w1330
              tunnel: w1329 -> [w1333 w1339]
              tunnel: w1328 -> [w1331 _]
              frame "iRFAndGain", Default {
                n612 = Unbundle By Name(w1331) -> ("niTClk sessions"=w1332:refnum<k20>[])
                n613 = call <instrlib>:"niTClk Initiate.vi"("error in (no error)"=w1333, "sessions"=w1332) -> ("error out"=w1334:errorcluster)  [unwired: 8 in, 1 out]
              }
              frame "Alignment" {
                n614 = call "Digitizer1_FGV.vi"("error in (no error)"=w1339) -> ("error out"=w1340:errorcluster, "Read data"=w1341:refnum<k15>)  [unwired: 9 in]
                n615 = call <instrlib>:"niScope Initiate Acquisition.vi"("instrument handle"=w1341, "error in"=w1340) -> ("error out"=w1338:errorcluster)  [unwired: 12 in, 1 out]
                n616 = call "Digitizer2_FGV.vi"("error in (no error)"=w1338) -> ("error out"=w1337:errorcluster, "Read data"=w1336:refnum<k15>)  [unwired: 9 in]
                n617 = call <instrlib>:"niScope Initiate Acquisition.vi"("instrument handle"=w1336, "error in"=w1337) -> ("error out"=w1335:errorcluster)  [unwired: 12 in, 1 out]
              }
            }
          }
          frame "Ch4" {
            n618 = local read "Task"() -> (w1342:enum32{"iRFAndGain", "Alignment"})
            n619 = case shown="\"iRFAndGain\", Default" w1342 {
              tunnel: [w1349 w1350] -> w1345
              tunnel: w1344 -> [w1348 w1354]
              tunnel: w1343 -> [w1346 _]
              frame "iRFAndGain", Default {
                n620 = Unbundle By Name(w1346) -> ("niTClk sessions"=w1347:refnum<k20>[])
                n621 = call <instrlib>:"niTClk Initiate.vi"("error in (no error)"=w1348, "sessions"=w1347) -> ("error out"=w1349:errorcluster)  [unwired: 8 in, 1 out]
              }
              frame "Alignment" {
                n622 = call "Digitizer1_FGV.vi"("error in (no error)"=w1354) -> ("error out"=w1355:errorcluster, "Read data"=w1356:refnum<k15>)  [unwired: 9 in]
                n623 = call <instrlib>:"niScope Initiate Acquisition.vi"("instrument handle"=w1356, "error in"=w1355) -> ("error out"=w1353:errorcluster)  [unwired: 12 in, 1 out]
                n624 = call "Digitizer2_FGV.vi"("error in (no error)"=w1353) -> ("error out"=w1352:errorcluster, "Read data"=w1351:refnum<k15>)  [unwired: 9 in]
                n625 = call <instrlib>:"niScope Initiate Acquisition.vi"("instrument handle"=w1351, "error in"=w1352) -> ("error out"=w1350:errorcluster)  [unwired: 12 in, 1 out]
              }
            }
          }
        }
        n626 = Generate User Event(priority (normal)=usereventprio."high priority", user event=w1315, event data cluster=TRUE ("event data"), error in=w1314) -> (error out=w1313:errorcluster)  [unwired: 1 out]
        n627 = call <vilib>:"Add State(s) to Queue__JKI_lib_State_Machine.vi"("State(s) in (\"\")"=w1321) -> ("States Out"=w1320:string)  [unwired: 14 in]
      }
      frame "Digitizer: Abort" {
        # "Template Separator\n(You can make a copy of, or modify, this frame)"
        n628 = call "Digitizer1_FGV.vi"("error in (no error)"=w1359, "Operation (Read)"=enum16{"Write", "Read"}."Read" ("Operation")) -> ("error out"=w1366:errorcluster, "Read data"=w1363:refnum<k15>)  [unwired: 8 in]
        n629 = call "Digitizer2_FGV.vi"("error in (no error)"=w1359, "Operation (Read)"=enum16{"Write", "Read"}."Read" ("Operation")) -> ("error out"=w1362:errorcluster, "Read data"=w1364:refnum<k15>)  [unwired: 8 in]
        n630 = call <instrlib>:"niScope Abort.vi"("instrument handle"=w1363, "error in"=w1366) -> ("error out"=w1367:errorcluster)  [unwired: 12 in, 1 out]
        n631 = call <instrlib>:"niScope Abort.vi"("instrument handle"=w1364, "error in"=w1362) -> ("error out"=w1357:errorcluster)  [unwired: 12 in, 1 out]
        n632 = Merge Errors(w1367, w1357) -> (w1360:errorcluster)
        n633 = call <vilib>:"Add State(s) to Queue__JKI_lib_State_Machine.vi"("State(s) in (\"\")"=w1370) -> ("States Out"=w1369:string)  [unwired: 14 in]
      }
      frame "Digitizer: checkTemp" {
        w1378 = enum16{"Write", "Read"}."Read" ("Operation")
        # "Template Separator\n(You can make a copy of, or modify, this frame)"
        n634 = call "Digitizer1_FGV.vi"("error in (no error)"=w1374, "Operation (Read)"=w1378) -> ("error out"=w1380:errorcluster, "Read data"=w1381:refnum<k15>)  [unwired: 8 in]
        n635 = call "Digitizer2_FGV.vi"("error in (no error)"=w1374, "Operation (Read)"=w1378) -> ("error out"=w1376:errorcluster, "Read data"=w1377:refnum<k15>)  [unwired: 8 in]
        n636 = property on="Property Node" class="niScope"(reference=w1381, error in=w1380) -> (error out=w1372:errorcluster, "Device Temperature"=→"Dig1 Temp":dbl)  [unwired: 1 out]
        n637 = property on="Property Node" class="niScope"(reference=w1377, error in=w1376) -> (error out=w1371:errorcluster, "Device Temperature"=→"Dig2 Temp":dbl)  [unwired: 1 out]
        n638 = Merge Errors(w1372, w1371) -> (w1373:errorcluster)
        n639 = call <vilib>:"Add State(s) to Queue__JKI_lib_State_Machine.vi"("State(s) in (\"\")"=w1385) -> ("States Out"=w1384:string)  [unwired: 14 in]
      }
      frame "Digitizer: Close" {
        # "Close Digitizer"
        n640 = call "Digitizer1_FGV.vi"("error in (no error)"=w1393, "Operation (Read)"=enum16{"Write", "Read"}."Read" ("Operation")) -> ("error out"=w1395:errorcluster, "Read data"=w1399:refnum<k15>)  [unwired: 8 in]
        n641 = call "Digitizer2_FGV.vi"("error in (no error)"=w1393, "Operation (Read)"=enum16{"Write", "Read"}."Read" ("Operation")) -> ("error out"=w1394:errorcluster, "Read data"=w1397:refnum<k15>)  [unwired: 8 in]
        n642 = call <instrlib>:"niScope Close.vi"("instrument handle"=w1399, "error in"=w1395) -> ("error out"=w1392:errorcluster)  [unwired: 13 in]
        n643 = call <instrlib>:"niScope Close.vi"("instrument handle"=w1397, "error in"=w1394) -> ("error out"=w1391:errorcluster)  [unwired: 13 in]
        n644 = Merge Errors(w1392, w1391) -> (w1390:errorcluster)
        n645 = Unbundle By Name(w1390) -> ("status"=w1389:bool)
        n646 = Bundle By Name(cluster=w1387, "System Status.Digitizer"=w1389) -> (w1386:T22)
        n647 = call <vilib>:"Add State(s) to Queue__JKI_lib_State_Machine.vi"("State(s) in (\"\")"=w1401) -> ("States Out"=w1400:string)  [unwired: 14 in]
      }
      frame "---------- LabJack ----------" {
        # "Template Separator\n(You can make a copy of, or modify, this frame)"
        n648 = call <vilib>:"Add State(s) to Queue__JKI_lib_State_Machine.vi"("State(s) in (\"\")"=w1406) -> ("States Out"=w1405:string)  [unwired: 14 in]
      }
      frame "LabJack: AB_DC_Start" {
        # "Template Separator\n(You can make a copy of, or modify, this frame)"
        n649 = Unbundle By Name(w1410) -> ("LJ Pinout.AimingBeam PWM"=w1409:string)
        n650 = call "LabJack_FGV.vi"("Operation(Read)"=enum16{"Write", "Read"}."Read", "error in (no error)"=w1413) -> ("error out"=w1411:errorcluster, "Read data"=w1412:i32)  [unwired: 8 in]
        n651 = call "LJM_eWriteName.vi"("Handle In"=w1412, "Name"=w1409, "Value"=1.0, "error in"=w1411) -> ("error out"=w1407:errorcluster)  [unwired: 10 in, 1 out]
        n652 = call <vilib>:"Add State(s) to Queue__JKI_lib_State_Machine.vi"("State(s) in (\"\")"=w1417) -> ("States Out"=w1416:string)  [unwired: 14 in]
      }
      frame "LabJack: AB_DC_Stop" {
        # "Template Separator\n(You can make a copy of, or modify, this frame)"
        n653 = Unbundle By Name(w1421) -> ("LJ Pinout.AimingBeam PWM"=w1420:string)
        n654 = call "LabJack_FGV.vi"("Operation(Read)"=enum16{"Write", "Read"}."Read", "error in (no error)"=w1424) -> ("error out"=w1422:errorcluster, "Read data"=w1423:i32)  [unwired: 8 in]
        n655 = call "LJM_eWriteName.vi"("Handle In"=w1423, "Name"=w1420, "Value"=0.0, "error in"=w1422) -> ("error out"=w1418:errorcluster)  [unwired: 10 in, 1 out]
        n656 = call <vilib>:"Add State(s) to Queue__JKI_lib_State_Machine.vi"("State(s) in (\"\")"=w1428) -> ("States Out"=w1427:string)  [unwired: 14 in]
      }
      frame "LabJack: checkPedal" {
        # "Template Separator\n(You can make a copy of, or modify, this frame)"
        n657 = Unbundle By Name(w1433) -> ("LJ Pinout.Foot Pedal"=w1435:string)
        n658 = local read "Tab Control"() -> (w1432:T2)
        n659 = call "LabJack_FGV.vi"("Operation(Read)"=enum16{"Write", "Read"}."Read" ("Operation"), "error in (no error)"=w1437) -> ("error out"=w1439:errorcluster, "Read data"=w1440:i32)  [unwired: 8 in]
        n660 = Equal?(x=w1432, y=T17."IO Ststus" ("Tab Control")) -> (x = y?=w1430:bool)
        n661 = call "LJM_eReadName.vi"("Handle In"=w1440, "Name"=w1435, "error in"=w1439) -> ("Value"=w1429:dbl, "error out"=w1438:errorcluster)  [unwired: 10 in, 1 out]
        n662 = case shown="True" w1430 {
          tunnel: w1429 -> [_ w1449]
          frame False {
          }
          frame True {
            # "[Covers: REQ14]"
            # "If on IO tab, show foot pedal status"
            n663 = Equal To 0?(x=w1449) -> (x = 0?=w1448:bool)
            n664 = Select(t=FALSE, s=w1448, f=TRUE) -> (s? t:f=w1447:bool)
            n665 = local write "Foot Pedal"(w1447) -> ()
          }
        }
        n666 = case shown="1" w1429 {
          tunnel: [w1450 w1455] -> w1434
          tunnel: ["" ("State(s) in Front (\"\")") w1454] -> w1436
          tunnel: w1433 -> [w1450 w1453]
          frame 0, Default {
          }
          frame 1 {
            # "If Pedal pressed"
            n667 = Unbundle By Name(w1453) -> ("Last Trigger"=w1452:u32)
            n668 = Tick Count (ms)() -> (millisecond timer value=w1459:u32)
            n669 = Subtract(x=w1459, y=w1452) -> (x-y=w1458:u32)
            n670 = Greater Or Equal?(x=w1458, y=u32 2000) -> (x >= y?=w1456:bool)
            n671 = case shown="True" w1456 {
              tunnel: [w1460 w1465] -> w1455
              tunnel: ["" ("State(s) in Front (\"\")") w1464] -> w1454
              tunnel: w1453 -> [w1460 w1462]
              frame False {
              }
              frame True {
                n672 = Tick Count (ms)() -> (millisecond timer value=w1466:u32)
                n673 = Unbundle By Name(w1462) -> ("SysRunning?"=w1463:bool)
                n674 = case shown="True" w1463 {
                  tunnel: ["Macro: StartRun" ("State(s) in Front (\"\")") "Macro: StopRun" ("State(s) in Front (\"\")")] -> w1464
                  frame False {
                  }
                  frame True {
                  }
                }
                n675 = Bundle By Name(cluster=w1462, "Last Trigger"=w1466) -> (w1465:T22)
              }
            }
          }
        }
        n676 = call <vilib>:"Add State(s) to Queue__JKI_lib_State_Machine.vi"("State(s) in Front (\"\")"=w1436, "State(s) in (\"\")"=w1444) -> ("States Out"=w1443:string)  [unwired: 13 in]
      }
      frame "LabJack: ZeroV" {
        # "Just Zero V\nDO not update FGV and front panel\nWIll resume from last V"
        # "set bias to 0"
        # "Zero APD bias\n(You can make a copy of, or modify, this frame)"
        n677 = Unbundle By Name(w1470) -> ("LJ Pinout.Ch1 Bias"=w1476:string, "LJ Pinout.Ch2 Bias"=w1475:string, "LJ Pinout.Ch3 Bias"=w1474:string)
        n678 = Build Array(w1476, w1475, w1474) -> (w1469:string[])
        n679 = call "LabJack_FGV.vi"("Operation(Read)"=enum16{"Write", "Read"}."Read" ("Operation"), "error in (no error)"=w1472) -> ("error out"=w1477:errorcluster, "Read data"=w1478:i32)  [unwired: 8 in]
        n680 = call "LJM_eWriteNames.vi"("Handle In"=w1478, "aNames"=w1469, "aValuesIn"=dbl[] [0.0, 0.0, 0.0], "error in"=w1477) -> ("error out"=w1471:errorcluster)  [unwired: 9 in, 2 out]
        n681 = call <vilib>:"Add State(s) to Queue__JKI_lib_State_Machine.vi"("State(s) in (\"\")"=w1482) -> ("States Out"=w1481:string)  [unwired: 14 in]
      }
      frame "LabJack: SetV" {
        # "set bias to user specifid"
        # "Zero APD bias\n(You can make a copy of, or modify, this frame)"
        n682 = Unbundle By Name(w1486) -> ("LJ Pinout.Ch1 Bias"=w1490:string, "LJ Pinout.Ch2 Bias"=w1488:string, "LJ Pinout.Ch3 Bias"=w1487:string)
        n683 = local read "Channel"() -> (w1491:enum32{"Ch1", "Ch2", "Ch3", "Ch4"})
        n684 = call "V1FGV.vi"("Error In"=w1494, "action (write)"=enum16{"write", "read"}."read" ("action")) -> ("Error Out"=w1483:errorcluster, "V1 out"=w1489:dbl)  [unwired: 8 in]
        n685 = local write "Ctrl V"(w1489) -> ()
        n686 = case shown="\"Ch1\", Default" w1491 {
          tunnel: w1490 -> [w1500 _ _]
          tunnel: [w1500 w1501 w1502] -> w1485
          tunnel: w1488 -> [_ w1501 _]
          tunnel: w1487 -> [_ _ w1502]
          frame "Ch1", Default {
          }
          frame "Ch2" {
          }
          frame "Ch3" {
          }
        }
        n687 = call "LabJack_FGV.vi"("error in (no error)"=w1494) -> ("error out"=w1495:errorcluster, "Read data"=w1496:i32)  [unwired: 9 in]
        n688 = call "LJM_eWriteName.vi"("Handle In"=w1496, "Name"=w1485, "Value"=w1489, "error in"=w1495) -> ("error out"=w1492:errorcluster)  [unwired: 10 in, 1 out]
        n689 = Merge Errors(w1483, w1492) -> (w1493:errorcluster)
        n690 = call <vilib>:"Add State(s) to Queue__JKI_lib_State_Machine.vi"("State(s) in (\"\")"=w1499) -> ("States Out"=w1498:string)  [unwired: 14 in]
      }
      frame "LabJack: Open" {
        # "Initialize LabJack T7\nEstablish connection and initialize pins"
        n691 = call "LJ_Open.vi"("error in"=w1511) -> ("error out"=w1509:errorcluster, "Success?"=w1510:bool, "Handle Out"=w1507:i32)  [unwired: 8 in]
        n692 = call "LabJack_FGV.vi"("Operation(Read)"=enum16{"Write", "Read"}."Write" ("Operation"), "error in (no error)"=w1509, "Write data"=w1507) -> ("error out"=w1506:errorcluster)  [unwired: 7 in, 1 out]
        n693 = Bundle By Name(cluster=w1503, "System Status.Labjack"=w1510) -> (w1504:T22)
        n694 = call <vilib>:"Add State(s) to Queue__JKI_lib_State_Machine.vi"("State(s) in (\"\")"=w1513) -> ("States Out"=w1512:string)  [unwired: 14 in]
      }
      frame "LabJack: SetDefaultSub" {
        w1524 = enum16{"write", "read"}."write" ("action")
        w1537 = "_EF_ENABLE" ("string")
        # "1. Disable PWM\n2. Set all V to 0\n3. Set 355 relay to open\n4. Set LED to off"
        # "read once to set DIO to input"
        # "set all initila V to 0. Set footpedal to input. Set PWM to low. Set laser relay to open. Set LEDs to yellow."
        # "Set Labjack to correct input and output state and initial values"
        n695 = Unbundle By Name(w1523) -> ("LJ Pinout.355 PWM"=w1515:string, "LJ Pinout.AimingBeam PWM"=w1514:string, "LJ Pinout.Ch1 Bias"=w1521:string, "LJ Pinout.Ch2 Bias"=w1520:string, "LJ Pinout.Ch3 Bias"=w1519:string, "LJ Pinout.Laser Start/Stop"=w1518:string, "LJ Pinout.Red LED"=w1517:string, "LJ Pinout.Green LED"=w1516:string)
        n696 = call "V1FGV.vi"("Error In"=w1531, "action (write)"=w1524, "V1 in"=0.0) -> ("Error Out"=w1532:errorcluster, "V1 out"=w1525:dbl)  [unwired: 7 in]
        n697 = call "LabJack_FGV.vi"("Operation(Read)"=enum16{"Write", "Read"}."Read" ("Operation"), "error in (no error)"=w1531) -> ("error out"=w1540:errorcluster, "Read data"=w1541:i32)  [unwired: 8 in]
        n698 = local write "Ctrl V"(w1525) -> ()
        n699 = call "V2FGV.vi"("Error In"=w1532, "action(write)"=w1524, "V2 in"=0.0) -> ("Error Out"=w1529:errorcluster)  [unwired: 7 in, 1 out]
        n700 = Concatenate Strings(w1515, w1537) -> (w1536:string)
        n701 = Concatenate Strings(w1514, w1537) -> (w1535:string)
        n702 = call "V3FGV.vi"("Error In"=w1529, "action(write)"=w1524, "V3 in"=0.0) -> ("Error Out"=w1526:errorcluster)  [unwired: 7 in, 1 out]
        n703 = Build Array(w1515, w1514, w1536, w1535, w1521, w1520, w1519, w1518, w1517, w1516) -> (w1544:string[])
        n704 = Unbundle By Name(w1523) -> ("LJ Pinout.Foot Pedal"=w1522:string)
        n705 = call "LJM_eWriteNames.vi"("Handle In"=w1541, "aNames"=w1544, "aValuesIn"=dbl[] [0.0, 0.0, 0.0, 0.0, 0.0, 0.0, 0.0, 0.0, 0.0, 0.0], "error in"=w1540) -> ("Handle Out"=w1539:i32, "error out"=w1538:errorcluster)  [unwired: 9 in, 1 out]
        n706 = call "LJM_eReadName.vi"("Handle In"=w1539, "Name"=w1522, "error in"=w1538) -> ("error out"=w1528:errorcluster)  [unwired: 10 in, 2 out]
        n707 = Merge Errors(w1528, w1526) -> (w1527:errorcluster)
        n708 = call <vilib>:"Add State(s) to Queue__JKI_lib_State_Machine.vi"("State(s) in (\"\")"=w1547) -> ("States Out"=w1546:string)  [unwired: 14 in]
      }
      frame "LabJack: FootPedalConfig" {
        # "Setup footPedal\n(You can make a copy of, or modify, this frame)"
        n709 = call "LabJack_FGV.vi"("Operation(Read)"=enum16{"Write", "Read"}."Read" ("Operation"), "error in (no error)"=w1549) -> ("error out"=w1553:errorcluster, "Read data"=w1554:i32)  [unwired: 8 in]
        n710 = call "LJM_eWriteName.vi"("Handle In"=w1554, "Name"="DIO15", "Value"=1.0, "error in"=w1553) -> ("error out"=w1550:errorcluster)  [unwired: 10 in, 1 out]
        n711 = call <vilib>:"Add State(s) to Queue__JKI_lib_State_Machine.vi"("State(s) in (\"\")"=w1558) -> ("States Out"=w1557:string)  [unwired: 14 in]
      }
      frame "LabJack: SetDefaultAndClose" {
        # "Template Separator\n(You can make a copy of, or modify, this frame)"
        n712 = call <vilib>:"Add State(s) to Queue__JKI_lib_State_Machine.vi"("State(s) in Front (\"\")"="LabJack: SetDefaultSub\nLabJack: Close" ("State(s) in Front (\"\")"), "State(s) in (\"\")"=w1564) -> ("States Out"=w1563:string)  [unwired: 13 in]
      }
      frame "LabJack: Close" {
        # "Close LabJack Refnum"
        n713 = call "LabJack_FGV.vi"("Operation(Read)"=enum16{"Write", "Read"}."Read" ("Operation"), "error in (no error)"=w1571) -> ("error out"=w1567:errorcluster, "Read data"=w1568:i32)  [unwired: 8 in]
        n714 = Bundle By Name(cluster=w1565, "System Status.Labjack"=FALSE ("System Status.Gain Control")) -> (w1566:T22)
        n715 = call "LJM_Close.vi"("error in"=w1567, "Handle"=w1568) -> ("error out"=w1573:errorcluster)  [unwired: 9 in]
        n716 = call <vilib>:"Add State(s) to Queue__JKI_lib_State_Machine.vi"("State(s) in (\"\")"=w1575) -> ("States Out"=w1574:string)  [unwired: 14 in]
      }
      frame "LabJack: Interlock enable/disable" {
        w1584 = i8 0  # int8
        # "Interlock enable/disable\n(Usage: \"LabJack: Interlock enable/disable >> 1|0\")"
        n717 = Fract/Exp String To Number(string=w1585, default (0 dbl)=w1584) -> (number=w1583:i8)  [unwired: 2 in, 1 out]
        n718 = Unbundle By Name(w1577) -> ("LJ Pinout.Interlock"=w1576:string)
        n719 = call "LabJack_FGV.vi"("Operation(Read)"=enum16{"Write", "Read"}."Read" ("Operation")) -> ("Read data"=w1581:i32)  [unwired: 9 in, 1 out]
        n720 = call "LJM_eWriteName.vi"("Handle In"=w1581, "Name"=w1576, "Value"=w1583, "error in"=w1582) -> ("error out"=w1579:errorcluster)  [unwired: 10 in, 1 out]
        n721 = call <vilib>:"Add State(s) to Queue__JKI_lib_State_Machine.vi"("State(s) in (\"\")"=w1587) -> ("States Out"=w1586:string)  [unwired: 14 in]
      }
      frame "LabJack: 355_PWM_Config" {
        w1597 = 0.0 ("element")
        w1610 = "DIO_EF_CLOCK1_ENABLE"
        # "Config PWM frequency"
        n722 = Unbundle By Name(w1595) -> ("LJ Pinout.355 PWM"=w1589:string)
        n723 = Unbundle By Name(w1595) -> ("355 PWM setting.DIO_EF_CLOCK1_DIVISOR"=w1594:i16, "355 PWM setting.DIO_EF_CLOCK1_ROLL_VALUE"=w1593:i32, "355 PWM setting.DIO#_EF_INDEX"=w1592:i16, "355 PWM setting.DIO#_EF_OPTIONS"=w1591:i16, "355 PWM setting.DIO#_EF_CONFIG_A"=w1590:i32)
        n724 = Concatenate Strings(w1589, "_EF_ENABLE" ("string")) -> (w1606:string)
        n725 = Concatenate Strings(w1589, "_EF_INDEX") -> (w1609:string)
        n726 = Concatenate Strings(w1589, "_EF_OPTIONS") -> (w1608:string)
        n727 = Concatenate Strings(w1589, "_EF_CONFIG_A") -> (w1607:string)
        n728 = call "LabJack_FGV.vi"("Operation(Read)"=enum16{"Write", "Read"}."Read" ("Operation")) -> ("Read data"=w1604:i32)  [unwired: 9 in, 1 out]
        n729 = Build Array(w1597, w1597, w1594, w1593, 1.0 ("element"), 0.0 ("element"), w1592, w1591, w1590) -> (w1601:dbl[])
        n730 = Build Array("DIO_EF_CLOCK0_ENABLE", w1610, "DIO_EF_CLOCK1_DIVISOR", "DIO_EF_CLOCK1_ROLL_VALUE", w1610, w1606, w1609, w1608, w1607) -> (w1605:string[])
        n731 = call "LJM_eWriteNames.vi"("Handle In"=w1604, "aNames"=w1605, "aValuesIn"=w1601, "error in"=w1599) -> ("error out"=w1600:errorcluster)  [unwired: 9 in, 2 out]
        n732 = call <vilib>:"Add State(s) to Queue__JKI_lib_State_Machine.vi"("State(s) in (\"\")"=w1618) -> ("States Out"=w1617:string)  [unwired: 14 in]
      }
      frame "LabJack: AB_PWM_Config" {
        w1630 = 0.0 ("element")
        w1641 = "DIO_EF_CLOCK2_ENABLE"
        # "Set PWM to ground so AB is disabled"
        # "Config PWM frequency"
        n733 = Unbundle By Name(w1628) -> ("LJ Pinout.AimingBeam PWM"=w1619:string)
        n734 = Unbundle By Name(w1628) -> ("AB PWM setting.DIO_EF_CLOCK1_DIVISOR"=w1627:i16, "AB PWM setting.DIO_EF_CLOCK1_ROLL_VALUE"=w1626:i32, "AB PWM setting.DIO#_EF_INDEX"=w1625:i16, "AB PWM setting.DIO#_EF_OPTIONS"=w1624:i16, "AB PWM setting.DIO#_EF_CONFIG_A"=w1623:i32)
        n735 = Concatenate Strings(w1619, "_EF_ENABLE" ("string")) -> (w1637:string)
        n736 = Concatenate Strings(w1619, "_EF_INDEX") -> (w1640:string)
        n737 = Concatenate Strings(w1619, "_EF_OPTIONS") -> (w1639:string)
        n738 = Concatenate Strings(w1619, "_EF_CONFIG_A") -> (w1638:string)
        n739 = Build Array(w1630, w1630, w1627, w1626, 1.0 ("element"), 0.0 ("element"), w1625, w1624, w1623) -> (w1633:dbl[])
        n740 = call "LabJack_FGV.vi"("Operation(Read)"=enum16{"Write", "Read"}."Read" ("Operation"), "error in (no error)"=w1620) -> ("error out"=w1621:errorcluster, "Read data"=w1622:i32)  [unwired: 8 in]
        n741 = Build Array("DIO_EF_CLOCK0_ENABLE", w1641, "DIO_EF_CLOCK2_DIVISOR", "DIO_EF_CLOCK2_ROLL_VALUE", w1641, w1637, w1640, w1639, w1638) -> (w1636:string[])
        n742 = call "LJM_eWriteNames.vi"("Handle In"=w1622, "aNames"=w1636, "aValuesIn"=w1633, "error in"=w1621) -> ("error out"=w1632:errorcluster)  [unwired: 9 in, 2 out]
        n743 = call <vilib>:"Add State(s) to Queue__JKI_lib_State_Machine.vi"("State(s) in (\"\")"=w1650) -> ("States Out"=w1649:string)  [unwired: 14 in]
      }
      frame "LabJack: 355_PWM_Start" {
        # "Template Separator\n(You can make a copy of, or modify, this frame)"
        n744 = Unbundle By Name(w1652) -> ("LJ Pinout.355 PWM"=w1651:string)
        n745 = call "LabJack_FGV.vi"("Operation(Read)"=enum16{"Write", "Read"}."Read" ("Operation"), "error in (no error)"=w1654) -> ("error out"=w1659:errorcluster, "Read data"=w1660:i32)  [unwired: 8 in]
        n746 = Concatenate Strings(w1651, "_EF_ENABLE" ("string")) -> (w1657:string)
        n747 = call "LJM_eWriteName.vi"("Handle In"=w1660, "Name"=w1657, "Value"=1.0, "error in"=w1659) -> ("error out"=w1655:errorcluster)  [unwired: 10 in, 1 out]
        n748 = call <vilib>:"Add State(s) to Queue__JKI_lib_State_Machine.vi"("State(s) in (\"\")"=w1663) -> ("States Out"=w1662:string)  [unwired: 14 in]
      }
      frame "LabJack: AB_PWM_Start" {
        # "Template Separator\n(You can make a copy of, or modify, this frame)"
        n749 = Unbundle By Name(w1665) -> ("LJ Pinout.AimingBeam PWM"=w1664:string)
        n750 = call "LabJack_FGV.vi"("Operation(Read)"=enum16{"Write", "Read"}."Read" ("Operation"), "error in (no error)"=w1667) -> ("error out"=w1672:errorcluster, "Read data"=w1673:i32)  [unwired: 8 in]
        n751 = Concatenate Strings(w1664, "_EF_ENABLE" ("string")) -> (w1670:string)
        n752 = call "LJM_eWriteName.vi"("Handle In"=w1673, "Name"=w1670, "Value"=1.0, "error in"=w1672) -> ("error out"=w1668:errorcluster)  [unwired: 10 in, 1 out]
        n753 = call <vilib>:"Add State(s) to Queue__JKI_lib_State_Machine.vi"("State(s) in (\"\")"=w1676) -> ("States Out"=w1675:string)  [unwired: 14 in]
      }
      frame "LabJack: 355_PWM_Stop" {
        # "Template Separator\n(You can make a copy of, or modify, this frame)"
        n754 = Unbundle By Name(w1679) -> ("LJ Pinout.355 PWM"=w1678:string)
        n755 = call "LabJack_FGV.vi"("Operation(Read)"=enum16{"Write", "Read"}."Read" ("Operation"), "error in (no error)"=w1684) -> ("error out"=w1687:errorcluster, "Read data"=w1682:i32)  [unwired: 8 in]
        n756 = Concatenate Strings(w1678, "_EF_ENABLE" ("string")) -> (w1685:string)
        n757 = call "LJM_eWriteName.vi"("Handle In"=w1682, "Name"=w1685, "Value"=0.0, "error in"=w1687) -> ("error out"=w1680:errorcluster)  [unwired: 10 in, 1 out]
        n758 = local write "355nm Laser toggle"(FALSE ("355nm Laser toggle")) -> ()
        n759 = call <vilib>:"Add State(s) to Queue__JKI_lib_State_Machine.vi"("State(s) in (\"\")"=w1690) -> ("States Out"=w1689:string)  [unwired: 14 in]
      }
      frame "LabJack: AB_PWM_Stop" {
        # "Template Separator\n(You can make a copy of, or modify, this frame)"
        n760 = Unbundle By Name(w1692) -> ("LJ Pinout.AimingBeam PWM"=w1691:string)
        n761 = call "LabJack_FGV.vi"("Operation(Read)"=enum16{"Write", "Read"}."Read" ("Operation"), "error in (no error)"=w1695) -> ("error out"=w1700:errorcluster, "Read data"=w1701:i32)  [unwired: 8 in]
        n762 = Concatenate Strings(w1691, "_EF_ENABLE" ("string")) -> (w1698:string)
        n763 = call "LJM_eWriteName.vi"("Handle In"=w1701, "Name"=w1698, "Value"=0.0, "error in"=w1700) -> ("error out"=w1696:errorcluster)  [unwired: 10 in, 1 out]
        n764 = local write "Aiming beam toggle"(FALSE ("Aiming beam toggle")) -> ()
        n765 = call <vilib>:"Add State(s) to Queue__JKI_lib_State_Machine.vi"("State(s) in (\"\")"=w1704) -> ("States Out"=w1703:string)  [unwired: 14 in]
      }
      frame "---------- LED ----------" {
        # "Template Separator\n(You can make a copy of, or modify, this frame)"
        n766 = call <vilib>:"Add State(s) to Queue__JKI_lib_State_Machine.vi"("State(s) in (\"\")"=w1709) -> ("States Out"=w1708:string)  [unwired: 14 in]
      }
      frame "LED: BreathGreen" {
        w1712 = FALSE ("Wait Until Done")
        # "breath LED Green\n(Run VI in background using VI server to breath LED green )"
        n767 = Unbundle By Name(w1718) -> ("LED vi reference"=w1717:refnum<vi>)
        n768 = invoke class="VI" method="Ctrl Val.Set"(reference=w1717, error in=w1710, "Control Name"="Color", "Value"=0) -> (reference out=w1714:refnum<vi>, error out=w1713:errorcluster)  [unwired: 1 in, 3 out]
        n769 = invoke class="VI" method="Run VI"(reference=w1714, error in=w1713, "Wait until done"=w1712, "Auto Dispose Ref"=w1712) -> (error out=w1711:errorcluster)  [unwired: 1 in, 4 out]
        n770 = call <vilib>:"Add State(s) to Queue__JKI_lib_State_Machine.vi"("State(s) in (\"\")"=w1721) -> ("States Out"=w1720:string)  [unwired: 14 in]
      }
      frame "LED: BreathOrange" {
        w1724 = FALSE ("Wait Until Done")
        # "breath LED Green\n(Run VI in background using VI server to breath LED green )"
        n771 = Unbundle By Name(w1730) -> ("LED vi reference"=w1729:refnum<vi>)
        n772 = invoke class="VI" method="Ctrl Val.Set"(reference=w1729, error in=w1722, "Control Name"="Color", "Value"=1) -> (reference out=w1726:refnum<vi>, error out=w1725:errorcluster)  [unwired: 1 in, 3 out]
        n773 = invoke class="VI" method="Run VI"(reference=w1726, error in=w1725, "Wait until done"=w1724, "Auto Dispose Ref"=w1724) -> (error out=w1723:errorcluster)  [unwired: 1 in, 4 out]
        n774 = call <vilib>:"Add State(s) to Queue__JKI_lib_State_Machine.vi"("State(s) in (\"\")"=w1733) -> ("States Out"=w1732:string)  [unwired: 14 in]
      }
      frame "LED: OpenVIRef" {
        # "Open LED vi ref\n(You can make a copy of, or modify, this frame)"
        n775 = call <vilib>:"Application Directory.vi"() -> ("Application Directory"=w1738:path)
        n776 = Build Path(base path=w1738, name or relative path="SubVI") -> (appended path=w1736:path)
        n777 = Build Path(base path=w1736, name or relative path="LEDBreath.vi") -> (appended path=w1734:path)
        n778 = Open VI Reference(vi path=w1734, error in (no error)=w1743) -> (vi reference=w1740:refnum<vi>, error out=w1742:errorcluster)  [unwired: 4 in]
        n779 = case shown="No Error" w1742 {
          tunnel: w1741 -> [w1747 w1751]
          tunnel: w1740 -> [w1750 _]
          tunnel: [w1748 w1751] -> w1739
          frame No Error {
            n780 = Bundle By Name(cluster=w1747, "LED vi reference"=w1750, "LedViRefOpen"=TRUE) -> (w1748:T22)
          }
          frame Error {
          }
        }
        n781 = call <vilib>:"Add State(s) to Queue__JKI_lib_State_Machine.vi"("State(s) in (\"\")"=w1746) -> ("States Out"=w1745:string)  [unwired: 14 in]
      }
      frame "LED: CloseVIRef" {
        # "Template Separator\n(You can make a copy of, or modify, this frame)"
        n782 = Unbundle By Name(w1753) -> ("LedViRefOpen"=w1752:bool, "LED vi reference"=w1755:refnum<vi>)
        n783 = case shown="True" w1752 {
          tunnel: w1756 -> [w1760 w1763]
          tunnel: w1755 -> [_ w1761]
          tunnel: [w1760 w1762] -> w1754
          frame False {
          }
          frame True {
            n784 = Close Reference(reference=w1761, error in (no error)=w1763) -> (error out=w1762:errorcluster)
          }
        }
        n785 = call <vilib>:"Add State(s) to Queue__JKI_lib_State_Machine.vi"("State(s) in (\"\")"=w1759) -> ("States Out"=w1758:string)  [unwired: 14 in]
      }
      frame "LED: BreathOff" {
        # "System LED Breath Off\n(LED breath off"
        n786 = Unbundle By Name(w1770) -> ("LED vi reference"=w1772:refnum<vi>)
        n787 = invoke on="Invoke Node" class="VI" method="Ctrl Val.Set"(reference=w1772, error in=w1771, "Control Name"="Stop", "Value"=TRUE) -> (reference out=w1766:refnum<vi>, error out=w1767:errorcluster)  [unwired: 1 in, 3 out]
        n788 = case shown="No Error" w1767 {
          selector: w1767 -> [w1777 _]
          tunnel: [w1776 errorcluster {"status"=FALSE, "code"=0, "source"=""} ("error IO")] -> w1764
          tunnel: ["" ("State(s) in Front (\"\")") "LED: BreathOff" ("State(s) in Front (\"\")")] -> w1765
          tunnel: w1766 -> [w1778 _]
          frame No Error {
            # "No error, wait for VI to stop"
            n789 = while {
              tunnel: w1778 -> [w1786]
              shift-right: [w1780] -> w1776
              shift-left: w1777 -> [w1785]
              stop <- w1782 stop-if-true
              # "continue check whether vi is running"
              n790 = property class="VI"(reference=w1786, error in=w1785) -> (error out=w1780:errorcluster, "Exec.State"=w1784:T18)  [unwired: 1 out]
              n791 = Wait (ms)(milliseconds to wait=u32 50) -> ()  [unwired: 1 out]
              n792 = Equal?(x=w1784, y=T18."Idle") -> (x = y?=w1782:bool)
            }
          }
          frame Error {
            # "try again when error"
          }
        }
        n793 = call <vilib>:"Add State(s) to Queue__JKI_lib_State_Machine.vi"("State(s) in Front (\"\")"=w1765, "State(s) in (\"\")"=w1775) -> ("States Out"=w1774:string)  [unwired: 13 in]
      }
      frame "LED: Off" {
        # "set LED to red"
        # "Template Separator\n(You can make a copy of, or modify, this frame)"
        n794 = Unbundle By Name(w1791) -> ("LJ Pinout.Red LED"=w1790:string, "LJ Pinout.Green LED"=w1789:string)
        n795 = call "LabJack_FGV.vi"("Operation(Read)"=enum16{"Write", "Read"}."Read" ("Operation"), "error in (no error)"=w1792) -> ("error out"=w1799:errorcluster, "Read data"=w1798:i32)  [unwired: 8 in]
        n796 = call "LJM_eWriteName.vi"("Handle In"=w1798, "Name"=w1790, "Value"=0.0, "error in"=w1799) -> ("Handle Out"=w1796:i32, "error out"=w1795:errorcluster)  [unwired: 10 in]
        n797 = call "LJM_eWriteName.vi"("Handle In"=w1796, "Name"=w1789, "Value"=0.0, "error in"=w1795) -> ("error out"=w1793:errorcluster)  [unwired: 10 in, 1 out]
        n798 = call <vilib>:"Add State(s) to Queue__JKI_lib_State_Machine.vi"("State(s) in (\"\")"=w1803) -> ("States Out"=w1802:string)  [unwired: 14 in]
      }
      frame "LED: Green" {
        # "set LED to green"
        # "Template Separator\n(You can make a copy of, or modify, this frame)"
        n799 = Unbundle By Name(w1806) -> ("LJ Pinout.Red LED"=w1805:string, "LJ Pinout.Green LED"=w1804:string)
        n800 = call "LabJack_FGV.vi"("Operation(Read)"=enum16{"Write", "Read"}."Read" ("Operation"), "error in (no error)"=w1809) -> ("error out"=w1815:errorcluster, "Read data"=w1814:i32)  [unwired: 8 in]
        n801 = call "LJM_eWriteName.vi"("Handle In"=w1814, "Name"=w1805, "Value"=0.0, "error in"=w1815) -> ("Handle Out"=w1812:i32, "error out"=w1811:errorcluster)  [unwired: 10 in]
        n802 = call "LJM_eWriteName.vi"("Handle In"=w1812, "Name"=w1804, "Value"=9.0, "error in"=w1811) -> ("error out"=w1808:errorcluster)  [unwired: 10 in, 1 out]
        n803 = call <vilib>:"Add State(s) to Queue__JKI_lib_State_Machine.vi"("State(s) in (\"\")"=w1818) -> ("States Out"=w1817:string)  [unwired: 14 in]
      }
      frame "---------- Queue ----------" {
        # "Template Separator\n(You can make a copy of, or modify, this frame)"
        n804 = call <vilib>:"Add State(s) to Queue__JKI_lib_State_Machine.vi"("State(s) in (\"\")"=w1823) -> ("States Out"=w1822:string)  [unwired: 14 in]
      }
      frame "Queue: CheckCtrlVQ" {
        # "Check control V queue\n(if contorl V queue is not empty, aquire data)"
        n805 = Unbundle By Name(w1828) -> ("SysRunning?"=w1827:bool)
        n806 = case shown="False" w1827 {
          tunnel: w1824 -> [w1840 w1857]
          tunnel: w1829 -> [w1839 _]
          tunnel: [w1835 "" ("State with Arguments")] -> w1826
          tunnel: [w1833 w1857] -> w1825
          frame False {
            # "system idle"
            n807 = Get Queue Status(queue=w1839, error in (no error)=w1840) -> (queue out=w1837:refnum<queue>, error out=w1836:errorcluster, # elements in queue=w1834:i32)  [unwired: 1 in, 5 out]
            n808 = Greater Than 0?(x=w1834) -> (x > 0?=w1838:bool)
            n809 = case shown="True" w1838 {
              tunnel: w1837 -> [_ w1854]
              tunnel: w1836 -> [w1841 w1853]
              tunnel: ["" ("State with Arguments") w1845] -> w1835
              tunnel: w1834 -> [_ w1849]
              tunnel: [w1841 w1843] -> w1833
              frame False {
              }
              frame True {
                n810 = Dequeue Element(queue=w1854, error in (no error)=w1853) -> (element=w1850:dbl, error out=w1843:errorcluster)  [unwired: 1 in, 2 out]
                n811 = Equal?(x=w1849, y=1) -> (x = y?=w1847:bool)
                n812 = Number To Fractional String(number=w1850) -> (F-format string=w1851:string)  [unwired: 3 in]
                n813 = case shown="True" w1847 {
                  tunnel: ["" ("Empty String Constant") "Data: parseDataAllGainMacro\nMacro: AskOverWrite"] -> w1844
                  frame False {
                  }
                  frame True {
                    # "if last control V, parse all data and ask whether to over-write"
                  }
                }
                n814 = call <vilib>:"Build State String with Arguments__JKI_lib_State_Machine.vi"("Arguments (\"\")"=w1851, "State"="Aquisition: RecordData") -> ("State with Arguments"=w1846:string)  [unwired: 4 in]
                n815 = call <vilib>:"Add State(s) to Queue__JKI_lib_State_Machine.vi"("State(s) in Front (\"\")"=w1846, "State(s) in (\"\")"=w1844) -> ("States Out"=w1845:string)  [unwired: 13 in]
              }
            }
          }
          frame True {
            # "System running"
          }
        }
        n816 = call <vilib>:"Add State(s) to Queue__JKI_lib_State_Machine.vi"("State(s) in Front (\"\")"=w1826, "State(s) in (\"\")"=w1832) -> ("States Out"=w1831:string)  [unwired: 13 in]
      }
      frame "Queue: FlashDataAllQueue" {
        # "Flash control V queue and DataAll queue\n(You can make a copy of, or modify, this frame)"
        n817 = Flush Queue(queue=w1864, error in (no error)=w1861) -> (error out=w1862:errorcluster)  [unwired: 2 out]
        n818 = Flush Queue(queue=w1866, error in (no error)=w1861) -> (error out=w1865:errorcluster)  [unwired: 2 out]
        n819 = Flush Queue(queue=w1860, error in (no error)=w1861) -> (error out=w1859:errorcluster)  [unwired: 2 out]
        n820 = Merge Errors(w1862, w1865, w1859) -> (w1863:errorcluster)
        n821 = call <vilib>:"Add State(s) to Queue__JKI_lib_State_Machine.vi"("State(s) in (\"\")"=w1870) -> ("States Out"=w1869:string)  [unwired: 14 in]
      }
      frame "Queue: CheckNumOfWF" {
        # "Template Separator\n(You can make a copy of, or modify, this frame)"
        n822 = call "FLImDAQ_FGV.vi"() -> ("Read data"=w1873:T4)  [unwired: 10 in, 1 out]
        n823 = Unbundle By Name(w1873) -> ("Waveform to Avg"=w1872:i16)
        n824 = Get Queue Status(queue=w1875) -> (# elements in queue=w1874:i32)  [unwired: 2 in, 7 out]
        n825 = Multiply(x=w1874, y=w1872) -> (x*y=w1871:i32)
        "numWFInQ" <- w1871
        n826 = Greater Or Equal?(x=w1871, y="Num WF to acquire") -> (x >= y?=w1877:bool)
        n827 = case shown="False" w1877 {
          tunnel: ["Queue: CheckNumOfWF" ("State(s) in Front (\"\")") "" ("State(s) in Front (\"\")")] -> w1876
          frame False {
            n828 = Wait (ms)(milliseconds to wait=u32 5) -> ()  [unwired: 1 out]
          }
          frame True {
          }
        }
        n829 = call <vilib>:"Add State(s) to Queue__JKI_lib_State_Machine.vi"("State(s) in Front (\"\")"=w1876, "State(s) in (\"\")"=w1883) -> ("States Out"=w1882:string)  [unwired: 13 in]
      }
      frame "Queue: Create" {
        # "Template Separator\n(You can make a copy of, or modify, this frame)"
        n830 = call <vilib>:"Add State(s) to Queue__JKI_lib_State_Machine.vi"("State(s) in (\"\")"=w1891) -> ("States Out"=w1890:string)  [unwired: 14 in]
      }
      frame "Queue: Flash" {
        # "Clear queue contnet\n(clear queue content by flash it)"
        n831 = Flush Queue(queue=w1895, error in (no error)=w1892) -> (error out=w1894:errorcluster)  [unwired: 2 out]
        n832 = local write "numWFInQ"(0 ("numWFInQ")) -> ()
        n833 = call <vilib>:"Add State(s) to Queue__JKI_lib_State_Machine.vi"("State(s) in (\"\")"=w1899) -> ("States Out"=w1898:string)  [unwired: 14 in]
      }
      frame "Queue: Destory" {
        # "Destory Data Queue\nDistory data queue ref so the aquisition loop stop"
        n834 = Release Queue(queue=w1907, error in (no error)=w1902) -> (error out=w1910:errorcluster)  [unwired: 1 in, 2 out]
        n835 = Release Queue(queue=w1906, error in (no error)=w1902) -> (error out=w1909:errorcluster)  [unwired: 1 in, 2 out]
        n836 = Release Queue(queue=w1904, error in (no error)=w1902) -> (error out=w1903:errorcluster)  [unwired: 1 in, 2 out]
        n837 = Release Queue(queue=w1901, error in (no error)=w1902) -> (error out=w1900:errorcluster)  [unwired: 1 in, 2 out]
        n838 = Merge Errors(w1910, w1909, w1903, w1900) -> (w1908:errorcluster)
        n839 = call <vilib>:"Add State(s) to Queue__JKI_lib_State_Machine.vi"("State(s) in (\"\")"=w1913) -> ("States Out"=w1912:string)  [unwired: 14 in]
      }
      frame "---------- SysConfig ----------" {
        # "Template Separator\n(You can make a copy of, or modify, this frame)"
        n840 = call <vilib>:"Add State(s) to Queue__JKI_lib_State_Machine.vi"("State(s) in (\"\")"=w1918) -> ("States Out"=w1917:string)  [unwired: 14 in]
      }
      frame "SysConfig: Load APD Info" {
        # "Macro to load APD data\n(load from serial number -> load all data -> get gain limit)"
        n841 = call <vilib>:"Add State(s) to Queue__JKI_lib_State_Machine.vi"("State(s) in Front (\"\")"="APD: LoadFromSerialNoRawData\nAPD: UpdateIndicatorMacro\nAPD: GetGainLimits" ("State(s) in Front (\"\")"), "State(s) in (\"\")"=w1924) -> ("States Out"=w1923:string)  [unwired: 13 in]
      }
      frame "SysConfig: Load Digitizer Setting" {
        w1927 = enum16{"Write", "Read"}."Write" ("Operation")
        # "Digitizers in FLImDAQ is not used\nLoad DAQ config\nSave to FGV"
        # "Template Separator\n(You can make a copy of, or modify, this frame)"
        n842 = call <userlib>:"Current VIs Parent Directory__ogtk.vi"() -> ("Parent Directory (+ Relative)"=w1938:path)  [unwired: 5 in]
        n843 = Build Path(base path=w1938, name or relative path="SubVI\\DigitizerConfiguration\\V6_Scope_iRFNew.config") -> (appended path=w1939:path)
        n844 = call "ReadDigitizerConfig(SubVI).vi"("error in (no error)"=w1936, "appended path"=w1939) -> ("error out"=w1931:errorcluster, "FLImDAQ"=w1929:T4)  [unwired: 8 in]
        n845 = call "FLImDAQ_FGV.vi"("error in (no error)"=w1931, "Operation (Read)"=w1927, "Write data"=w1929) -> ("error out"=w1934:errorcluster)  [unwired: 7 in, 1 out]
        n846 = Bundle By Name(cluster=w1925, "FLImDAQ"=w1929) -> (w1926:T22)
        n847 = Unbundle By Name(w1929) -> ("Digitizer 1"=w1932:refnum<k15>, "Digitizer 2"=w1933:refnum<k15>)
        n848 = call "Digitizer1_FGV.vi"("error in (no error)"=w1934, "Operation (Read)"=w1927, "Write data"=w1932) -> ("error out"=w1935:errorcluster)  [unwired: 7 in, 1 out]
        n849 = call "Digitizer2_FGV.vi"("error in (no error)"=w1935, "Operation (Read)"=w1927, "Write data"=w1933) -> ("error out"=w1930:errorcluster)  [unwired: 7 in, 1 out]
        n850 = call <vilib>:"Add State(s) to Queue__JKI_lib_State_Machine.vi"("State(s) in (\"\")"=w1941) -> ("States Out"=w1940:string)  [unwired: 14 in]
      }
      frame "SysConfig: Load Digitizer Setting Gain" {
        w1944 = enum16{"Write", "Read"}."Write" ("Operation")
        # "Digitizers in FLImDAQ is not used\nLoad DAQ config\nSave to FGV"
        # "Template Separator\n(You can make a copy of, or modify, this frame)"
        n851 = call <userlib>:"Current VIs Parent Directory__ogtk.vi"() -> ("Parent Directory (+ Relative)"=w1955:path)  [unwired: 5 in]
        n852 = Build Path(base path=w1955, name or relative path="SubVI\\DigitizerConfiguration\\V6_Scope_Gain.config") -> (appended path=w1956:path)
        n853 = call "ReadDigitizerConfig(SubVI).vi"("error in (no error)"=w1953, "appended path"=w1956) -> ("error out"=w1948:errorcluster, "FLImDAQ"=w1946:T4)  [unwired: 8 in]
        n854 = call "FLImDAQ_FGV.vi"("error in (no error)"=w1948, "Operation (Read)"=w1944, "Write data"=w1946) -> ("error out"=w1951:errorcluster)  [unwired: 7 in, 1 out]
        n855 = Bundle By Name(cluster=w1942, "FLImDAQ"=w1946) -> (w1943:T22)
        n856 = Unbundle By Name(w1946) -> ("Digitizer 1"=w1949:refnum<k15>, "Digitizer 2"=w1950:refnum<k15>)
        n857 = call "Digitizer1_FGV.vi"("error in (no error)"=w1951, "Operation (Read)"=w1944, "Write data"=w1949) -> ("error out"=w1952:errorcluster)  [unwired: 7 in, 1 out]
        n858 = call "Digitizer2_FGV.vi"("error in (no error)"=w1952, "Operation (Read)"=w1944, "Write data"=w1950) -> ("error out"=w1947:errorcluster)  [unwired: 7 in, 1 out]
        n859 = call <vilib>:"Add State(s) to Queue__JKI_lib_State_Machine.vi"("State(s) in (\"\")"=w1958) -> ("States Out"=w1957:string)  [unwired: 14 in]
      }
      frame "SysConfig: Load LJ Pinout" {
        # "Template Separator\n(You can make a copy of, or modify, this frame)"
        n860 = call <userlib>:"Current VIs Parent Directory__ogtk.vi"() -> ("Parent Directory (+ Relative)"=w1973:path)  [unwired: 5 in]
        n861 = Build Path(base path=w1973, name or relative path="SubVI\\LabJack\\LJ_pin_setting.config") -> (appended path=w1971:path)
        n862 = call "ReadLabjackConfig(SubVI).vi"("error in (no error)"=w1969, "appended path"=w1971) -> ("error out"=w1970:errorcluster, "Utility"=w1968:T3)  [unwired: 8 in]
        n863 = Unbundle By Name(w1968) -> ("Ch1 Bias"=w1967:string, "Ch2 Bias"=w1966:string, "Ch3 Bias"=w1965:string, "Ch4 Bias"=w1959:string, "Red LED"=w1963:string, "Green LED"=w1962:string)
        n864 = global write "GlobalVariables.vi" "LED Green pin"(w1962) -> ()
        n865 = global write "GlobalVariables.vi" "LED Red pin"(w1963) -> ()
        n866 = global write "GlobalVariables.vi" "Ch1 LJ pin"(w1967) -> ()
        n867 = global write "GlobalVariables.vi" "Ch2 LJ pin"(w1966) -> ()
        n868 = global write "GlobalVariables.vi" "Ch3 LJ pin"(w1965) -> ()
        n869 = global write "GlobalVariables.vi" "Ch4 LJ pin"(w1959) -> ()
        n870 = Bundle By Name(cluster=w1960, "LJ Pinout"=w1968) -> (w1961:T22)
        n871 = call <vilib>:"Add State(s) to Queue__JKI_lib_State_Machine.vi"("State(s) in (\"\")"=w1975) -> ("States Out"=w1974:string)  [unwired: 14 in]
      }
      frame "SysConfig: Load 355 PWM" {
        # "Template Separator\n(You can make a copy of, or modify, this frame)"
        n872 = call <userlib>:"Current VIs Parent Directory__ogtk.vi"() -> ("Parent Directory (+ Relative)"=w1993:path)  [unwired: 5 in]
        n873 = Build Path(base path=w1993, name or relative path="SubVI\\LabJack\\PWM_setting_355.config") -> (appended path=w1991:path)
        n874 = call "ReadPWMConfig(SubVI).vi"("error in (no error)"=w1989, "appended path"=w1991) -> ("error out"=w1990:errorcluster, "PWM Setting"=w1988:T32)  [unwired: 8 in]
        n875 = Unbundle By Name(w1988) -> ("DIO_EF_CLOCK1_DIVISOR"=w1985:i16, "DIO_EF_CLOCK1_ROLL_VALUE"=w1984:i32)
        n876 = Multiply(x=w1985, y=w1984) -> (x*y=w1986:i32)
        n877 = Bundle By Name(cluster=w1976, "355 PWM setting"=w1988) -> (w1977:T22)
        n878 = Divide(x=80000000.0, y=w1986) -> (x/y=w1978:dbl)
        n879 = Number To Decimal String(number=w1978) -> (decimal integer string=w1983:string)  [unwired: 1 in]
        n880 = Concatenate Strings("355nm " ("string"), w1983, "Hz" ("string")) -> (w1981:string)
        n881 = local write "Laser Rep Rate"(w1978) -> ()
        n882 = property on="355nm Laser toggle" class="Bool (strict)"("Caption.Text"=w1981) -> ()  [unwired: 2 in, 2 out]
        n883 = call <vilib>:"Add State(s) to Queue__JKI_lib_State_Machine.vi"("State(s) in (\"\")"=w1995) -> ("States Out"=w1994:string)  [unwired: 14 in]
      }
      frame "SysConfig: Load AB PWM" {
        # "Load AB PWM setting\n(load setting, update AB toggle text)"
        n884 = call <userlib>:"Current VIs Parent Directory__ogtk.vi"() -> ("Parent Directory (+ Relative)"=w2018:path)  [unwired: 5 in]
        n885 = Build Path(base path=w2018, name or relative path="SubVI\\LabJack\\PWM_setting_AB.config") -> (appended path=w2016:path)
        n886 = call "ReadPWMConfig(SubVI).vi"("error in (no error)"=w2014, "appended path"=w2016) -> ("error out"=w2015:errorcluster, "PWM Setting"=w2013:T32)  [unwired: 8 in]
        n887 = Unbundle By Name(w2013) -> ("DIO_EF_CLOCK1_DIVISOR"=w2010:i16, "DIO_EF_CLOCK1_ROLL_VALUE"=w1999:i32, "DIO#_EF_CONFIG_A"=w2000:i32)
        n888 = Divide(x=w2000, y=w1999) -> (x/y=w1998:dbl)
        n889 = Multiply(x=w2010, y=w1999) -> (x*y=w2011:i32)
        n890 = Multiply(x=w1998, y=100.0) -> (x*y=w1996:dbl)
        n891 = Bundle By Name(cluster=w2001, "AB PWM setting"=w2013) -> (w2002:T22)
        n892 = Divide(x=80000000.0, y=w2011) -> (x/y=w2003:dbl)
        n893 = Number To Decimal String(number=w2003, width (-)=i16 2) -> (decimal integer string=w2009:string)
        n894 = local write "Duty Cycle (%)"(w1996) -> ()
        n895 = local write "AB Rep Rate"(w2003) -> ()
        n896 = Concatenate Strings("445nm " ("string"), w2009, "Hz " ("string")) -> (w2007:string)
        n897 = property on="Aiming beam toggle" class="Bool (strict)"("Caption.Text"=w2007) -> ()  [unwired: 2 in, 2 out]
        n898 = call <vilib>:"Add State(s) to Queue__JKI_lib_State_Machine.vi"("State(s) in (\"\")"=w2020) -> ("States Out"=w2019:string)  [unwired: 14 in]
      }
      frame "SysConfig: Load AB setting" {
        # "Template Separator\n(You can make a copy of, or modify, this frame)"
        n899 = call "readAimingBeamSetting.vi"("error in (no error)"=w2024) -> ("error out"=w2023:errorcluster, "Aiming Beam Setting"=w2022:T33)  [unwired: 9 in]
        n900 = Bundle By Name(cluster=w2025, "AB Cluster"=w2022) -> (w2026:T22)
        n901 = Unbundle By Name(w2022) -> ("Frequency(Hz)"=w2021:u32)
        n902 = local write "AB Rep Rate"(w2021) -> ()
        n903 = call <vilib>:"Add State(s) to Queue__JKI_lib_State_Machine.vi"("State(s) in (\"\")"=w2029) -> ("States Out"=w2028:string)  [unwired: 14 in]
      }
      frame "---------- SystemStatus ----------" {
        # "Template Separator\n(You can make a copy of, or modify, this frame)"
        n904 = call <vilib>:"Add State(s) to Queue__JKI_lib_State_Machine.vi"("State(s) in (\"\")"=w2034) -> ("States Out"=w2033:string)  [unwired: 14 in]
      }
      frame "SystemStatus: SlowSysStatusMacro" {
        # "store system check time"
        # "Template Separator\n(You can make a copy of, or modify, this frame)"
        n905 = Tick Count (ms)() -> (millisecond timer value=w2037:u32)
        n906 = Bundle By Name(cluster=w2035, "SlowTimer"=w2037) -> (w2036:T22)
        n907 = call <vilib>:"Add State(s) to Queue__JKI_lib_State_Machine.vi"("State(s) in Front (\"\")"="/*Digitizer: checkTemp" ("State(s) in Front (\"\")"), "State(s) in (\"\")"=w2042) -> ("States Out"=w2041:string)  [unwired: 13 in]
      }
      frame "SystemStatus: FastSysStatusMacro" {
        # "store system check time"
        # "Template Separator\n(You can make a copy of, or modify, this frame)"
        n908 = Tick Count (ms)() -> (millisecond timer value=w2045:u32)
        n909 = Bundle By Name(cluster=w2043, "FastTimer"=w2045) -> (w2044:T22)
        n910 = call <vilib>:"Add State(s) to Queue__JKI_lib_State_Machine.vi"("State(s) in Front (\"\")"="355 Laser: CheckPWMStatus\nAimingBeam: GetPWMStatus" ("State(s) in Front (\"\")"), "State(s) in (\"\")"=w2050) -> ("States Out"=w2049:string)  [unwired: 13 in]
      }
      frame "---------- UI ----------" {
        # "Do not put any code in this frame.\n(It is a separator no-op. You can make a copy of this frame to create a new UI frame)"
        n911 = call <vilib>:"Add State(s) to Queue__JKI_lib_State_Machine.vi"("State(s) in (\"\")"=w2055) -> ("States Out"=w2054:string)  [unwired: 14 in]
      }
      frame "UI: InitIRFDataTable" {
        # "Initial iRF table setup\n(Setup the table for iRF measurement, set the active cell to 1st roll)"
        n912 = while {
          tunnel: [w2080] -> w2059 mode=indexing
          shift-right: [w2080] -> _
          shift-left: 0.03 -> [w2086]
          stop <- w2081 continue-if-true
          # "Generate Gain less than 3"
          n913 = Greater Or Equal?(x=w2086, y=3.0) -> (x >= y?=w2089:bool)
          n914 = Select(t=0.1, s=w2089, f=0.3) -> (s? t:f=w2085:dbl)
          n915 = Add(x=w2085, y=w2086) -> (x+y=w2084:dbl)
          n916 = In Range and Coerce(upper limit=4.6, x=w2084, lower limit=0.05) -> (coerced(x)=w2080:dbl, In Range?=w2081:bool)
        }
        "iRFCtrlV" <- w2059
        n917 = for {
          tunnel: w2059 -> [w2079] mode=indexing
          tunnel: [w2075] -> w2058 mode=indexing
          tunnel: T19 {"Row"=0, "Column"=0} ("Active Cell:Active Cell") -> [w2070]
          i -> [w2069]
          n918 = Bundle By Name(cluster=w2070, "Row"=w2069, "Column"=0) -> (w2073:T19)
          n919 = Number To Fractional String(number=w2079, precision (6)=i16 2) -> (F-format string=w2077:string)  [unwired: 2 in]
          n920 = Equal To 0?(x=w2069) -> (x = 0?=w2068:bool)
          n921 = Select(t=u32 16773632 ("Active Cell:Cell Background Color"), s=w2068, f=u32 16448250 ("Active Cell:Cell Background Color")) -> (s? t:f=w2065:u32)
          n922 = property on="iRFDataTable" class="Tbl (strict)"("Active Cell"=w2073, "Cell BG Color"=w2065) -> ()  [unwired: 2 in, 2 out]
          n923 = Build Array(w2077, "No" ("element")) -> (w2075:string[])
          n924 = Bundle By Name(cluster=w2070, "Row"=w2069, "Column"=1) -> (w2071:T19)
          n925 = property on="iRFDataTable" class="Tbl (strict)"("Active Cell"=w2071, "Cell BG Color"=w2065) -> ()  [unwired: 2 in, 2 out]
        }
        "iRFDataTable" <- w2058
        n926 = call <vilib>:"Add State(s) to Queue__JKI_lib_State_Machine.vi"("State(s) in (\"\")"=w2064) -> ("States Out"=w2063:string)  [unwired: 14 in]
      }
      frame "UI: UpdateIRFDataTable" {
        w2093 = i32[] [0, 1]
        w2092 = T19 {"Row"=0, "Column"=0} ("Active Cell:Active Cell")
        # "Update iRF data table.\n(Change Status to yes, update table color)"
        n927 = local read "iRFDataTable"() -> (w2099:string[][])
        n928 = Unbundle By Name(w2098) -> ("iRFIdx"=w2091:i32)
        n929 = Decrement(x=w2091) -> (x-1=w2094:i32)
        n930 = Replace Array Subset(array=w2099, new element="Yes" ("new element/subarray"), index (row)=w2094, index (col)=1 ("disabled index (col)")) -> (w2095:string[][])
        n931 = for {
          tunnel: w2093 -> [w2111] mode=indexing
          tunnel: w2092 -> [w2113]
          tunnel: w2094 -> [w2112]
          # "Update cell BG color"
          n932 = Bundle By Name(cluster=w2113, "Row"=w2112, "Column"=w2111) -> (w2110:T19)
          n933 = property on="iRFDataTable" class="Tbl (strict)"("Active Cell"=w2110, "Cell BG Color"=u32 6618880 ("Active Cell:Cell Background Color")) -> ()  [unwired: 2 in, 2 out]
        }
        n934 = for {
          tunnel: w2093 -> [w2106] mode=indexing
          tunnel: w2092 -> [w2108]
          tunnel: w2091 -> [w2107]
          n935 = Bundle By Name(cluster=w2108, "Row"=w2107, "Column"=w2106) -> (w2105:T19)
          n936 = property on="iRFDataTable" class="Tbl (strict)"("Active Cell"=w2105, "Cell BG Color"=u32 16773632 ("Active Cell:Cell Background Color")) -> ()  [unwired: 2 in, 2 out]
        }
        n937 = local write "iRFDataTable"(w2095) -> ()
        n938 = call <vilib>:"Add State(s) to Queue__JKI_lib_State_Machine.vi"("State(s) in (\"\")"=w2103) -> ("States Out"=w2102:string)  [unwired: 14 in]
      }
      frame "UI: UpdateGainDataIndicators" {
        # "Update indicator for Gain data.\n(Update Arrays and tables)"
        n939 = Unbundle By Name(w2124) -> ("GainDataTemp.CtrlV"=w2115:dbl, "GainDataTemp.AUC"=w2114:dbl, "GainDataTemp.AUC Std"=w2123:dbl, "GainDataTemp.IntFactor"=w2122:dbl, "GainDataTemp.IntCorrAUC"=w2121:dbl)
        n940 = local read "Int Corr AUC"() -> (w2127:dbl[])
        n941 = Build Array(w2115, w2114, w2123, w2122, w2121) -> (w2120:dbl[])
        n942 = local read "Intensity Factor"() -> (w2130:dbl[])
        n943 = for {
          tunnel: w2120 -> [w2146] mode=indexing
          tunnel: [w2144] -> w2118 mode=indexing
          n944 = Number To Fractional String(number=w2146, precision (6)=i16 3) -> (F-format string=w2144:string)  [unwired: 2 in]
        }
        n945 = local read "AUC Std"() -> (w2133:dbl[])
        n946 = local read "AUC"() -> (w2139:dbl[])
        n947 = local read "Ctrl V"() -> (w2136:dbl[])
        n948 = Insert Into Array(array=w2139, index=0, new element=w2114) -> (→"AUC":dbl[])
        n949 = Insert Into Array(array=w2136, index=0, new element=w2115) -> (→"Ctrl V":dbl[])
        n950 = Insert Into Array(array=w2130, index=0, new element=w2122) -> (→"Intensity Factor":dbl[])
        n951 = Insert Into Array(array=w2127, index=0, new element=w2121) -> (→"Int Corr AUC":dbl[])
        n952 = Insert Into Array(array=w2133, index=0, new element=w2123) -> (→"AUC Std":dbl[])
        n953 = local read "GainDataTable"() -> (w2116:string[][])
        n954 = Insert Into Array(array=w2116, index (row)=0, new element=w2118) -> (→"GainDataTable":string[][])  [unwired: 1 in]
        n955 = call <vilib>:"Add State(s) to Queue__JKI_lib_State_Machine.vi"("State(s) in (\"\")"=w2143) -> ("States Out"=w2142:string)  [unwired: 14 in]
      }
      frame "UI: ShowDialog" {
        # "Show dialog ask user to adjust signal level\n(If OK aquire data, if abort stop auqisition)"
        n956 = local read "Task"() -> (w2147:enum32{"iRFAndGain", "Alignment"})
        n957 = case shown="\"Alignment\"" w2147 {
          tunnel: ["Please adjsut max signal level to around 1V." ("message") "Click OK to confirm data!" ("message")] -> w2153
          frame "iRFAndGain", Default {
          }
          frame "Alignment" {
          }
        }
        n958 = Two Button Dialog(message=w2153, 1:"Abort" ("F button name (\"Cancel\")"), 2:"OK" ("T button name (\"OK\")")) -> (T button?=w2150:bool)
        n959 = case shown="False" w2150 {
          tunnel: ["Macro: StopRun\nQueue: FlashDataAllQueue" ("State(s) in Front (\"\")") w2161] -> w2149
          tunnel: w2148 -> [_ w2161]
          frame False {
            # "Stop if abort"
          }
          frame True {
            # "Continue if OK"
          }
        }
        n960 = call <vilib>:"Add State(s) to Queue__JKI_lib_State_Machine.vi"("State(s) in Front (\"\")"=w2149) -> ("States Out"=w2157:string)  [unwired: 14 in]
      }
      frame "UI: WFAutoScale" {
        # "Set graph auto scale.\n(UI: WFAutoScale >> T/F)"
        n961 = Equal?(x=w2162, y="F") -> (x = y?=w2163:bool)
        n962 = Equal?(x=w2162, y="T") -> (x = y?=w2165:bool)
        n963 = case shown="True" w2165 {
          frame False {
          }
          frame True {
            n964 = property on="Waveform (no average)" class="WFGraph (strict)"("YScale.ScaleFit"=u8 2 ("Y Scale.Scale Fit")) -> ()  [unwired: 2 in, 2 out]
          }
        }
        n965 = case shown="True" w2163 {
          frame False {
          }
          frame True {
            n966 = property on="Waveform (no average)" class="WFGraph (strict)"("YScale.ScaleFit"=u8 0 ("Y Scale.Scale Fit")) -> (error out=w2173:errorcluster)  [unwired: 2 in, 1 out]
            n967 = property on="Waveform (no average)" class="WFGraph (strict)"(error in=w2173, "YScale.Maximum"=2.0 ("Y Scale.Range:Maximum")) -> (error out=w2172:errorcluster)  [unwired: 1 in, 1 out]
            n968 = property on="Waveform (no average)" class="WFGraph (strict)"(error in=w2172, "YScale.Minimum"=0.0 ("Y Scale.Range:Maximum")) -> ()  [unwired: 1 in, 2 out]
          }
        }
        n969 = call <vilib>:"Add State(s) to Queue__JKI_lib_State_Machine.vi"("State(s) in (\"\")"=w2171) -> ("States Out"=w2170:string)  [unwired: 14 in]
      }
      frame "UI: Initialize" {
        w2179 = T11."Disabled and Grayed Out" ("Disabled")
        # "Disable all button on startup"
        # "Initialize the User Interface, here.\n(this is called automatically, by the Macro: Init)"
        n970 = property on="Ctrl V" class="DigNum (strict)"("DisabledEnum"=w2179) -> ()  [unwired: 2 in, 2 out]
        n971 = property on="StopButton" class="Bool"("DisabledEnum"=w2179) -> ()  [unwired: 2 in, 2 out]
        n972 = property on="Sys Reconfig" class="Bool"("DisabledEnum"=w2179) -> ()  [unwired: 2 in, 2 out]
        n973 = property on="StartButton" class="Bool"("DisabledEnum"=w2179) -> ()  [unwired: 2 in, 2 out]
        n974 = property on="355nm Laser toggle" class="Bool (strict)"("DisabledEnum"=w2179) -> ()  [unwired: 2 in, 2 out]
        n975 = property on="Aiming beam toggle" class="Bool (strict)"("DisabledEnum"=w2179) -> ()  [unwired: 2 in, 2 out]
        n976 = property on="Ctrl V" class="DigNum (strict)"("Data Range"=T20 {"Minimum"=0.0, "Maximum"=5.5, "Increment"=0.1} ("Data Entry Limits")) -> ()  [unwired: 2 in, 2 out]
        n977 = call <vilib>:"Add State(s) to Queue__JKI_lib_State_Machine.vi"("State(s) in (\"\")"=w2184) -> ("States Out"=w2183:string)  [unwired: 14 in]
      }
      frame "UI: showDisclaimer" {
        # "Show disclamer window.\n(It is a separator no-op. You can make a copy of this frame to create a new UI frame)"
        n978 = call <vilib>:"Application Directory.vi"() -> ("Application Directory"=w2197:path)
        n979 = Build Path(base path=w2197, name or relative path="Disclamer.png") -> (appended path=w2195:path)
        n980 = property on="Disclamer" class="Pict"() -> ("Draw Area Size"=w2193:T34)  [unwired: 2 in, 2 out]
        n981 = call <vilib>:"Read PNG File.vi"("path to PNG file"=w2195) -> ("image data"=w2192:T35)  [unwired: 8 in, 2 out]
        n982 = disable-structure "Diagram Disable Structure" shown="Disabled" {
          frame Disabled {
            n983 = flat-sequence {
              frame #0 {
                n984 = call "disclaimer.vi"() -> ()  [unwired: 12 in]
              }
              frame #1 {
                n985 = Wait (ms)(milliseconds to wait=u32 250) -> ()  [unwired: 1 out]
              }
              frame #2 {
                n986 = call "SoftwareNote.vi"() -> ()  [unwired: 12 in]
              }
            }
          }
          frame Enabled {
          }
        }
        n987 = Unbundle By Name(w2192) -> ("Rectangle.right"=w2190:i16, "Rectangle.bottom"=w2188:i16)
        n988 = Unbundle By Name(w2193) -> ("Width"=w2191:u32, "Height"=w2189:u32)
        n989 = call <vilib>:"Draw Flattened Pixmap.vi"("image data"=w2192) -> ("new picture"=→"Disclamer":picture)  [unwired: 8 in]
        n990 = Divide(x=w2191, y=w2190) -> (x/y=w2187:dbl)
        n991 = Divide(x=w2189, y=w2188) -> (x/y=w2186:dbl)
        n992 = Max & Min(x=w2187, y=w2186) -> (min(x,y)=w2185:dbl)  [unwired: 1 out]
        n993 = property on="Disclamer" class="Pict"("ZoomFactor"=w2185) -> ()  [unwired: 2 in, 2 out]
        n994 = call <vilib>:"Add State(s) to Queue__JKI_lib_State_Machine.vi"("State(s) in (\"\")"=w2202) -> ("States Out"=w2201:string)  [unwired: 14 in]
      }
      frame "UI: SetButtonText" {
        # "Set button text of 355nm laser and aiming beam."
        n995 = call <vilib>:"Add State(s) to Queue__JKI_lib_State_Machine.vi"("State(s) in (\"\")"=w2208) -> ("States Out"=w2207:string)  [unwired: 14 in]
      }
      frame "UI: DuringAquisition" {
        w2209 = T11."Enabled" ("Disabled")
        w2214 = T11."Disabled and Grayed Out" ("Disabled")
        # "Do not put any code in this frame.\n(It is a separator no-op. You can make a copy of this frame to create a new UI frame)"
        n996 = property on="StopButton" class="Bool"("DisabledEnum"=w2209) -> ()  [unwired: 2 in, 2 out]
        n997 = property on="iRFSigInRange" class="Bool (strict)"("DisabledEnum"=w2209) -> ()  [unwired: 2 in, 2 out]
        n998 = property on="AcquireGain" class="Bool"("DisabledEnum"=w2209) -> ()  [unwired: 2 in, 2 out]
        n999 = property on="GainSigInRange" class="Bool (strict)"("DisabledEnum"=w2209) -> ()  [unwired: 2 in, 2 out]
        n1000 = property on="AcquireIRF" class="Bool"("DisabledEnum"=w2209) -> ()  [unwired: 2 in, 2 out]
        n1001 = Bundle By Name(cluster=w2212, "SysRunning?"=TRUE) -> (w2213:T22)
        n1002 = property on="StartButton" class="Bool"("DisabledEnum"=w2214) -> ()  [unwired: 2 in, 2 out]
        n1003 = property on="Sys Reconfig" class="Bool"("DisabledEnum"=w2214) -> ()  [unwired: 2 in, 2 out]
        n1004 = property on="355nm Laser toggle" class="Bool (strict)"("DisabledEnum"=w2214) -> ()  [unwired: 2 in, 2 out]
        n1005 = property on="Aiming beam toggle" class="Bool (strict)"("DisabledEnum"=w2214) -> ()  [unwired: 2 in, 2 out]
        n1006 = local write "GainInstSting"("Please set control voltage and make sure data is in range.\nClick 'Acquire' button to record data." ("GainInstSting")) -> ()
        n1007 = property on="Quit" class="Bool"("DisabledEnum"=w2214) -> ()  [unwired: 2 in, 2 out]
        n1008 = local write "iRFInstSting"("1. Click 'Set CtrlV' to set APD bias voltage\n2. Click 'Acquire' button to record data." ("iRFInstSting")) -> ()
        n1009 = property on="Laser Rep Rate" class="DigNum (strict)"("DisabledEnum"=w2214) -> ()  [unwired: 2 in, 2 out]
        n1010 = property on="Channel" class="RadioBtnsControl (strict)"("DisabledEnum"=w2214) -> ()  [unwired: 2 in, 2 out]
        n1011 = property on="Task" class="RadioBtnsControl (strict)"("DisabledEnum"=w2214) -> ()  [unwired: 2 in, 2 out]
        n1012 = call <vilib>:"Add State(s) to Queue__JKI_lib_State_Machine.vi"("State(s) in (\"\")"=w2219) -> ("States Out"=w2218:string)  [unwired: 14 in]
      }
      frame "UI: ReadyForAquisition" {
        w2220 = T11."Disabled and Grayed Out" ("Disabled")
        w2226 = T11."Enabled" ("Disabled")
        # "Do not put any code in this frame.\n(It is a separator no-op. You can make a copy of this frame to create a new UI frame)"
        n1013 = local read "Channel"() -> (w2222:enum32{"Ch1", "Ch2", "Ch3", "Ch4"})
        n1014 = property on="StopButton" class="Bool"("DisabledEnum"=w2220) -> ()  [unwired: 2 in, 2 out]
        n1015 = property on="AcquireGain" class="Bool"("DisabledEnum"=w2220) -> ()  [unwired: 2 in, 2 out]
        n1016 = property on="iRFSigInRange" class="Bool (strict)"("DisabledEnum"=w2220) -> ()  [unwired: 2 in, 2 out]
        n1017 = property on="GainSigInRange" class="Bool (strict)"("DisabledEnum"=w2220) -> ()  [unwired: 2 in, 2 out]
        n1018 = property on="AcquireIRF" class="Bool"("DisabledEnum"=w2220) -> ()  [unwired: 2 in, 2 out]
        n1019 = Bundle By Name(cluster=w2224, "SysRunning?"=FALSE) -> (w2225:T22)
        n1020 = case shown="\"Ch2\"" w2222 {
          tunnel: ["To aquire gain data:\n1. Place blue Chroma slide as close as possible to the fiber port! \n2. Start data aquisition." ("GainInstSting") "To aquire gain data:\n1. Place blue Chroma slide as close as possible to the fiber port! \n2. Start data aquisition." ("GainInstSting") "To aquire gain data:\n1. Place green Chroma slide as close as possible to the fiber port! \n2. Remove Channel 3 bandpass filter!\n3. Start data aquisition." ("GainInstSting")] -> w2223
          tunnel: ["To aquire gain data:\n1. Install Thorlabs fiber stop! \n2. Start data aquisition." ("GainInstSting") "To aquire gain data:\n1. Install Thorlabs fiber stop! \n2. Start data aquisition." ("GainInstSting") "To aquire gain data:\n1. Install fiber probe!\n2. Place DASPI solution as close as possible to fiber probe.\n3. Remove Channel 3 bandpass filter. \n4. Start data aquisition." ("GainInstSting")] -> w2221
          frame "Ch1", Default {
          }
          frame "Ch2" {
          }
          frame "Ch3" {
          }
        }
        "GainInstSting" <- w2223
        "iRFInstSting" <- w2221
        n1021 = property on="StartButton" class="Bool"("DisabledEnum"=w2226) -> ()  [unwired: 2 in, 2 out]
        n1022 = property on="Sys Reconfig" class="Bool"("DisabledEnum"=w2226) -> ()  [unwired: 2 in, 2 out]
        n1023 = property on="355nm Laser toggle" class="Bool (strict)"("DisabledEnum"=w2226) -> ()  [unwired: 2 in, 2 out]
        n1024 = property on="Aiming beam toggle" class="Bool (strict)"("DisabledEnum"=w2226) -> ()  [unwired: 2 in, 2 out]
        n1025 = property on="Quit" class="Bool"("DisabledEnum"=w2226) -> ()  [unwired: 2 in, 2 out]
        n1026 = property on="Channel" class="RadioBtnsControl (strict)"("DisabledEnum"=w2226) -> ()  [unwired: 2 in, 2 out]
        n1027 = property on="Laser Rep Rate" class="DigNum (strict)"("DisabledEnum"=w2226) -> ()  [unwired: 2 in, 2 out]
        n1028 = property on="Task" class="RadioBtnsControl (strict)"("DisabledEnum"=w2226) -> ()  [unwired: 2 in, 2 out]
        n1029 = call <vilib>:"Add State(s) to Queue__JKI_lib_State_Machine.vi"("State(s) in Front (\"\")"="LED: Green" ("State(s) in Front (\"\")"), "State(s) in (\"\")"=w2232) -> ("States Out"=w2231:string)  [unwired: 13 in]
      }
      frame "UI: Update" {
        # "Do not put any code in this frame.\n(It is a separator no-op. You can make a copy of this frame to create a new UI frame)"
        n1030 = Unbundle By Name(w2246) -> ("System Status"=→"System Hardware Connection Status":T1, "IDs.RunID"=→"Run #":i8, "FLImDAQ"=→"FLImDAQ":T27, "SysRunning?"=→"System Status:":bool, "LJ Pinout"=→"LJ Pinout":T3, "IDs.BG ID"=→"BG #":i8, "IDs.Cali ID"=→"Calibration #":i8)
        n1031 = call <vilib>:"Add State(s) to Queue__JKI_lib_State_Machine.vi"("State(s) in (\"\")"=w2250) -> ("States Out"=w2249:string)  [unwired: 14 in]
      }
      frame "UI: Cursor Set" {
        # "Argument"
        # "Set and Unset Cursor Busy.\n(Usage: \"UI: Cursor Set >> Busy|Idle\")"
        n1032 = case shown="\"Idle\", Default" w2252 {
          tunnel: w2254 -> [w2259 w2261]
          tunnel: [w2258 w2260] -> w2253
          frame "Idle", Default {
            n1033 = call <vilib>:"Unset Busy.vi"("error in (no error)"=w2259) -> ("error out"=w2258:errorcluster)  [unwired: 10 in]
          }
          frame "Busy" {
            n1034 = call <vilib>:"Set Busy.vi"("error in (no error)"=w2261) -> ("error out"=w2260:errorcluster)  [unwired: 9 in, 1 out]
          }
        }
        n1035 = call <vilib>:"Add State(s) to Queue__JKI_lib_State_Machine.vi"("State(s) in (\"\")"=w2257) -> ("States Out"=w2256:string)  [unwired: 14 in]
      }
      frame "UI: Front Panel State" {
        # "Argument"
        # "Set Front Panel Open or Closed\n(Usage: \"UI: Front Panel State >> Open|Close\")"
        n1036 = Unbundle By Name(w2262) -> ("Core.Current VI Reference"=w2265:refnum<vi>)
        n1037 = case shown="\"Open\", \"Standard\", Default" w2264 {
          tunnel: w2267 -> [w2275 w2288 w2299 w2311 w2323]
          tunnel: [w2276 w2289 w2300 w2312 w2324] -> w2266
          tunnel: w2265 -> [_ _ _ _ _]
          frame "Open", "Standard", Default {
            w2270 = T14."Standard" ("State")
            n1038 = property on="Property Node" class="VI"(error in=w2275) -> (reference out=w2273:refnum<vi>, error out=w2274:errorcluster, "FP.State"=w2272:T14)  [unwired: 1 in]
            n1039 = Not Equal?(x=w2272, y=w2270) -> (x != y?=w2271:bool)
            n1040 = case shown="True" w2271 {
              tunnel: [w2280 w2282] -> w2276
              tunnel: w2274 -> [w2279 w2282]
              tunnel: w2273 -> [w2278 _]
              tunnel: w2270 -> [w2277 _]
              frame True {
                n1041 = invoke on="Invoke Node" class="VI" method="FP.Open"(reference=w2278, error in=w2279, "Activate"=TRUE, "State"=w2277) -> (error out=w2280:errorcluster)  [unwired: 1 in, 4 out]
              }
              frame False {
              }
            }
          }
          frame "Close", "Closed" {
            n1042 = property on="Property Node" class="VI"(error in=w2288) -> (reference out=w2286:refnum<vi>, error out=w2287:errorcluster, "FP.State"=w2284:T14)  [unwired: 1 in]
            n1043 = Not Equal?(x=w2284, y=T14."Closed" ("Front Panel Window:State")) -> (x != y?=w2283:bool)
            n1044 = case shown="True" w2283 {
              tunnel: [w2290 w2293] -> w2289
              tunnel: w2287 -> [w2290 w2292]
              tunnel: w2286 -> [_ w2291]
              frame False {
              }
              frame True {
                n1045 = invoke on="Invoke Node" class="VI" method="FP.Close"(reference=w2291, error in=w2292) -> (error out=w2293:errorcluster)  [unwired: 1 in, 2 out]
              }
            }
          }
          frame "Hidden", "Hide" {
            w2294 = T14."Hidden" ("State")
            n1046 = property on="Property Node" class="VI"(error in=w2299) -> (reference out=w2297:refnum<vi>, error out=w2298:errorcluster, "FP.State"=w2296:T14)  [unwired: 1 in]
            n1047 = Not Equal?(x=w2296, y=w2294) -> (x != y?=w2295:bool)
            n1048 = case shown="True" w2295 {
              tunnel: [w2304 w2305] -> w2300
              tunnel: w2298 -> [w2303 w2305]
              tunnel: w2297 -> [w2302 _]
              tunnel: w2294 -> [w2301 _]
              frame True {
                n1049 = invoke on="Invoke Node" class="VI" method="FP.Open"(reference=w2302, error in=w2303, "State"=w2301) -> (error out=w2304:errorcluster)  [unwired: 2 in, 4 out]
              }
              frame False {
              }
            }
          }
          frame "Minimize", "Minimized" {
            w2306 = T14."Minimized" ("State")
            n1050 = property on="Property Node" class="VI"(error in=w2311) -> (reference out=w2309:refnum<vi>, error out=w2310:errorcluster, "FP.State"=w2308:T14)  [unwired: 1 in]
            n1051 = Not Equal?(x=w2308, y=w2306) -> (x != y?=w2307:bool)
            n1052 = case shown="True" w2307 {
              tunnel: [w2316 w2317] -> w2312
              tunnel: w2310 -> [w2315 w2317]
              tunnel: w2309 -> [w2314 _]
              tunnel: w2306 -> [w2313 _]
              frame True {
                n1053 = invoke on="Invoke Node" class="VI" method="FP.Open"(reference=w2314, error in=w2315, "State"=w2313) -> (error out=w2316:errorcluster)  [unwired: 2 in, 4 out]
              }
              frame False {
              }
            }
          }
          frame "Maximize", "Maximized" {
            w2318 = T14."Maximized" ("State")
            n1054 = property on="Property Node" class="VI"(error in=w2323) -> (reference out=w2321:refnum<vi>, error out=w2322:errorcluster, "FP.State"=w2320:T14)  [unwired: 1 in]
            n1055 = Not Equal?(x=w2320, y=w2318) -> (x != y?=w2319:bool)
            n1056 = case shown="True" w2319 {
              tunnel: [w2328 w2329] -> w2324
              tunnel: w2322 -> [w2327 w2329]
              tunnel: w2321 -> [w2326 _]
              tunnel: w2318 -> [w2325 _]
              frame True {
                n1057 = invoke on="Invoke Node" class="VI" method="FP.Open"(reference=w2326, error in=w2327, "State"=w2325) -> (error out=w2328:errorcluster)  [unwired: 2 in, 4 out]
              }
              frame False {
              }
            }
          }
        }
        n1058 = call <vilib>:"Add State(s) to Queue__JKI_lib_State_Machine.vi"("State(s) in (\"\")"=w2269) -> ("States Out"=w2268:string)  [unwired: 14 in]
      }
      frame "---------- 355 Laser ----------" {
        # "Template Separator\n(You can make a copy of, or modify, this frame)"
        n1059 = call <vilib>:"Add State(s) to Queue__JKI_lib_State_Machine.vi"("State(s) in (\"\")"=w2334) -> ("States Out"=w2333:string)  [unwired: 14 in]
      }
      frame "355 Laser: Check Dewelling" {
        # "if time laser start time is less than 7.5s before, wait 250ms then check again."
        # "Check laser timer\n(Check laser timer, make sure enough time lapsed after laser enable)"
        n1060 = Unbundle By Name(w2336) -> ("Laser start tic"=w2335:u32)
        n1061 = Tick Count (ms)() -> (millisecond timer value=w2341:u32)
        n1062 = Subtract(x=w2341, y=w2335) -> (x-y=w2340:u32)
        n1063 = Greater?(x=w2340, y=u32 5000) -> (0:w2338:bool)
        n1064 = case shown="False" w2338 {
          tunnel: ["355 Laser: Check Dewelling" ""] -> w2337
          frame False {
            n1065 = Wait (ms)(milliseconds to wait=u32 500) -> ()  [unwired: 1 out]
          }
          frame True {
          }
        }
        n1066 = call <vilib>:"Add State(s) to Queue__JKI_lib_State_Machine.vi"("State(s) in Front (\"\")"=w2337, "State(s) in (\"\")"=w2345) -> ("States Out"=w2344:string)  [unwired: 13 in]
      }
      frame "355 Laser: Laser enable" {
        # "Laser enable/disable\n(Usage: \"LabJack: Laser enable/disable >> 1|0\")"
        n1067 = Unbundle By Name(w2350) -> ("LJ Pinout.Laser Start/Stop"=w2356:string, "System Status.355 Laser"=w2349:bool)
        n1068 = case shown="False" w2349 {
          tunnel: w2352 -> [w2371 w2372]
          tunnel: w2356 -> [w2359 _]
          tunnel: [w2361 w2372] -> w2354
          tunnel: [w2360 u32 0 ("millisecond timer value")] -> w2353
          frame False {
            n1069 = call "LabJack_FGV.vi"("Operation(Read)"=enum16{"Write", "Read"}."Read" ("Operation")) -> ("Read data"=w2367:i32)  [unwired: 9 in, 1 out]
            n1070 = call "LJM_eWriteName.vi"("Handle In"=w2367, "Name"=w2359, "Value"=1.0, "error in"=w2371) -> ("Handle Out"=w2366:i32, "error out"=w2365:errorcluster)  [unwired: 10 in]
            n1071 = call <userlib>:"Wait (ms)__ogtk.vi"("error in (no error)"=w2365, "milliseconds to wait"=u32 250) -> ("error out"=w2364:errorcluster)  [unwired: 8 in, 1 out]
            n1072 = call "LJM_eWriteName.vi"("Handle In"=w2366, "Name"=w2359, "Value"=0.0, "error in"=w2364) -> ("error out"=w2362:errorcluster)  [unwired: 10 in, 1 out]
            n1073 = call <userlib>:"Tick Count (ms)__ogtk.vi"("error in (no error)"=w2362) -> ("error out"=w2361:errorcluster, "millisecond timer value"=w2360:u32)  [unwired: 9 in]
          }
          frame True {
          }
        }
        n1074 = Bundle By Name(cluster=w2350, "Laser start tic"=w2353) -> (w2351:T22)
        n1075 = call <vilib>:"Add State(s) to Queue__JKI_lib_State_Machine.vi"("State(s) in (\"\")"=w2358) -> ("States Out"=w2357:string)  [unwired: 14 in]
      }
      frame "355 Laser: Laser disable" {
        # "Laser enable/disable\n(Usage: \"LabJack: Laser enable/disable >> 1|0\")"
        n1076 = Unbundle By Name(w2375) -> ("LJ Pinout.Laser Start/Stop"=w2380:string, "System Status.355 Laser"=w2374:bool)
        n1077 = case shown="True" w2374 {
          tunnel: w2381 -> [w2384 w2398]
          tunnel: w2380 -> [_ w2386]
          tunnel: [w2384 w2388] -> w2378
          tunnel: [u32 0 ("millisecond timer value") w2387] -> w2377
          frame False {
          }
          frame True {
            n1078 = call "LabJack_FGV.vi"("Operation(Read)"=enum16{"Write", "Read"}."Read" ("Operation")) -> ("Read data"=w2394:i32)  [unwired: 9 in, 1 out]
            n1079 = call "LJM_eWriteName.vi"("Handle In"=w2394, "Name"=w2386, "Value"=1.0, "error in"=w2398) -> ("Handle Out"=w2393:i32, "error out"=w2392:errorcluster)  [unwired: 10 in]
            n1080 = call <userlib>:"Wait (ms)__ogtk.vi"("error in (no error)"=w2392, "milliseconds to wait"=u32 250) -> ("error out"=w2391:errorcluster)  [unwired: 8 in, 1 out]
            n1081 = call "LJM_eWriteName.vi"("Handle In"=w2393, "Name"=w2386, "Value"=0.0, "error in"=w2391) -> ("error out"=w2389:errorcluster)  [unwired: 10 in, 1 out]
            n1082 = call <userlib>:"Tick Count (ms)__ogtk.vi"("error in (no error)"=w2389) -> ("error out"=w2388:errorcluster, "millisecond timer value"=w2387:u32)  [unwired: 9 in]
          }
        }
        n1083 = Bundle By Name(cluster=w2375, "Laser start tic"=w2377) -> (w2376:T22)
        n1084 = call <vilib>:"Add State(s) to Queue__JKI_lib_State_Machine.vi"("State(s) in (\"\")"=w2383) -> ("States Out"=w2382:string)  [unwired: 14 in]
      }
      frame "355 Laser: Dewelling" {
        # "Wait some time (ms)\n(355 Laser: Dewelling >> #)"
        n1085 = Fract/Exp String To Number(string=w2402, default (0 dbl)=0) -> (number=w2400:i32)  [unwired: 2 in, 1 out]
        n1086 = Wait (ms)(milliseconds to wait=w2400) -> ()  [unwired: 1 out]
        n1087 = call <vilib>:"Add State(s) to Queue__JKI_lib_State_Machine.vi"("State(s) in (\"\")"=w2406) -> ("States Out"=w2405:string)  [unwired: 14 in]
      }
      frame "355 Laser: Init" {
        # "Initilize 355nm laser\n(Start laser, enable interlock)"
        n1088 = call <vilib>:"Add State(s) to Queue__JKI_lib_State_Machine.vi"("State(s) in Front (\"\")"="355 Laser: CheckControllerStatus", "State(s) in (\"\")"=w2412) -> ("States Out"=w2411:string)  [unwired: 13 in]
      }
      frame "355 Laser: Close" {
        # "Template Separator\n(You can make a copy of, or modify, this frame)"
        n1089 = call <vilib>:"Add State(s) to Queue__JKI_lib_State_Machine.vi"("State(s) in Front (\"\")"="355 Laser: CheckControllerStatus\n355 Laser: Laser disable\n355 Laser: Dewelling >>1000", "State(s) in (\"\")"=w2418) -> ("States Out"=w2417:string)  [unwired: 13 in]
      }
      frame "355 Laser: CheckControllerStatus" {
        # "if average < 1, laser on\nif average > 9, laser off\nif 1<average<9, interlock open, blink indicator"
        # "take 10 measuremt and look at average"
        # "Check 355 laser controller status\nBy probing Emisison Lamp negative terminal voltage"
        n1090 = Unbundle By Name(w2419) -> ("LJ Pinout.Laser Ready"=w2429:string)
        n1091 = call "LabJack_FGV.vi"("Operation(Read)"=enum16{"Write", "Read"}."Read" ("Operation")) -> ("Read data"=w2430:i32)  [unwired: 9 in, 1 out]
        n1092 = for {
          N: 10 -> [_]
          tunnel: w2430 -> [w2464]
          tunnel: w2429 -> [w2459]
          shift-right: [w2463] -> w2423
          shift-left: w2428 -> [w2462]
          tunnel: [w2460] -> w2421 mode=indexing
          n1093 = call "LJM_eReadName.vi"("Handle In"=w2464, "Name"=w2459, "error in"=w2462) -> ("Value"=w2460:dbl, "error out"=w2463:errorcluster)  [unwired: 10 in, 1 out]
          n1094 = Wait (ms)(milliseconds to wait=u32 50) -> ()  [unwired: 1 out]
        }
        n1095 = case shown="No Error" w2423 {
          selector: w2423 -> [w2438 w2457]
          tunnel: [w2440 FALSE] -> w2425
          tunnel: [w2439 w2457] -> w2424
          tunnel: [w2434 nan] -> w2422
          tunnel: w2421 -> [w2436 _]
          frame No Error {
            n1096 = call-poly <vilib>:"Mean.vi"("X"=w2436) -> ("mean"=w2434:dbl)  [unwired: 1 out]
            n1097 = Less?(x=w2434, y=9.3) -> (x < y?=w2435:bool)
            n1098 = case shown="False" w2435 {
              tunnel: [w2443 TRUE] -> w2440
              tunnel: w2434 -> [w2446 _]
              tunnel: w2438 -> [w2442 w2453]
              tunnel: [w2441 w2453] -> w2439
              frame False {
                n1099 = Greater?(x=w2446, y=10.0) -> (0:w2444:bool)
                n1100 = case shown="True" w2444 {
                  tunnel: [FALSE FALSE] -> w2443
                  tunnel: w2442 -> [_ w2450]
                  tunnel: [errorcluster {"status"=TRUE, "code"=5002, "source"="355 Laser"} ("error out") w2450] -> w2441
                  frame False {
                    n1101 = property on="355 Laser" class="Bool (strict)"("Blinking"=FALSE) -> ()  [unwired: 2 in, 2 out]
                  }
                  frame True {
                    n1102 = property on="355 Laser" class="Bool (strict)"("Blinking"=FALSE) -> ()  [unwired: 2 in, 2 out]
                  }
                }
              }
              frame True {
                n1103 = property on="355 Laser" class="Bool (strict)"("Blinking"=FALSE) -> ()  [unwired: 2 in, 2 out]
              }
            }
          }
          frame Error {
          }
        }
        "laser EM lamp V" <- w2422
        n1104 = Bundle By Name(cluster=w2419, "System Status.355 Laser"=w2425) -> (w2420:T22)
        n1105 = call <vilib>:"Add State(s) to Queue__JKI_lib_State_Machine.vi"("State(s) in (\"\")"=w2433) -> ("States Out"=w2432:string)  [unwired: 14 in]
      }
      frame "355 Laser: CheckPWMStatus" {
        # "Check 355 laser PWM status\n(Read LJ DIO#EF_ENABLE register to determine PWM status)"
        n1106 = Unbundle By Name(w2465) -> ("LJ Pinout.355 PWM"=w2466:string)
        n1107 = call "LabJack_FGV.vi"("Operation(Read)"=enum16{"Write", "Read"}."Read" ("Operation"), "error in (no error)"=w2469) -> ("error out"=w2472:errorcluster, "Read data"=w2473:i32)  [unwired: 8 in]
        n1108 = Concatenate Strings(w2466, "_EF_ENABLE" ("string")) -> (w2471:string)
        n1109 = call "LJM_eReadName.vi"("Handle In"=w2473, "Name"=w2471, "error in"=w2472) -> ("Value"=w2468:dbl, "error out"=w2470:errorcluster)  [unwired: 10 in, 1 out]
        n1110 = Greater Than 0?(x=w2468) -> (x > 0?=w2467:bool)
        n1111 = case shown="False" w2467 {
          frame False {
            # "PWM is off\nset color to gray"
            n1112 = local write "355nm Laser toggle"(FALSE ("355nm Laser")) -> ()
          }
          frame True {
            # "PWM is on\nset color to light green"
            n1113 = local write "355nm Laser toggle"(TRUE ("355nm Laser")) -> ()
          }
        }
        n1114 = call <vilib>:"Add State(s) to Queue__JKI_lib_State_Machine.vi"("State(s) in (\"\")"=w2478) -> ("States Out"=w2477:string)  [unwired: 14 in]
      }
      frame "355 Laser: Start" {
        # "Template Separator\n(You can make a copy of, or modify, this frame)"
        n1115 = call <vilib>:"Add State(s) to Queue__JKI_lib_State_Machine.vi"("State(s) in Front (\"\")"="LabJack: 355_PWM_Start", "State(s) in (\"\")"=w2486) -> ("States Out"=w2485:string)  [unwired: 13 in]
      }
      frame "355 Laser: Stop" {
        # "Template Separator\n(You can make a copy of, or modify, this frame)"
        n1116 = call <vilib>:"Add State(s) to Queue__JKI_lib_State_Machine.vi"("State(s) in Front (\"\")"="LabJack: 355_PWM_Stop", "State(s) in (\"\")"=w2492) -> ("States Out"=w2491:string)  [unwired: 13 in]
      }
      frame "---------- Utility ----------" {
        # "Template Separator\n(You can make a copy of, or modify, this frame)"
        n1117 = call <vilib>:"Add State(s) to Queue__JKI_lib_State_Machine.vi"("State(s) in (\"\")"=w2497) -> ("States Out"=w2496:string)  [unwired: 14 in]
      }
      frame "Utility: EnableGain?" {
        # "Enable or disable control V numeric control\n(Utility: EnableGain? >> True|False)"
        n1118 = case shown="\"True\", Default" w2498 {
          frame "False" {
            n1119 = property on="Ctrl V" class="DigNum (strict)"("DisabledEnum"=T11."Disabled and Grayed Out" ("Disabled")) -> ()  [unwired: 2 in, 2 out]
          }
          frame "True", Default {
            n1120 = property on="Ctrl V" class="DigNum (strict)"("DisabledEnum"=T11."Enabled" ("Disabled")) -> ()  [unwired: 2 in, 2 out]
          }
        }
        n1121 = call <vilib>:"Add State(s) to Queue__JKI_lib_State_Machine.vi"("State(s) in (\"\")"=w2503) -> ("States Out"=w2502:string)  [unwired: 14 in]
      }
      frame "Utility: SetDefaultMaxV" {
        # "Template Separator\n(You can make a copy of, or modify, this frame)"
        n1122 = local read "Ch1 Max CtrlV"() -> (w2506:dbl)
        n1123 = local write "Gain High"(w2506) -> ()
        n1124 = call <vilib>:"Add State(s) to Queue__JKI_lib_State_Machine.vi"("State(s) in (\"\")"=w2511) -> ("States Out"=w2510:string)  [unwired: 14 in]
      }
      frame "Utility: setSaveFlag" {
        # "Template Separator\n(You can make a copy of, or modify, this frame)"
        n1125 = Fract/Exp String To Number(string=w2512, default (0 dbl)=u8 0) -> (number=w2514:u8)  [unwired: 2 in, 1 out]
        n1126 = case shown="0, Default" w2514 {
          tunnel: [FALSE TRUE] -> w2513
          frame 0, Default {
          }
          frame 1 {
          }
        }
        n1127 = local write "SaveData?"(w2513) -> ()
        n1128 = call <vilib>:"Add State(s) to Queue__JKI_lib_State_Machine.vi"("State(s) in (\"\")"=w2520) -> ("States Out"=w2519:string)  [unwired: 14 in]
      }
      frame "Utility: Dewelling" {
        # "Main loop dewell\n(Dewelling >> #)"
        n1129 = Fract/Exp String To Number(string=w2525, default (0 dbl)=0) -> (number=w2523:i32)  [unwired: 2 in, 1 out]
        n1130 = Wait (ms)(milliseconds to wait=w2523) -> ()  [unwired: 1 out]
        n1131 = call <vilib>:"Add State(s) to Queue__JKI_lib_State_Machine.vi"("State(s) in (\"\")"=w2530) -> ("States Out"=w2529:string)  [unwired: 14 in]
      }
      frame "Utility: SetAllChanManualGain" {
        # "Template Separator\n(You can make a copy of, or modify, this frame)"
        n1132 = property on="Auto gain" class="Bool (strict)"("Val(Sgnl)"=FALSE ("Value (Signaling)")) -> ()  [unwired: 2 in, 2 out]
        n1133 = call <vilib>:"Add State(s) to Queue__JKI_lib_State_Machine.vi"("State(s) in (\"\")"=w2536) -> ("States Out"=w2535:string)  [unwired: 14 in]
      }
      frame "Utility: SetAllChanAutoGain" {
        # "Template Separator\n(You can make a copy of, or modify, this frame)"
        n1134 = property on="Auto gain" class="Bool (strict)"("Val(Sgnl)"=TRUE ("Value (Signaling)")) -> ()  [unwired: 2 in, 2 out]
        n1135 = call <vilib>:"Add State(s) to Queue__JKI_lib_State_Machine.vi"("State(s) in (\"\")"=w2542) -> ("States Out"=w2541:string)  [unwired: 14 in]
      }
      frame "---------- Graph ----------" {
        # "Template Separator\n(You can make a copy of, or modify, this frame)"
        n1136 = call <vilib>:"Add State(s) to Queue__JKI_lib_State_Machine.vi"("State(s) in (\"\")"=w2547) -> ("States Out"=w2546:string)  [unwired: 14 in]
      }
      frame "Graph: ClearHistory" {
        # "Clear intensity trace history\n(You can make a copy of, or modify, this frame)"
        n1137 = property on="Waveform Chart" class="WFChart (strict)"("History Data"=dbl[] []) -> ()  [unwired: 2 in, 2 out]
        n1138 = call <vilib>:"Add State(s) to Queue__JKI_lib_State_Machine.vi"("State(s) in (\"\")"=w2553) -> ("States Out"=w2552:string)  [unwired: 14 in]
      }
      frame "Graph: SetXScale" {
        # "Set X scale multiplier\n(Check digitizer aquisition speed and update x scale)"
        n1139 = local read "Channel"() -> (w2558:enum32{"Ch1", "Ch2", "Ch3", "Ch4"})
        n1140 = case shown="\"Ch1\", \"Ch2\", Default" w2558 {
          tunnel: w2557 -> [w2569 w2572]
          tunnel: [w2568 w2570] -> w2556
          tunnel: [w2567 w2571] -> w2555
          frame "Ch1", "Ch2", Default {
            n1141 = call "Digitizer1_FGV.vi"("error in (no error)"=w2569) -> ("error out"=w2568:errorcluster, "Read data"=w2567:refnum<k15>)  [unwired: 9 in]
          }
          frame "Ch3" {
            n1142 = call "Digitizer2_FGV.vi"("error in (no error)"=w2572) -> ("error out"=w2570:errorcluster, "Read data"=w2571:refnum<k15>)  [unwired: 9 in]
          }
        }
        n1143 = property on="Property Node" class="niScope"(reference=w2555, error in=w2556) -> (error out=w2560:errorcluster, "Min Sample Rate"=w2562:dbl)  [unwired: 1 out]
        n1144 = Divide(x=1.0, y=w2562) -> (x/y=w2561:dbl)
        "dt (s)" <- w2561
        n1145 = property on="Waveform (no average)" class="WFGraph (strict)"(error in=w2560, "XScale.Multiplier"=w2561) -> (error out=w2559:errorcluster)  [unwired: 1 in, 1 out]
        n1146 = call <vilib>:"Add State(s) to Queue__JKI_lib_State_Machine.vi"("State(s) in (\"\")"=w2566) -> ("States Out"=w2565:string)  [unwired: 14 in]
      }
      frame "Graph: AddCursors" {
        # "Add BG and DC cursor to all graphs\n(You can make a copy of, or modify, this frame)"
        n1147 = property on="Waveform (no average)" class="WFGraph (strict)"(error in=w2594) -> ("CrsrList"=w2580:T36, "XScale.Maximum"=w2588:dbl)  [unwired: 1 in, 2 out]
        n1148 = Multiply(x=w2588, y=0.8) -> (x*y=w2591:dbl)
        n1149 = Multiply(x=w2588, y=0.1) -> (x*y=w2584:dbl)
        n1150 = Multiply(x=w2588, y=0.9) -> (x*y=w2586:dbl)
        n1151 = Multiply(x=w2588, y=0.2) -> (x*y=w2583:dbl)
        n1152 = Build Array(w2591, w2586, w2584, w2583) -> (w2585:dbl[])
        n1153 = Index Array(array=w2580, index=4) -> (element=w2578:T37)
        n1154 = for {
          N: 4 -> [_]
          tunnel: w2580 -> [w2604] mode=indexing
          tunnel: w2585 -> [w2602] mode=indexing
          tunnel: [w2603] -> w2575 mode=indexing
          tunnel: u32[] [6618880, 6618880, 16711680, 16711680] -> [w2601] mode=indexing
          n1155 = Bundle By Name(cluster=w2604, "Position.X"=w2602, "Color"=w2601) -> (w2603:T37)
        }
        n1156 = Bundle By Name(cluster=w2578, "Position.Y"=0.0, "Color"=u32 6618880) -> (w2574:T37)
        n1157 = Build Array (concatenate)(w2575, w2574) -> (w2573:T38)
        n1158 = control-ref of="Waveform (no average)"() -> (w2582:refnum<vi>)
        n1159 = property on="Waveform (no average)" class="WFGraph (strict)"("CrsrList"=w2573) -> (error out=w2593:errorcluster)  [unwired: 2 in, 1 out]
        n1160 = call "UpdateCurserIdx(SubVI).vi"("error in (no error)"=w2593, "WaveformGraph in"=w2582) -> ("error out"=w2595:errorcluster)  [unwired: 9 in]
        n1161 = call <vilib>:"Add State(s) to Queue__JKI_lib_State_Machine.vi"("State(s) in (\"\")"=w2600) -> ("States Out"=w2599:string)  [unwired: 14 in]
      }
      frame "---------- APD ----------" {
        # "Template Separator\n(You can make a copy of, or modify, this frame)"
        n1162 = call <vilib>:"Add State(s) to Queue__JKI_lib_State_Machine.vi"("State(s) in (\"\")"=w2609) -> ("States Out"=w2608:string)  [unwired: 14 in]
      }
      frame "APD: Initialize" {
        w2610 = enum16{"Read", "Write"}."Write" ("Operation (Read)")
        w2613 = refnum<class "APDClass.lvclass"> refnum  # APDClass.lvclass
        # "Initialize APD FVG\n(You can make a copy of, or modify, this frame)"
        n1163 = call "APD2FGV.vi"("Error In"=w2612, "Operation (Read)"=w2610, "APDClass in"=w2613) -> ("Error Out"=w2614:errorcluster)  [unwired: 7 in, 1 out]
        n1164 = call "APD1FGV.vi"("Error In"=w2612, "Operation (Read)"=w2610, "APDClass in"=w2613) -> ("Error Out"=w2615:errorcluster)  [unwired: 7 in, 1 out]
        n1165 = call "APD4FGV.vi"("Error In"=w2612, "Operation (Read)"=w2610, "APDClass in"=w2613) -> ("Error Out"=w2611:errorcluster)  [unwired: 7 in, 1 out]
        n1166 = call "APD3FGV.vi"("Error In"=w2612, "Operation (Read)"=w2610, "APDClass in"=w2613) -> ("Error Out"=w2617:errorcluster)  [unwired: 7 in, 1 out]
        n1167 = Merge Errors(w2615, w2614, w2617, w2611) -> (w2616:errorcluster)
        n1168 = call <vilib>:"Add State(s) to Queue__JKI_lib_State_Machine.vi"("State(s) in (\"\")"=w2621) -> ("States Out"=w2620:string)  [unwired: 14 in]
      }
      frame "APD: LoadFromSerial" {
        # "Load APD info based on serial numbers\n(update FGV)"
        n1169 = call "readAPDSerial.vi"("Error In"=w2627) -> ("Error Out"=w2624:errorcluster, "output cluster"=w2625:T39)  [unwired: 9 in]
        n1170 = local read "Channel"() -> (w2626:enum32{"Ch1", "Ch2", "Ch3", "Ch4"})
        n1171 = case shown="\"Ch1\", Default" w2626 {
          tunnel: w2625 -> [w2639 w2645 w2651 w2658]
          tunnel: w2624 -> [w2635 w2643 w2649 w2656]
          tunnel: enum16{"Read", "Write"}."Write" ("Operation (Read)") -> [w2634 w2640 w2648 w2654]
          tunnel: [w2633 w2641 w2647 w2655] -> w2622
          frame "Ch1", Default {
            n1172 = Unbundle By Name(w2639) -> ("Ch1APDSerial#"=w2636:string)
            n1173 = call "CreatFromSerialNum.vi"("error in (no error)"=w2635, "APD Serial #"=w2636) -> ("error out"=w2638:errorcluster, "APDClass out"=w2637:refnum<class "APDClass.lvclass">)  [unwired: 8 in]
            n1174 = call "APD1FGV.vi"("Error In"=w2638, "Operation (Read)"=w2634, "APDClass in"=w2637) -> ("Error Out"=w2633:errorcluster)  [unwired: 7 in, 1 out]
          }
          frame "Ch2" {
            n1175 = Unbundle By Name(w2645) -> ("Ch2APDSerial#"=w2644:string)
            n1176 = call "CreatFromSerialNum.vi"("error in (no error)"=w2643, "APD Serial #"=w2644) -> ("error out"=w2642:errorcluster, "APDClass out"=w2646:refnum<class "APDClass.lvclass">)  [unwired: 8 in]
            n1177 = call "APD2FGV.vi"("Error In"=w2642, "Operation (Read)"=w2640, "APDClass in"=w2646) -> ("Error Out"=w2641:errorcluster)  [unwired: 7 in, 1 out]
          }
          frame "Ch3" {
            n1178 = Unbundle By Name(w2651) -> ("Ch3APDSerial#"=w2650:string)
            n1179 = call "CreatFromSerialNum.vi"("error in (no error)"=w2649, "APD Serial #"=w2650) -> ("error out"=w2652:errorcluster, "APDClass out"=w2653:refnum<class "APDClass.lvclass">)  [unwired: 8 in]
            n1180 = call "APD3FGV.vi"("Error In"=w2652, "Operation (Read)"=w2648, "APDClass in"=w2653) -> ("Error Out"=w2647:errorcluster)  [unwired: 7 in, 1 out]
          }
          frame "Ch4" {
            n1181 = Unbundle By Name(w2658) -> ("Ch4APDSerial#"=w2657:string)
            n1182 = call "CreatFromSerialNum.vi"("error in (no error)"=w2656, "APD Serial #"=w2657) -> ("error out"=w2660:errorcluster, "APDClass out"=w2659:refnum<class "APDClass.lvclass">)  [unwired: 8 in]
            n1183 = call "APD4FGV.vi"("Error In"=w2660, "Operation (Read)"=w2654, "APDClass in"=w2659) -> ("Error Out"=w2655:errorcluster)  [unwired: 7 in, 1 out]
          }
        }
        n1184 = Bundle By Name(cluster=w2628, "APDSerials"=w2625) -> (w2629:T22)
        n1185 = call <vilib>:"Add State(s) to Queue__JKI_lib_State_Machine.vi"("State(s) in (\"\")"=w2632) -> ("States Out"=w2631:string)  [unwired: 14 in]
      }
      frame "APD: LoadFromSerialNoRawData" {
        w2664 = enum16{"Read", "Write"}."Write" ("Operation (Read)")
        # "Load APD info based on serial numbers\n(update FGV)"
        n1186 = call "readAPDSerial.vi"("Error In"=w2668) -> ("Error Out"=w2666:errorcluster, "output cluster"=w2669:T39)  [unwired: 9 in]
        n1187 = Unbundle By Name(w2669) -> ("Ch1APDSerial#"=w2680:string, "Ch2APDSerial#"=w2678:string, "Ch3APDSerial#"=w2667:string, "Ch4APDSerial#"=w2661:string)
        n1188 = call "CreatFromSerialNumNoRaw.vi"("error in (no error)"=w2666, "APD Serial #"=w2680) -> ("error out"=w2670:errorcluster, "APDClass out"=w2679:refnum<class "APDClass.lvclass">)  [unwired: 8 in]
        n1189 = call "CreatFromSerialNumNoRaw.vi"("error in (no error)"=w2666, "APD Serial #"=w2678) -> ("error out"=w2677:errorcluster, "APDClass out"=w2674:refnum<class "APDClass.lvclass">)  [unwired: 8 in]
        n1190 = call "CreatFromSerialNumNoRaw.vi"("error in (no error)"=w2666, "APD Serial #"=w2667) -> ("error out"=w2676:errorcluster, "APDClass out"=w2675:refnum<class "APDClass.lvclass">)  [unwired: 8 in]
        n1191 = call "CreatFromSerialNumNoRaw.vi"("error in (no error)"=w2666, "APD Serial #"=w2661) -> ("error out"=w2663:errorcluster, "APDClass out"=w2665:refnum<class "APDClass.lvclass">)  [unwired: 8 in]
        n1192 = call "APD1FGV.vi"("Error In"=w2670, "Operation (Read)"=w2664, "APDClass in"=w2679) -> ("Error Out"=w2681:errorcluster)  [unwired: 7 in, 1 out]
        n1193 = call "APD2FGV.vi"("Error In"=w2677, "Operation (Read)"=w2664, "APDClass in"=w2674) -> ("Error Out"=w2682:errorcluster)  [unwired: 7 in, 1 out]
        n1194 = call "APD3FGV.vi"("Error In"=w2676, "Operation (Read)"=w2664, "APDClass in"=w2675) -> ("Error Out"=w2683:errorcluster)  [unwired: 7 in, 1 out]
        n1195 = call "APD4FGV.vi"("Error In"=w2663, "Operation (Read)"=w2664, "APDClass in"=w2665) -> ("Error Out"=w2662:errorcluster)  [unwired: 7 in, 1 out]
        n1196 = Merge Errors(w2681, w2682, w2683, w2662) -> (w2671:errorcluster)
        n1197 = Bundle By Name(cluster=w2672, "APDSerials"=w2669) -> (w2673:T22)
        n1198 = call <vilib>:"Add State(s) to Queue__JKI_lib_State_Machine.vi"("State(s) in (\"\")"=w2686) -> ("States Out"=w2685:string)  [unwired: 14 in]
      }
      frame "APD: GetGainLimits" {
        w2691 = enum16{"Read", "Write"}."Read" ("Operation (Read)")
        # "Template Separator\n(You can make a copy of, or modify, this frame)"
        n1199 = call "APD1FGV.vi"("Error In"=w2690, "Operation (Read)"=w2691) -> ("Error Out"=w2703:errorcluster, "APDClass out"=w2704:refnum<class "APDClass.lvclass">)  [unwired: 8 in]
        n1200 = call "APD2FGV.vi"("Error In"=w2690, "Operation (Read)"=w2691) -> ("Error Out"=w2700:errorcluster, "APDClass out"=w2701:refnum<class "APDClass.lvclass">)  [unwired: 8 in]
        n1201 = call "APD3FGV.vi"("Error In"=w2690, "Operation (Read)"=w2691) -> ("Error Out"=w2698:errorcluster, "APDClass out"=w2699:refnum<class "APDClass.lvclass">)  [unwired: 8 in]
        n1202 = call "APD4FGV.vi"("Error In"=w2690, "Operation (Read)"=w2691) -> ("Error Out"=w2689:errorcluster, "APDClass out"=w2688:refnum<class "APDClass.lvclass">)  [unwired: 8 in]
        n1203 = call-dynamic "Read Gain Limits(Log).vi"("error in (no error)"=w2689, "APDClass in"=w2688) -> ("GainLimits(Log)"=w2687:cluster{"GainMax":dbl, "GainMin":dbl})  [unwired: 7 in, 2 out]
        n1204 = call-dynamic "Read Gain Limits(Log).vi"("error in (no error)"=w2703, "APDClass in"=w2704) -> ("error out"=w2695:errorcluster, "GainLimits(Log)"=w2702:cluster{"GainMax":dbl, "GainMin":dbl})  [unwired: 7 in, 1 out]
        n1205 = call-dynamic "Read Gain Limits(Log).vi"("error in (no error)"=w2700, "APDClass in"=w2701) -> ("error out"=w2694:errorcluster, "GainLimits(Log)"=w2697:cluster{"GainMax":dbl, "GainMin":dbl})  [unwired: 7 in, 1 out]
        n1206 = call-dynamic "Read Gain Limits(Log).vi"("error in (no error)"=w2698, "APDClass in"=w2699) -> ("error out"=w2693:errorcluster, "GainLimits(Log)"=w2696:cluster{"GainMax":dbl, "GainMin":dbl})  [unwired: 7 in, 1 out]
        n1207 = global write "GlobalVariables.vi" "Ch1GainLim(Log)"(w2702) -> ()
        n1208 = global write "GlobalVariables.vi" "Ch2GainLim(Log)"(w2697) -> ()
        n1209 = global write "GlobalVariables.vi" "Ch3GainLim(Log)"(w2696) -> ()
        n1210 = global write "GlobalVariables.vi" "Ch4GainLim(Log)"(w2687) -> ()
        n1211 = Merge Errors(w2695, w2694, w2693) -> (w2692:errorcluster)
        n1212 = call <vilib>:"Add State(s) to Queue__JKI_lib_State_Machine.vi"("State(s) in (\"\")"=w2708) -> ("States Out"=w2707:string)  [unwired: 14 in]
      }
      frame "APD: UpdateIndicatorMacro" {
        # "update indicator for all channel\n(You can make a copy of, or modify, this frame)"
        n1213 = call <vilib>:"Add State(s) to Queue__JKI_lib_State_Machine.vi"("State(s) in Front (\"\")"="APD: UpdateIndicatorCh1\nAPD: UpdateIndicatorCh2\nAPD: UpdateIndicatorCh3\nAPD: UpdateIndicatorCh4" ("State(s) in Front (\"\")"), "State(s) in (\"\")"=w2714) -> ("States Out"=w2713:string)  [unwired: 13 in]
      }
      frame "APD: UpdateIndicatorCh1" {
        # "Update APD module front panel indicators\n(Read data, update FGV, update plot)"
        n1214 = call "APD1FGV.vi"("Error In"=w2715) -> ("Error Out"=w2734:errorcluster, "APDClass out"=w2735:refnum<class "APDClass.lvclass">)  [unwired: 9 in]
        n1215 = call-dynamic "Read APD Serial.vi"("error in (no error)"=w2734, "APDClass in"=w2735) -> ("error out"=w2722:errorcluster, "APD Serial #"=w2731:string, "APDClass out"=w2724:refnum<class "APDClass.lvclass">)  [unwired: 7 in]
        n1216 = call-dynamic "Read DateTime.vi"("error in (no error)"=w2722, "APDClass in"=w2724) -> ("error out"=w2721:errorcluster, "DateTime"=→"DateTimeCh1":string, "APDClass out"=w2723:refnum<class "APDClass.lvclass">)  [unwired: 7 in]
        n1217 = local write "Serial Number Ch1"(w2731) -> ()
        n1218 = call-dynamic "Read GainData.vi"("error in (no error)"=w2721, "APDClass in"=w2723) -> ("error out"=w2732:errorcluster, "GainData"=w2725:T40, "APDClass out"=w2733:refnum<class "APDClass.lvclass">)  [unwired: 7 in]
        n1219 = Unbundle By Name(w2725) -> ("CtrlV"=w2720:dbl[], "Gain"=w2719:dbl[])
        n1220 = call-dynamic "Read iRFData.vi"("error in (no error)"=w2732, "APDClass in"=w2733) -> ("error out"=w2727:errorcluster, "iRFData"=w2730:T41)  [unwired: 7 in, 1 out]
        n1221 = Array Max & Min(array=w2720) -> (max value=→"Ch1 Max CtrlV":dbl)  [unwired: 3 out]
        n1222 = Bundle("CtrlV"=w2720, "Gain"=w2719) -> (→"Ch1 Gain":cluster{"CtrlV":dbl[], "Gain":dbl[]})  [unwired: 1 in]
        n1223 = Unbundle By Name(w2730) -> ("iRFWFsAvg"=→"Ch1 iRF Graph":dbl[][], "dt"=w2728:dbl)
        n1224 = property on="Ch1 iRF Graph" class="WFGraph (strict)"(error in=w2727, "XScale.Multiplier"=w2728) -> (error out=w2726:errorcluster)  [unwired: 1 in, 1 out]
        n1225 = call <vilib>:"Add State(s) to Queue__JKI_lib_State_Machine.vi"("State(s) in (\"\")"=w2739) -> ("States Out"=w2738:string)  [unwired: 14 in]
      }
      frame "APD: UpdateIndicatorCh2" {
        # "Update Channel 2 indicators\n(You can make a copy of, or modify, this frame)"
        n1226 = call "APD2FGV.vi"("Error In"=w2741) -> ("Error Out"=w2757:errorcluster, "APDClass out"=w2758:refnum<class "APDClass.lvclass">)  [unwired: 9 in]
        n1227 = call-dynamic "Read APD Serial.vi"("error in (no error)"=w2757, "APDClass in"=w2758) -> ("error out"=w2747:errorcluster, "APD Serial #"=w2756:string, "APDClass out"=w2749:refnum<class "APDClass.lvclass">)  [unwired: 7 in]
        n1228 = call-dynamic "Read DateTime.vi"("error in (no error)"=w2747, "APDClass in"=w2749) -> ("error out"=w2746:errorcluster, "DateTime"=→"DateTimeCh2":string, "APDClass out"=w2748:refnum<class "APDClass.lvclass">)  [unwired: 7 in]
        n1229 = local write "Serial Number Ch2"(w2756) -> ()
        n1230 = call-dynamic "Read GainData.vi"("error in (no error)"=w2746, "APDClass in"=w2748) -> ("error out"=w2759:errorcluster, "GainData"=w2751:T40, "APDClass out"=w2760:refnum<class "APDClass.lvclass">)  [unwired: 7 in]
        n1231 = Unbundle By Name(w2751) -> ("CtrlV"=w2744:dbl[], "Gain"=w2743:dbl[])
        n1232 = call-dynamic "Read iRFData.vi"("error in (no error)"=w2759, "APDClass in"=w2760) -> ("error out"=w2752:errorcluster, "iRFData"=w2755:T41)  [unwired: 7 in, 1 out]
        n1233 = Array Max & Min(array=w2744) -> (max value=→"Ch2 Max CtrlV":dbl)  [unwired: 3 out]
        n1234 = Bundle("CtrlV"=w2744, "Gain"=w2743) -> (→"Ch2 Gain":cluster{"CtrlV":dbl[], "Gain":dbl[]})  [unwired: 1 in]
        n1235 = Unbundle By Name(w2755) -> ("iRFWFsAvg"=→"Ch2 iRF Graph":dbl[][], "dt"=w2753:dbl)
        n1236 = property on="Ch2 iRF Graph" class="WFGraph (strict)"(error in=w2752, "XScale.Multiplier"=w2753) -> (error out=w2740:errorcluster)  [unwired: 1 in, 1 out]
        n1237 = call <vilib>:"Add State(s) to Queue__JKI_lib_State_Machine.vi"("State(s) in (\"\")"=w2764) -> ("States Out"=w2763:string)  [unwired: 14 in]
      }
      frame "APD: UpdateIndicatorCh3" {
        # "update ch3 indicator\n(You can make a copy of, or modify, this frame)"
        n1238 = call "APD3FGV.vi"("Error In"=w2765) -> ("Error Out"=w2783:errorcluster, "APDClass out"=w2784:refnum<class "APDClass.lvclass">)  [unwired: 9 in]
        n1239 = call-dynamic "Read APD Serial.vi"("error in (no error)"=w2783, "APDClass in"=w2784) -> ("error out"=w2775:errorcluster, "APD Serial #"=w2777:string, "APDClass out"=w2776:refnum<class "APDClass.lvclass">)  [unwired: 7 in]
        n1240 = call-dynamic "Read DateTime.vi"("error in (no error)"=w2775, "APDClass in"=w2776) -> ("error out"=w2773:errorcluster, "DateTime"=→"DateTimeCh3":string, "APDClass out"=w2774:refnum<class "APDClass.lvclass">)  [unwired: 7 in]
        n1241 = local write "Serial Number Ch3"(w2777) -> ()
        n1242 = call-dynamic "Read GainData.vi"("error in (no error)"=w2773, "APDClass in"=w2774) -> ("error out"=w2782:errorcluster, "GainData"=w2772:T40, "APDClass out"=w2785:refnum<class "APDClass.lvclass">)  [unwired: 7 in]
        n1243 = Unbundle By Name(w2772) -> ("CtrlV"=w2771:dbl[], "Gain"=w2770:dbl[])
        n1244 = call-dynamic "Read iRFData.vi"("error in (no error)"=w2782, "APDClass in"=w2785) -> ("error out"=w2781:errorcluster, "iRFData"=w2778:T41)  [unwired: 7 in, 1 out]
        n1245 = Array Max & Min(array=w2771) -> (max value=→"Ch3 Max CtrlV":dbl)  [unwired: 3 out]
        n1246 = Bundle("CtrlV"=w2771, "Gain"=w2770) -> (→"Ch3 Gain":cluster{"CtrlV":dbl[], "Gain":dbl[]})  [unwired: 1 in]
        n1247 = Unbundle By Name(w2778) -> ("iRFWFsAvg"=→"Ch3 iRF Graph":dbl[][], "dt"=w2780:dbl)
        n1248 = property on="Ch3 iRF Graph" class="WFGraph (strict)"(error in=w2781, "XScale.Multiplier"=w2780) -> (error out=w2766:errorcluster)  [unwired: 1 in, 1 out]
        n1249 = call <vilib>:"Add State(s) to Queue__JKI_lib_State_Machine.vi"("State(s) in (\"\")"=w2789) -> ("States Out"=w2788:string)  [unwired: 14 in]
      }
      frame "APD: UpdateIndicatorCh4" {
        # "update ch4 indicators\n(You can make a copy of, or modify, this frame)"
        n1250 = call "APD4FGV.vi"("Error In"=w2806) -> ("Error Out"=w2810:errorcluster, "APDClass out"=w2805:refnum<class "APDClass.lvclass">)  [unwired: 9 in]
        n1251 = call-dynamic "Read APD Serial.vi"("error in (no error)"=w2810, "APDClass in"=w2805) -> ("error out"=w2809:errorcluster, "APD Serial #"=→"Serial Number Ch4":string, "APDClass out"=w2804:refnum<class "APDClass.lvclass">)  [unwired: 7 in]
        n1252 = call-dynamic "Read DateTime.vi"("error in (no error)"=w2809, "APDClass in"=w2804) -> ("error out"=w2808:errorcluster, "DateTime"=→"DateTimeCh4":string, "APDClass out"=w2803:refnum<class "APDClass.lvclass">)  [unwired: 7 in]
        n1253 = call-dynamic "Read GainData.vi"("error in (no error)"=w2808, "APDClass in"=w2803) -> ("error out"=w2807:errorcluster, "GainData"=w2799:T40, "APDClass out"=w2802:refnum<class "APDClass.lvclass">)  [unwired: 7 in]
        n1254 = Unbundle By Name(w2799) -> ("CtrlV"=w2797:dbl[], "Gain"=w2796:dbl[])
        n1255 = call-dynamic "Read iRFData.vi"("error in (no error)"=w2807, "APDClass in"=w2802) -> ("error out"=w2791:errorcluster, "iRFData"=w2794:T41)  [unwired: 7 in, 1 out]
        n1256 = Array Max & Min(array=w2797) -> (max value=→"Ch4 Max CtrlV":dbl)  [unwired: 3 out]
        n1257 = Bundle("CtrlV"=w2797, "Gain"=w2796) -> (→"Ch4 Gain":cluster{"CtrlV":dbl[], "Gain":dbl[]})  [unwired: 1 in]
        n1258 = Unbundle By Name(w2794) -> ("iRFWFsAvg"=→"Ch4 iRF Graph":dbl[][], "dt"=w2792:dbl)
        n1259 = property on="Ch4 iRF Graph" class="WFGraph (strict)"(error in=w2791, "XScale.Multiplier"=w2792) -> (error out=w2790:errorcluster)  [unwired: 1 in, 1 out]
        n1260 = call <vilib>:"Add State(s) to Queue__JKI_lib_State_Machine.vi"("State(s) in (\"\")"=w2814) -> ("States Out"=w2813:string)  [unwired: 14 in]
      }
      frame "APD: writeGain" {
        w2815 = T40 {"CtrlV"=[], "NumOfWFs"=0, "WF length"=0, "Gain"=[], "GainRaw"=[], "GainBGRaw"=[]}  # GainData
        # "Parse all data for all gain\n(parse data all gain)"
        n1261 = Flush Queue(queue=w2827, error in (no error)=w2828) -> (remaining elements=w2824:cluster{"CtrlV":dbl, "WFs":dbl[][]}[], error out=w2822:errorcluster)  [unwired: 1 out]
        n1262 = for {
          tunnel: w2824 -> [w2871] mode=indexing
          tunnel: [w2870] -> w2821 mode=indexing
          tunnel: [w2867] -> w2817
          tunnel: [w2864] -> w2816
          # "Reshape gain WF array to vectors"
          n1263 = Unbundle By Name(w2871) -> ("WFs"=w2869:dbl[][])
          n1264 = Array Size(array=w2869) -> (size(s)=w2868:i32[])
          n1265 = for {
            tunnel: w2869 -> [w2872] mode=indexing
            tunnel: [w2872] -> w2870 mode=concatenating
          }
          n1266 = Index Array(array=w2868, index #1=0 ("index"), index #2=1 ("index")) -> (element #1=w2864:i32, element #2=w2867:i32)
        }
        n1267 = local read "Ctrl V"() -> (w2819:dbl[])
        n1268 = local read "Gain"() -> (w2818:dbl[])
        n1269 = Bundle By Name(cluster=w2815, "CtrlV"=w2819, "Gain"=w2818, "WF length"=w2817, "NumOfWFs"=w2816, "GainRaw"=w2821) -> (w2820:T40)
        n1270 = local read "Channel"() -> (w2823:enum32{"Ch1", "Ch2", "Ch3", "Ch4"})
        n1271 = case shown="\"Ch2\"" w2823 {
          tunnel: [w2833 w2840 w2848 w2856] -> w2826
          tunnel: w2822 -> [w2839 w2847 w2855 w2863]
          tunnel: w2820 -> [w2837 w2844 w2852 w2860]
          frame "Ch1", Default {
            n1272 = call "APD1FGV.vi"("Error In"=w2839) -> ("Error Out"=w2838:errorcluster, "APDClass out"=w2836:refnum<class "APDClass.lvclass">)  [unwired: 9 in]
            n1273 = call-dynamic "Write GainData.vi"("error in (no error)"=w2838, "GainData"=w2837, "APDClass in"=w2836) -> ("error out"=w2834:errorcluster, "APDClass out"=w2835:refnum<class "APDClass.lvclass">)  [unwired: 7 in]
            n1274 = call "APD1FGV.vi"("Error In"=w2834, "Operation (Read)"=enum16{"Read", "Write"}."Write", "APDClass in"=w2835) -> ("Error Out"=w2833:errorcluster)  [unwired: 7 in, 1 out]
          }
          frame "Ch2" {
            n1275 = call "APD2FGV.vi"("Error In"=w2847) -> ("Error Out"=w2845:errorcluster, "APDClass out"=w2846:refnum<class "APDClass.lvclass">)  [unwired: 9 in]
            n1276 = call-dynamic "Write GainData.vi"("error in (no error)"=w2845, "GainData"=w2844, "APDClass in"=w2846) -> ("error out"=w2841:errorcluster, "APDClass out"=w2843:refnum<class "APDClass.lvclass">)  [unwired: 7 in]
            n1277 = call "APD2FGV.vi"("Error In"=w2841, "Operation (Read)"=enum16{"Read", "Write"}."Write", "APDClass in"=w2843) -> ("Error Out"=w2840:errorcluster)  [unwired: 7 in, 1 out]
          }
          frame "Ch3" {
            n1278 = call "APD3FGV.vi"("Error In"=w2855) -> ("Error Out"=w2853:errorcluster, "APDClass out"=w2854:refnum<class "APDClass.lvclass">)  [unwired: 9 in]
            n1279 = call-dynamic "Write GainData.vi"("error in (no error)"=w2853, "GainData"=w2852, "APDClass in"=w2854) -> ("error out"=w2849:errorcluster, "APDClass out"=w2851:refnum<class "APDClass.lvclass">)  [unwired: 7 in]
            n1280 = call "APD3FGV.vi"("Error In"=w2849, "Operation (Read)"=enum16{"Read", "Write"}."Write", "APDClass in"=w2851) -> ("Error Out"=w2848:errorcluster)  [unwired: 7 in, 1 out]
          }
          frame "Ch4" {
            n1281 = call "APD4FGV.vi"("Error In"=w2863) -> ("Error Out"=w2861:errorcluster, "APDClass out"=w2862:refnum<class "APDClass.lvclass">)  [unwired: 9 in]
            n1282 = call-dynamic "Write GainData.vi"("error in (no error)"=w2861, "GainData"=w2860, "APDClass in"=w2862) -> ("error out"=w2857:errorcluster, "APDClass out"=w2859:refnum<class "APDClass.lvclass">)  [unwired: 7 in]
            n1283 = call "APD4FGV.vi"("Error In"=w2857, "Operation (Read)"=enum16{"Read", "Write"}."Write", "APDClass in"=w2859) -> ("Error Out"=w2856:errorcluster)  [unwired: 7 in, 1 out]
          }
        }
        n1284 = call <vilib>:"Add State(s) to Queue__JKI_lib_State_Machine.vi"("State(s) in (\"\")"=w2831) -> ("States Out"=w2830:string)  [unwired: 14 in]
      }
      frame "APD: writeiRF" {
        w2882 = T41 {"dt"=0.0, "NumOfWFs"=0, "WFLength"=0, "iRFCtrlV"=[], "iRFWFsAvg"=[], "iRFRaw"=[]}  # iRF
        # "Parse all data for all gain\n(parse data all gain)"
        n1285 = Flush Queue(queue=w2891, error in (no error)=w2889) -> (remaining elements=w2887:T42, error out=w2884:errorcluster)  [unwired: 1 out]
        n1286 = for {
          tunnel: w2887 -> [w2939] mode=indexing
          tunnel: [w2937] -> w2880 mode=indexing
          tunnel: [w2938] -> w2879 mode=indexing
          tunnel: [w2936] -> w2881 mode=indexing
          shift-right: [w2932] -> w2878
          shift-left: i32[] [] -> [w2931]
          i -> [w2935]
          n1287 = Equal To 0?(x=w2935) -> (x = 0?=w2934:bool)
          n1288 = Unbundle By Name(w2939) -> ("CtrlV"=w2937:dbl, "WFavg"=w2938:dbl[], "WFs"=w2933:dbl[][])
          n1289 = case shown="True" w2934 {
            tunnel: w2933 -> [_ w2942]
            tunnel: [w2940 w2941] -> w2932
            tunnel: w2931 -> [w2940 _]
            frame False {
            }
            frame True {
              n1290 = Array Size(array=w2942) -> (size(s)=w2941:i32[])
            }
          }
          n1291 = for {
            tunnel: w2933 -> [w2943] mode=indexing
            tunnel: [w2943] -> w2936 mode=concatenating
          }
        }
        n1292 = Index Array(array=w2878, index #1=0 ("index (row)"), index #2=1 ("disabled index (col)")) -> (element #1=w2874:i32, element #2=w2873:i32)
        n1293 = Bundle By Name(cluster=w2882, "dt"=0.2, "NumOfWFs"=w2874, "WFLength"=w2873, "iRFCtrlV"=w2880, "iRFWFsAvg"=w2879, "iRFRaw"=w2881) -> (w2883:T41)
        n1294 = local read "Channel"() -> (w2885:enum32{"Ch1", "Ch2", "Ch3", "Ch4"})
        n1295 = case shown="\"Ch4\"" w2885 {
          tunnel: w2884 -> [w2903 w2911 w2920 w2929]
          tunnel: w2879 -> [w2902 w2912 w2921 w2930]
          tunnel: w2883 -> [w2900 w2908 w2915 w2924]
          tunnel: [w2895 w2904 w2913 w2922] -> w2890
          frame "Ch1", Default {
            n1296 = local write "Ch1 iRF Graph"(w2902) -> ()
            n1297 = call "APD1FGV.vi"("Error In"=w2903) -> ("Error Out"=w2901:errorcluster, "APDClass out"=w2899:refnum<class "APDClass.lvclass">)  [unwired: 9 in]
            n1298 = call-dynamic "Write iRFData.vi"("error in (no error)"=w2901, "iRFData"=w2900, "APDClass in"=w2899) -> ("error out"=w2898:errorcluster, "APDClass out"=w2897:refnum<class "APDClass.lvclass">)  [unwired: 7 in]
            n1299 = call "APD1FGV.vi"("Error In"=w2898, "Operation (Read)"=enum16{"Read", "Write"}."Write", "APDClass in"=w2897) -> ("Error Out"=w2895:errorcluster)  [unwired: 7 in, 1 out]
          }
          frame "Ch2" {
            n1300 = local write "Ch2 iRF Graph"(w2912) -> ()
            n1301 = call "APD2FGV.vi"("Error In"=w2911) -> ("Error Out"=w2910:errorcluster, "APDClass out"=w2909:refnum<class "APDClass.lvclass">)  [unwired: 9 in]
            n1302 = call-dynamic "Write iRFData.vi"("error in (no error)"=w2910, "iRFData"=w2908, "APDClass in"=w2909) -> ("error out"=w2906:errorcluster, "APDClass out"=w2907:refnum<class "APDClass.lvclass">)  [unwired: 7 in]
            n1303 = call "APD2FGV.vi"("Error In"=w2906, "Operation (Read)"=enum16{"Read", "Write"}."Write", "APDClass in"=w2907) -> ("Error Out"=w2904:errorcluster)  [unwired: 7 in, 1 out]
          }
          frame "Ch3" {
            n1304 = local write "Ch3 iRF Graph"(w2921) -> ()
            n1305 = call "APD3FGV.vi"("Error In"=w2920) -> ("Error Out"=w2919:errorcluster, "APDClass out"=w2917:refnum<class "APDClass.lvclass">)  [unwired: 9 in]
            n1306 = call-dynamic "Write iRFData.vi"("error in (no error)"=w2919, "iRFData"=w2915, "APDClass in"=w2917) -> ("error out"=w2918:errorcluster, "APDClass out"=w2916:refnum<class "APDClass.lvclass">)  [unwired: 7 in]
            n1307 = call "APD3FGV.vi"("Error In"=w2918, "Operation (Read)"=enum16{"Read", "Write"}."Write", "APDClass in"=w2916) -> ("Error Out"=w2913:errorcluster)  [unwired: 7 in, 1 out]
          }
          frame "Ch4" {
            n1308 = local write "Ch4 iRF Graph"(w2930) -> ()
            n1309 = call "APD4FGV.vi"("Error In"=w2929) -> ("Error Out"=w2928:errorcluster, "APDClass out"=w2926:refnum<class "APDClass.lvclass">)  [unwired: 9 in]
            n1310 = call-dynamic "Write iRFData.vi"("error in (no error)"=w2928, "iRFData"=w2924, "APDClass in"=w2926) -> ("error out"=w2927:errorcluster, "APDClass out"=w2925:refnum<class "APDClass.lvclass">)  [unwired: 7 in]
            n1311 = call "APD4FGV.vi"("Error In"=w2927, "Operation (Read)"=enum16{"Read", "Write"}."Write", "APDClass in"=w2925) -> ("Error Out"=w2922:errorcluster)  [unwired: 7 in, 1 out]
          }
        }
        n1312 = call <vilib>:"Add State(s) to Queue__JKI_lib_State_Machine.vi"("State(s) in (\"\")"=w2894) -> ("States Out"=w2893:string)  [unwired: 14 in]
      }
      frame "APD: SaveNew" {
        # "Save APD info\n(You can make a copy of, or modify, this frame)"
        n1313 = local read "Channel"() -> (w2948:enum32{"Ch1", "Ch2", "Ch3", "Ch4"})
        n1314 = case shown="\"Ch1\", Default" w2948 {
          tunnel: [w2957 w2960 w2963 w2966] -> w2947
          tunnel: w2946 -> [w2956 w2958 w2961 w2964]
          tunnel: [w2955 w2959 w2962 w2965] -> w2945
          frame "Ch1", Default {
            n1315 = call "APD1FGV.vi"("Error In"=w2956) -> ("Error Out"=w2955:errorcluster, "APDClass out"=w2957:refnum<class "APDClass.lvclass">)  [unwired: 9 in]
          }
          frame "Ch2" {
            n1316 = call "APD2FGV.vi"("Error In"=w2958) -> ("Error Out"=w2959:errorcluster, "APDClass out"=w2960:refnum<class "APDClass.lvclass">)  [unwired: 9 in]
          }
          frame "Ch3" {
            n1317 = call "APD3FGV.vi"("Error In"=w2961) -> ("Error Out"=w2962:errorcluster, "APDClass out"=w2963:refnum<class "APDClass.lvclass">)  [unwired: 9 in]
          }
          frame "Ch4" {
            n1318 = call "APD4FGV.vi"("Error In"=w2964) -> ("Error Out"=w2965:errorcluster, "APDClass out"=w2966:refnum<class "APDClass.lvclass">)  [unwired: 9 in]
          }
        }
        n1319 = call "Write to File.vi"("Error In"=w2945, "APDClass.lvclass"=w2947) -> ("Error Out"=w2944:errorcluster)  [unwired: 9 in]
        n1320 = case shown="Error .." w2944 {
          frame No Error {
            n1321 = One Button Dialog(message="Data saved successfully!") -> ()  [unwired: 1 in, 1 out]
          }
          frame Error {
            n1322 = One Button Dialog(message="Error saving to APD file!") -> ()  [unwired: 1 in, 1 out]
          }
        }
        n1323 = call <vilib>:"Add State(s) to Queue__JKI_lib_State_Machine.vi"("State(s) in (\"\")"=w2952) -> ("States Out"=w2951:string)  [unwired: 14 in]
      }
      frame "---------- Aquisition ----------" {
        # "Template Separator\n(You can make a copy of, or modify, this frame)"
        n1324 = call <vilib>:"Add State(s) to Queue__JKI_lib_State_Machine.vi"("State(s) in (\"\")"=w2971) -> ("States Out"=w2970:string)  [unwired: 14 in]
      }
      frame "Aquisition: EnqueueV" {
        # "Enqueue aquisition V\n(You can make a copy of, or modify, this frame)"
        n1325 = while {
          tunnel: w2976 -> [w2994]
          shift-right: [w2992] -> w2975
          shift-left: w2974 -> [w2993]
          shift-right: [w2986] -> _
          shift-left: "Gain low" -> [w2990]
          tunnel: "Step" -> [w2987]
          tunnel: "Gain High" -> [w2988]
          tunnel: "Gain low" -> [w2991]
          stop <- w2985 stop-if-true
          # "check gain value, stop if out of range"
          n1326 = Add(x=w2988, y=w2987) -> (x+y=w2984:dbl)
          n1327 = In Range and Coerce(upper limit=w2988, x=w2990, lower limit=w2991) -> (coerced(x)=w2989:dbl)  [unwired: 1 out]
          n1328 = Enqueue Element(queue=w2994, element=w2989, error in (no error)=w2993) -> (error out=w2992:errorcluster)  [unwired: 1 in, 2 out]
          n1329 = Subtract(x=w2984, y=0.0001) -> (x-y=w2982:dbl)
          n1330 = Add(x=w2990, y=w2987) -> (x+y=w2986:dbl)
          n1331 = Greater Or Equal?(x=w2986, y=w2982) -> (x >= y?=w2985:bool)
        }
        n1332 = call <vilib>:"Add State(s) to Queue__JKI_lib_State_Machine.vi"("State(s) in (\"\")"=w2981) -> ("States Out"=w2980:string)  [unwired: 14 in]
      }
      frame "Aquisition: RecordData" {
        # "Set gain\nstart aquisition\nask user to adjust signal level\nstop aquisition\nstart aquisition"
        # "Template Separator\n(You can make a copy of, or modify, this frame)"
        n1333 = Fract/Exp String To Number(string=w2995) -> (number=w3000:dbl)  [unwired: 3 in, 1 out]
        n1334 = call "V1FGV.vi"("Error In"=w2999, "action (write)"=enum16{"write", "read"}."write" ("action"), "V1 in"=w3000) -> ("Error Out"=w2998:errorcluster)  [unwired: 7 in, 1 out]
        n1335 = call <vilib>:"Add State(s) to Queue__JKI_lib_State_Machine.vi"("State(s) in Front (\"\")"="Queue: Flash\nUtility: setSaveFlag >> 0\nMacro: StartRun\nUI: ShowDialog\nUtility: setSaveFlag >> 1\nQueue: CheckNumOfWF\nMacro: StopRun\n" ("State(s) in Front (\"\")"), "State(s) in (\"\")"=w3004) -> ("States Out"=w3003:string)  [unwired: 13 in]
      }
      frame "---------- File ----------" {
        # "Template Separator\n(You can make a copy of, or modify, this frame)"
        n1336 = call <vilib>:"Add State(s) to Queue__JKI_lib_State_Machine.vi"("State(s) in (\"\")"=w3009) -> ("States Out"=w3008:string)  [unwired: 14 in]
      }
      frame "File: BackupOld" {
        w3017 = ".tdms" ("string")
        # ".tdms_index file is not required for storage or distribution and automatically regenerates\nno need to copy the index file"
        # "Backup old APD data file\n()"
        n1337 = local read "Channel"() -> (w3027:enum32{"Ch1", "Ch2", "Ch3", "Ch4"})
        n1338 = case shown="\"Ch1\", Default" w3027 {
          tunnel: [w3032 w3033 w3034 w3035] -> w3018
          frame "Ch1", Default {
            n1339 = local read "Serial Number Ch1"() -> (w3032:string)
          }
          frame "Ch2" {
            n1340 = local read "Serial Number Ch2"() -> (w3033:string)
          }
          frame "Ch3" {
            n1341 = local read "Serial Number Ch3"() -> (w3034:string)
          }
          frame "Ch4" {
            n1342 = local read "Serial Number Ch4"() -> (w3035:string)
          }
        }
        n1343 = call <vilib>:"Application Directory.vi"() -> ("Application Directory"=w3028:path)
        n1344 = Get Date/Time In Seconds() -> (seconds since 1Jan1904=w3022:timestamp)
        n1345 = Format Date/Time String(time format string (%c)="%m-%d-%Y %H-%M", seconds (now)=w3022) -> (date/time string=w3021:string)  [unwired: 1 in]
        n1346 = Build Path(base path=w3028, name or relative path="ConfigFiles") -> (appended path=w3025:path)
        n1347 = Build Path(base path=w3025, name or relative path="Backup") -> (appended path=w3024:path)
        n1348 = Concatenate Strings(w3018, w3017) -> (w3019:string)
        n1349 = Concatenate Strings(w3018, " BK " ("string"), w3021, w3017) -> (w3020:string)
        n1350 = Build Path(base path=w3025, name or relative path=w3019) -> (appended path=w3026:path)
        n1351 = Build Path(base path=w3024, name or relative path=w3020) -> (appended path=w3023:path)
        n1352 = Copy(8:w3012, 10:w3023, 11:w3026) -> (0:w3011:errorcluster)  [unwired: 2 in, 2 out]
        n1353 = call <vilib>:"Add State(s) to Queue__JKI_lib_State_Machine.vi"("State(s) in (\"\")"=w3031) -> ("States Out"=w3030:string)  [unwired: 14 in]
      }
      frame "---------- PID ----------" {
        # "Template Separator\n(You can make a copy of, or modify, this frame)"
        n1354 = call <vilib>:"Add State(s) to Queue__JKI_lib_State_Machine.vi"("State(s) in (\"\")"=w3040) -> ("States Out"=w3039:string)  [unwired: 14 in]
      }
      frame "PID: loadPID" {
        # "Template Separator\n(You can make a copy of, or modify, this frame)"
        n1355 = call "readPIDSetting.vi"("Error In"=w3044) -> ("Error Out"=w3045:errorcluster, "Ch3 PID out"=w3041:T6, "Ch2 PID out"=w3042:T6, "Ch1 PID out"=w3043:T6)  [unwired: 7 in]
        n1356 = local write "Ch1 PID gains"(w3043) -> ()
        n1357 = local write "Ch2 PID gains"(w3042) -> ()
        n1358 = local write "Ch3 PID gains"(w3041) -> ()
        n1359 = call <vilib>:"Add State(s) to Queue__JKI_lib_State_Machine.vi"("State(s) in (\"\")"=w3049) -> ("States Out"=w3048:string)  [unwired: 14 in]
      }
      frame "---------- Template ----------" {
        # "Template Separator\n(You can make a copy of, or modify, this frame)"
        n1360 = call <vilib>:"Add State(s) to Queue__JKI_lib_State_Machine.vi"("State(s) in (\"\")"=w3054) -> ("States Out"=w3053:string)  [unwired: 14 in]
      }
    }
  }
  n1361 = while {
    tunnel: w39 -> [w3087]
    shift-right: [w3069] -> _
    shift-left: w26 -> [w3068]
    tunnel: w36 -> [w3080]
    tunnel: [w3078] -> w35
    shift-right: [w3077] -> _
    shift-left: w23 -> [w3076]
    i -> [w3072]
    stop <- w3071 stop-if-true
    # "stop on error"
    # "Gain adjustment and Data processing"
    n1362 = Wait on Notification(notifier=w3087, ignore previous (F)=TRUE) -> (notification=w3085:cluster{"idx":i32, "CH1&2":dbl[][]}, error out=w3062:errorcluster)  [unwired: 2 in, 2 out]
    n1363 = call <vilib>:"High Resolution Relative Seconds.vi"() -> ("relative seconds"=w3077:dbl)
    n1364 = flat-sequence {
      tunnel: [w3223] -> w3056
      tunnel: w3062 -> [_]
      frame #0 {
        # "make sure it is read after data arrive"
        n1365 = local read "Auto gain"() -> (w3223:bool)
      }
    }
    n1366 = Subtract(x=w3077, y=w3076) -> (x-y=w3075:dbl)
    n1367 = Unbundle(w3085) -> ("CH1&2"=w3067:dbl[][])  [unwired: 1 out]
    n1368 = call "AvgArrayTimeCritical.vi"("2D array"=w3067) -> ("1D Avg"=w3066:dbl[])  [unwired: 10 in]
    n1369 = Multiply(x=w3075, y=1000.0) -> (x*y=→"processing loop timing(ms)":dbl)
    n1370 = Array Max & Min(array=w3066) -> (max value=w3059:dbl)  [unwired: 3 out]
    n1371 = local read "Channel"() -> (w3055:enum32{"Ch1", "Ch2", "Ch3", "Ch4"})
    n1372 = case shown="True" w3056 {
      tunnel: [w3092 w3124] -> w3063
      tunnel: w3062 -> [w3093 w3123]
      tunnel: [w3093 w3122] -> w3061
      tunnel: "V target(1.0)" -> [_ w3121]
      tunnel: w3059 -> [_ w3120]
      tunnel: [w3088 w3118] -> w3058
      tunnel: [w3089 w3117] -> w3057
      tunnel: w3055 -> [w3091 w3116]
      frame False {
        n1373 = case shown="\"Ch4\"" w3091 {
          tunnel: [w3096 w3098 w3100 w3102] -> w3092
          tunnel: [enum16{"Ch1", "Ch2", "Ch3"}."Ch1" ("Channel") enum16{"Ch1", "Ch2", "Ch3"}."Ch2" ("Channel") enum16{"Ch1", "Ch2", "Ch3"}."Ch3" ("Channel") enum16{"Ch1", "Ch2", "Ch3", "Ch4"}."Ch4" ("Channel")] -> w3090
          frame "Ch1", Default {
            n1374 = global read "GlobalVariables.vi" "Ch1 LJ pin"() -> (w3096:string)
          }
          frame "Ch2" {
            n1375 = global read "GlobalVariables.vi" "Ch2 LJ pin"() -> (w3098:string)
          }
          frame "Ch3" {
            n1376 = global read "GlobalVariables.vi" "Ch3 LJ pin"() -> (w3100:string)
          }
          frame "Ch4" {
            n1377 = global read "GlobalVariables.vi" "Ch4 LJ pin"() -> (w3102:string)
          }
        }
        n1378 = call "V1FGV.vi"("action (write)"=enum16{"write", "read"}."read" ("action")) -> ("V1 out"=w3089:dbl)  [unwired: 9 in, 1 out]
        n1379 = call "CtrlVtoGain.vi"("CtrlV(V)"=w3089, "Channel"=w3090) -> ("Gain"=w3088:dbl)  [unwired: 8 in, 1 out]
      }
      frame True {
        n1380 = case shown="\"Ch4\"" w3116 {
          tunnel: [w3149 w3173 w3197 w3221] -> w3124
          tunnel: w3123 -> [w3148 w3172 w3196 w3220]
          tunnel: [w3148 w3172 w3196 w3220] -> w3122
          tunnel: [w3147 w3171 w3195 w3219] -> _
          tunnel: w3121 -> [w3136 w3160 w3184 w3209]
          tunnel: w3120 -> [w3135 w3159 w3183 w3208]
          tunnel: "autotune? (F)" -> [w3142 w3166 w3190 w3215]
          tunnel: [w3146 w3170 w3194 w3218] -> w3118
          tunnel: [w3128 w3151 w3175 w3200] -> w3117
          tunnel: "PID dt (s)" -> [w3138 w3162 w3186 w3211]
          tunnel: "autotuning parameters" -> [w3134 w3158 w3182 w3207]
          tunnel: [w3137 w3161 w3185 w3210] -> w3114
          tunnel: "Accept?" -> [w3133 w3157 w3181 w3206]
          tunnel: "Gain(Log)" -> [w3132 w3156 w3180 w3205]
          tunnel: [w3131 w3155 w3179 w3204] -> w3110
          tunnel: [w3131 w3155 w3179 w3204] -> w3109
          tunnel: [w3130 w3154 w3178 w3203] -> w3108
          tunnel: [w3125 w3153 w3177 w3202] -> w3107
          tunnel: [w3129 w3152 w3176 w3201] -> w3106
          tunnel: [w3128 w3151 w3175 w3200] -> w3105
          tunnel: "gamma" -> [w3127 _ _ _]
          tunnel: "alpha" -> [w3126 _ _ _]
          frame "Ch1", Default {
            w3147 = enum16{"Ch1", "Ch2", "Ch3"}."Ch1" ("Enum")
            n1381 = global read "GlobalVariables.vi" "Ch1GainLim(Log)"() -> (w3140:cluster{"GainMax":dbl, "GainMin":dbl})
            n1382 = call-poly <vilib>:"PID Online Autotuning.vi"("setpoint"=w3136, "manipulated variable"=w3132, "autotuning parameters"=w3134, "process variable"=w3135, "PID gains in"="Ch1 PID gains", "dt (s)"=w3138, "autotune? (F)"=w3142) -> ("setpoint out"=w3144:dbl, "process variable out"=w3143:dbl, "tuning completed?"=w3129:bool, "PID gains out"=w3141:T6, "tuned PID gains"=w3125:T6)  [unwired: 4 in]
            n1383 = case shown="True" w3133 {
              tunnel: w3125 -> [_ w3150]
              frame False {
              }
              frame True {
                n1384 = local write "Ch1 PID gains"(w3150) -> ()
              }
            }
            n1385 = call-poly <vilib>:"PID Advanced.vi"("setpoint"=w3144, "output range"=w3140, "auto? (T)"=TRUE, "process variable"=w3143, "gamma"=w3127, "alpha"=w3126, "PID gains"=w3141, "dt (s)"=w3138) -> ("output"=w3131:dbl, "dt out (s)"=w3137:dbl)  [unwired: 6 in]
            n1386 = Power Of 10(x=w3131) -> (10^x=w3146:dbl)
            n1387 = call "GainToCtrlV.vi"("Gain"=w3146, "Channel"=w3147) -> ("CtrlV"=w3128:dbl)  [unwired: 8 in, 1 out]
            n1388 = global read "GlobalVariables.vi" "Ch1 LJ pin"() -> (w3149:string)
            n1389 = Bundle("V target(1.0)"=w3136, w3135) -> (w3130:cluster{"V target(1.0)":dbl, dbl})  [unwired: 1 in]
          }
          frame "Ch2" {
            w3171 = enum16{"Ch1", "Ch2", "Ch3"}."Ch2" ("Enum")
            n1390 = global read "GlobalVariables.vi" "Ch2GainLim(Log)"() -> (w3164:cluster{"GainMax":dbl, "GainMin":dbl})
            n1391 = call-poly <vilib>:"PID Online Autotuning.vi"("setpoint"=w3160, "manipulated variable"=w3156, "autotuning parameters"=w3158, "process variable"=w3159, "PID gains in"="Ch2 PID gains", "dt (s)"=w3162, "autotune? (F)"=w3166) -> ("setpoint out"=w3168:dbl, "process variable out"=w3167:dbl, "tuning completed?"=w3152:bool, "PID gains out"=w3165:T6, "tuned PID gains"=w3153:T6)  [unwired: 4 in]
            n1392 = case shown="True" w3157 {
              tunnel: w3153 -> [_ w3174]
              frame False {
              }
              frame True {
                n1393 = local write "Ch2 PID gains"(w3174) -> ()
              }
            }
            n1394 = call-poly <vilib>:"PID Advanced.vi"("setpoint"=w3168, "output range"=w3164, "auto? (T)"=TRUE, "process variable"=w3167, "PID gains"=w3165, "dt (s)"=w3162) -> ("output"=w3155:dbl, "dt out (s)"=w3161:dbl)  [unwired: 8 in]
            n1395 = Power Of 10(x=w3155) -> (10^x=w3170:dbl)
            n1396 = call "GainToCtrlV.vi"("Gain"=w3170, "Channel"=w3171) -> ("CtrlV"=w3151:dbl)  [unwired: 8 in, 1 out]
            n1397 = global read "GlobalVariables.vi" "Ch2 LJ pin"() -> (w3173:string)
            n1398 = Bundle("V target(1.0)"=w3160, w3159) -> (w3154:cluster{"V target(1.0)":dbl, dbl})  [unwired: 1 in]
          }
          frame "Ch3" {
            w3195 = enum16{"Ch1", "Ch2", "Ch3"}."Ch3" ("Enum")
            n1399 = global read "GlobalVariables.vi" "Ch3GainLim(Log)"() -> (w3188:cluster{"GainMax":dbl, "GainMin":dbl})
            n1400 = call-poly <vilib>:"PID Online Autotuning.vi"("setpoint"=w3184, "manipulated variable"=w3180, "autotuning parameters"=w3182, "process variable"=w3183, "PID gains in"="Ch3 PID gains", "dt (s)"=w3186, "autotune? (F)"=w3190) -> ("setpoint out"=w3192:dbl, "process variable out"=w3191:dbl, "tuning completed?"=w3176:bool, "PID gains out"=w3189:T6, "tuned PID gains"=w3177:T6)  [unwired: 4 in]
            n1401 = case shown="True" w3181 {
              tunnel: w3177 -> [_ w3198]
              frame False {
              }
              frame True {
                n1402 = local write "Ch3 PID gains"(w3198) -> ()
              }
            }
            n1403 = call-poly <vilib>:"PID Advanced.vi"("setpoint"=w3192, "output range"=w3188, "auto? (T)"=TRUE, "process variable"=w3191, "PID gains"=w3189, "dt (s)"=w3186) -> ("output"=w3179:dbl, "dt out (s)"=w3185:dbl)  [unwired: 8 in]
            n1404 = Power Of 10(x=w3179) -> (10^x=w3194:dbl)
            n1405 = call "GainToCtrlV.vi"("Gain"=w3194, "Channel"=w3195) -> ("CtrlV"=w3175:dbl)  [unwired: 8 in, 1 out]
            n1406 = global read "GlobalVariables.vi" "Ch3 LJ pin"() -> (w3197:string)
            n1407 = Bundle("V target(1.0)"=w3184, w3183) -> (w3178:cluster{"V target(1.0)":dbl, dbl})  [unwired: 1 in]
          }
          frame "Ch4" {
            w3219 = enum16{"Ch1", "Ch2", "Ch3"}."Ch3" ("Enum")
            n1408 = global read "GlobalVariables.vi" "Ch4GainLim(Log)"() -> (w3213:cluster{"GainMax":dbl, "GainMin":dbl})
            n1409 = call-poly <vilib>:"PID Online Autotuning.vi"("setpoint"=w3209, "manipulated variable"=w3205, "autotuning parameters"=w3207, "process variable"=w3208, "PID gains in"="Ch4 PID gains", "dt (s)"=w3211, "autotune? (F)"=w3215) -> ("setpoint out"=w3217:dbl, "process variable out"=w3216:dbl, "tuning completed?"=w3201:bool, "PID gains out"=w3214:T6, "tuned PID gains"=w3202:T6)  [unwired: 4 in]
            n1410 = case shown="True" w3206 {
              tunnel: w3202 -> [_ w3222]
              frame False {
              }
              frame True {
                n1411 = local write "Ch4 PID gains"(w3222) -> ()
              }
            }
            n1412 = call-poly <vilib>:"PID Advanced.vi"("setpoint"=w3217, "output range"=w3213, "auto? (T)"=TRUE, "process variable"=w3216, "PID gains"=w3214, "dt (s)"=w3211) -> ("output"=w3204:dbl, "dt out (s)"=w3210:dbl)  [unwired: 8 in]
            n1413 = Power Of 10(x=w3204) -> (10^x=w3218:dbl)
            n1414 = call "GainToCtrlV.vi"("Gain"=w3218, "Channel"=w3219) -> ("CtrlV"=w3200:dbl)  [unwired: 8 in, 1 out]
            n1415 = global read "GlobalVariables.vi" "Ch4 LJ pin"() -> (w3221:string)
            n1416 = Bundle("V target(1.0)"=w3209, w3208) -> (w3203:cluster{"V target(1.0)":dbl, dbl})  [unwired: 1 in]
          }
        }
        "dt out (s)" <- w3114
        "Gain(Log10)" <- w3109
        "Targer and Max" <- w3108
        "tuned PID gains" <- w3107
        "Completed?" <- w3106
        n1417 = local write "Ctrl V"(w3105) -> ()
        n1418 = local write "Gain(Log)"(w3110) -> ()
        n1419 = call "V1FGV.vi"("V1 in"=w3105) -> ()  [unwired: 9 in, 2 out]
      }
    }
    n1420 = local write "GainIndicator"(w3058) -> ()
    n1421 = call "LabJack_FGV.vi"("Operation(Read)"=enum16{"Write", "Read"}."Read" ("Operation"), "error in (no error)"=w3061) -> ("error out"=w3084:errorcluster, "Read data"=w3083:i32)  [unwired: 8 in]
    n1422 = Not Equal?(x=w3057, y=w3068) -> (x != y?=w3070:bool)
    n1423 = case shown="True" w3070 {
      tunnel: w3084 -> [w3225 w3226]
      tunnel: w3083 -> [_ w3230]
      tunnel: [w3225 w3229] -> w3064
      tunnel: w3057 -> [w3224 w3227]
      tunnel: [w3224 w3227] -> w3069
      tunnel: w3063 -> [_ w3228]
      frame False {
      }
      frame True {
        n1424 = call "LJM_eWriteName.vi"("Handle In"=w3230, "Name"=w3228, "Value"=w3227, "error in"=w3226) -> ("error out"=w3229:errorcluster)  [unwired: 10 in, 1 out]
      }
    }
    n1425 = Build Array(w3066) -> (w3065:dbl[][])
    n1426 = Bundle(w3065) -> (w3081:cluster{dbl[][]})  [unwired: 1 in]
    n1427 = Send Notification(notification=w3081, notifier=w3080) -> (notifier out=w3078:refnum<notifier>, error out=w3079:errorcluster)  [unwired: 1 in]
    n1428 = Merge Errors(w3064, w3079) -> (w3071:errorcluster)
    "processing Error Out" <- w3071
    "processing loop" <- w3072
  }
  n1429 = while {
    tunnel: w54 -> [w3243]
    tunnel: w44 -> [w3242]
    tunnel: [w3241] -> w52
    tunnel: w39 -> [w3240]
    tunnel: [w3239] -> w48
    tunnel: w27 -> [w3237]
    tunnel: w32 -> [w3236]
    tunnel: w24 -> [w3231]
    stop <- w3234 stop-if-true
    # "acquire data and send it to processing loop"
    # "Data Aquisition Loop"
    n1430 = event shown="[1] <Start digitizer>: User Event" {
      selector: w3242 -> [_ _]
      dyn-events: [_ _] -> w3241
      timeout: 20 -> [_ _]
      tunnel: w3243 -> [w3249 w3261]
      tunnel: [w3244 _] -> w3234
      tunnel: w3240 -> [w3248 w3267]
      tunnel: [w3248 w3266] -> w3239
      tunnel: w3237 -> [_ w3265]
      tunnel: w3236 -> [w3247 w3260]
      tunnel: w3231 -> [_ w3258]
      event Timeout {
        # "use queue to stop data loop\nwhen queue ref is released, error will stop this loop"
        n1431 = event-data() -> ()  [unwired: 1 in, 3 out]
        n1432 = Get Queue Status(queue=w3249) -> (error out=w3246:errorcluster)  [unwired: 2 in, 7 out]
        n1433 = Get Queue Status(queue=w3247) -> (error out=w3245:errorcluster)  [unwired: 2 in, 7 out]
        n1434 = Merge Errors(w3246, w3245) -> (w3244:errorcluster)
      }
      event User Event {
        n1435 = event-data() -> ()  [unwired: 1 in, 4 out]
        n1436 = local read "Channel"() -> (w3253:enum32{"Ch1", "Ch2", "Ch3", "Ch4"})
        n1437 = case shown="\"Ch4\"" w3253 {
          tunnel: [w3276 w3284 w3287 w3295] -> w3264
          tunnel: [w3274 w3282 w3289 w3297] -> w3257
          tunnel: [w3273 w3281 w3292 w3300] -> w3256
          tunnel: [w3272 w3280 w3291 w3299] -> w3255
          tunnel: [w3271 w3279 w3290 w3298] -> w3254
          tunnel: [w3270 w3278 w3286 w3294] -> w3252
          frame "Ch1", Default {
            w3270 = "0" ("Active Channel")
            w3277 = enum16{"Write", "Read"}."Read" ("Operation")
            n1438 = call "Digitizer1_FGV.vi"("Operation (Read)"=w3277) -> ("Read data"=w3275:refnum<k15>)  [unwired: 9 in, 1 out]
            n1439 = call "Digitizer2_FGV.vi"("Operation (Read)"=w3277) -> ("Read data"=w3276:refnum<k15>)  [unwired: 9 in, 1 out]
            n1440 = property on="Property Node" class="niScope"(reference=w3275, "Active Channel"=w3270) -> (reference out=w3274:refnum<k15>, error out=w3272:errorcluster, "Vertical Range"=w3271:dbl, "Vertical Offset"=w3273:dbl)  [unwired: 1 in]
          }
          frame "Ch2" {
            w3278 = "1" ("Active Channel")
            w3285 = enum16{"Write", "Read"}."Read" ("Operation")
            n1441 = call "Digitizer1_FGV.vi"("Operation (Read)"=w3285) -> ("Read data"=w3283:refnum<k15>)  [unwired: 9 in, 1 out]
            n1442 = call "Digitizer2_FGV.vi"("Operation (Read)"=w3285) -> ("Read data"=w3284:refnum<k15>)  [unwired: 9 in, 1 out]
            n1443 = property on="Property Node" class="niScope"(reference=w3283, "Active Channel"=w3278) -> (reference out=w3282:refnum<k15>, error out=w3280:errorcluster, "Vertical Range"=w3279:dbl, "Vertical Offset"=w3281:dbl)  [unwired: 1 in]
          }
          frame "Ch3" {
            w3286 = "0" ("Active Channel")
            w3293 = enum16{"Write", "Read"}."Read" ("Operation")
            n1444 = call "Digitizer2_FGV.vi"("Operation (Read)"=w3293) -> ("Read data"=w3288:refnum<k15>)  [unwired: 9 in, 1 out]
            n1445 = call "Digitizer1_FGV.vi"("Operation (Read)"=w3293) -> ("Read data"=w3289:refnum<k15>)  [unwired: 9 in, 1 out]
            n1446 = property on="Property Node" class="niScope"(reference=w3288, "Active Channel"=w3286) -> (reference out=w3287:refnum<k15>, error out=w3291:errorcluster, "Vertical Range"=w3290:dbl, "Vertical Offset"=w3292:dbl)  [unwired: 1 in]
          }
          frame "Ch4" {
            w3294 = "1" ("Active Channel")
            w3301 = enum16{"Write", "Read"}."Read" ("Operation")
            n1447 = call "Digitizer2_FGV.vi"("Operation (Read)"=w3301) -> ("Read data"=w3296:refnum<k15>)  [unwired: 9 in, 1 out]
            n1448 = call "Digitizer1_FGV.vi"("Operation (Read)"=w3301) -> ("Read data"=w3297:refnum<k15>)  [unwired: 9 in, 1 out]
            n1449 = property on="Property Node" class="niScope"(reference=w3296, "Active Channel"=w3294) -> (reference out=w3295:refnum<k15>, error out=w3299:errorcluster, "Vertical Range"=w3298:dbl, "Vertical Offset"=w3300:dbl)  [unwired: 1 in]
          }
        }
        n1450 = local read "Task"() -> (w3250:enum32{"iRFAndGain", "Alignment"})
        n1451 = case shown="\"Alignment\"" w3250 {
          tunnel: [0.25 ("timeout") 0.75 ("timeout")] -> w3251
          frame "iRFAndGain", Default {
          }
          frame "Alignment" {
          }
        }
        n1452 = call "FLImDAQ_FGV.vi"() -> ("Read data"=w3263:T4)  [unwired: 10 in, 1 out]
        n1453 = Unbundle By Name(w3263) -> ("Waveform to Avg"=w3262:i16)
        n1454 = while {
          tunnel: w3267 -> [w3340]
          tunnel: [w3339] -> w3266
          tunnel: w3264 -> [w3337]
          tunnel: w3257 -> [w3336]
          tunnel: w3265 -> [w3335]
          shift-right: [w3319] -> _
          shift-left: u32 0 ("millisecond timer value") -> [w3331]
          tunnel: w3262 -> [w3329]
          tunnel: w3261 -> [_]
          tunnel: w3260 -> [w3327]
          tunnel: w3258 -> [w3324]
          tunnel: w3254 -> [w3320]
          tunnel: w3256 -> [w3321]
          tunnel: w3255 -> [w3314]
          tunnel: w3253 -> [w3313]
          tunnel: w3252 -> [w3312]
          tunnel: w3251 -> [w3303]
          i -> [w3328]
          stop <- w3317 stop-if-true
          # "enqueue data"
          # "send data for processing"
          n1455 = Tick Count (ms)() -> (millisecond timer value=w3319:u32)
          n1456 = Subtract(x=w3319, y=w3331) -> (x-y=→"Aquisition loop timing(ms)":u32)
          n1457 = Multiply(x=w3329, y=w3328) -> (x*y=w3322:i32)
          "Fetch Record #" <- w3322
          n1458 = property on="Property Node" class="niScope"(reference=w3336, error in=w3314, "Fetch Record Number"=w3322) -> (reference out=w3342:refnum<k15>, error out=w3341:errorcluster, "Records Done"=w3306:i32)
          "Fetch:Records Done" <- w3306
          n1459 = Subtract(x=w3306, y=w3322) -> (x-y=→"Record Backlog":i32)
          n1460 = call-poly <instrlib>:"niScope Fetch (poly).vi"("timeout"=w3303, "error in"=w3341, "channels"=w3312, "instrument handle"=w3342) -> ("error out"=w3318:errorcluster, "wfm"=w3311:i16[][])  [unwired: 4 in, 2 out]
          n1461 = case shown="\"Ch3\"" w3313 {
            tunnel: w3337 -> [_ w3358 w3368]
            tunnel: [w3349 w3357 w3367] -> w3332
            tunnel: w3322 -> [_ w3356 w3366]
            tunnel: w3318 -> [w3350 w3355 w3365]
            tunnel: [w3350 w3354 w3364] -> w3308
            tunnel: w3311 -> [w3349 _ _]
            tunnel: w3303 -> [_ w3352 w3362]
            tunnel: [0 ("Records Done") w3351 w3361] -> w3302
            frame "Ch1", "Ch2", Default {
            }
            frame "Ch3" {
              n1462 = property on="Property Node" class="niScope"(reference=w3358, error in=w3355, "Fetch Record Number"=w3356) -> (reference out=w3360:refnum<k15>, error out=w3353:errorcluster, "Records Done"=w3351:i32)
              n1463 = call-poly <instrlib>:"niScope Fetch (poly).vi"("timeout"=w3352, "error in"=w3353, "channels"="0", "instrument handle"=w3360) -> ("error out"=w3354:errorcluster, "wfm"=w3357:i16[][])  [unwired: 4 in, 2 out]
            }
            frame "Ch4" {
              n1464 = property on="Property Node" class="niScope"(reference=w3368, error in=w3365, "Fetch Record Number"=w3366) -> (reference out=w3370:refnum<k15>, error out=w3363:errorcluster, "Records Done"=w3361:i32)
              n1465 = call-poly <instrlib>:"niScope Fetch (poly).vi"("timeout"=w3362, "error in"=w3363, "channels"="1", "instrument handle"=w3370) -> ("error out"=w3364:errorcluster, "wfm"=w3367:i16[][])  [unwired: 4 in, 2 out]
            }
          }
          "Fetch:Records Done 2" <- w3302
          n1466 = call "V1FGV.vi"("action (write)"=enum16{"write", "read"}."read" ("action")) -> ("V1 out"=w3305:dbl)  [unwired: 9 in, 1 out]
          n1467 = Enqueue Element(queue=w3324, element=w3305, error in (no error)=w3308) -> (error out=w3323:errorcluster)  [unwired: 1 in, 2 out]
          n1468 = Divide(x=w3332, y=65536) -> (x/y=w3334:dbl[][])
          n1469 = Multiply(x=w3334, y=w3320) -> (x*y=w3333:dbl[][])
          n1470 = Add(x=w3333, y=w3321) -> (x+y=w3309:dbl[][])
          n1471 = Bundle(w3328, w3309) -> (w3307:cluster{i32, dbl[][]})  [unwired: 1 in]
          n1472 = case shown="True" "SaveData?" {
            tunnel: w3327 -> [_ w3347]
            tunnel: [w3343 w3346] -> w3316
            tunnel: w3309 -> [_ w3345]
            tunnel: w3308 -> [w3343 w3344]
            frame False {
            }
            frame True {
              n1473 = Enqueue Element(queue=w3347, element=w3345, error in (no error)=w3344) -> (error out=w3346:errorcluster)  [unwired: 1 in, 2 out]
            }
          }
          n1474 = Send Notification(notification=w3307, notifier=w3340, error in (no error)=w3316) -> (notifier out=w3339:refnum<notifier>, error out=w3315:errorcluster)
          n1475 = Merge Errors(w3323, w3315) -> (w3326:errorcluster)
          n1476 = case shown="Error .." w3326 {
            selector: w3326 -> [w3371 w3372]
            tunnel: w3335 -> [_ w3375]
            tunnel: [w3371 w3372] -> w3317
            frame No Error {
            }
            frame Error {
              # "Send user event to signal aquisition has stoped"
              n1477 = Generate User Event(priority (normal)=usereventprio."high priority", user event=w3375, event data cluster=TRUE ("event data")) -> ()  [unwired: 1 in, 2 out]
            }
          }
          "aquisition loop Error Out" <- w3317
        }
      }
    }
    n1478 = Unbundle By Name(w3234) -> ("status"=w3233:bool)
    n1479 = Not(x=w3233) -> (.not. x?=w3232:bool)
    n1480 = local write "Aq Loop?"(w3232) -> ()
    "Aq Loop?" <- TRUE ("Aq L?")
  }
  n1481 = Close File(refnum=w10, error in=w11) -> (error out=w7:errorcluster)  [unwired: 1 out]
  n1482 = Release Queue(queue=w6, error in (no error)=w7) -> ()  [unwired: 1 in, 3 out]
  n1483 = Unregister For Events(event registration refnum=w30, error in=w40) -> (error out=w41:errorcluster)
  n1484 = Release Notifier(notifier=w35, error in (no error)=w33) -> (error out=w34:errorcluster)  [unwired: 1 in, 2 out]
  n1485 = call <vilib>:"Simple Error Handler.vi"("error in (no error)"=w34) -> ()  [unwired: 4 in, 5 out]
  n1486 = Destroy User Event(user event=w27, error in=w41) -> ()  [unwired: 1 out]
  n1487 = Release Notifier(notifier=w48, error in (no error)=w47) -> (error out=w46:errorcluster)  [unwired: 1 in, 2 out]
  n1488 = Unregister For Events(event registration refnum=w52, error in=w50) -> (error out=w51:errorcluster)
  n1489 = call <vilib>:"Simple Error Handler.vi"("error in (no error)"=w46) -> ()  [unwired: 4 in, 5 out]
  n1490 = Destroy User Event(user event=w42, error in=w51) -> ()  [unwired: 1 out]
